vi "Demo_Main-Administrator.vi"() -> ()   [LabVIEW 2010]
uses:
  ControlCAN/ControlCAN.llb/DevType.ctl
  ControlCAN/ControlCAN.llb/CAN Channel.ctl
  ControlCAN/ControlCAN.llb/InitFlag.ctl
  ControlCAN/ControlCAN.llb/Mode.ctl
  ControlCAN/ControlCAN.llb/Fliter.ctl
  ControlCAN/ControlCAN.llb/VCI_CAN_OBJ.ctl
  ControlCAN/ControlCAN.llb/VCI_INIT_CONFIG.ctl
  ControlCAN/ControlCAN.llb/Return Val.ctl
  ControlCAN/ControlCAN.lvlib
panel:
  in  "下限":dbl format="%#.1f"
  out "零位角":dbl format="%#.6f"
  in  "Zero_R":bool
  in  "Zero_SAVE_W":bool
  in  "ZeroEn_R":bool
  in  "零位En":i8
  out "零位使能":i8
  in  "ZeroEn_W":bool
  in  "设定力矩_R":bool
  in  "设定力矩":dbl format="%#.6f"
  out "设定力矩_回":dbl format="%#.6f"
  in  "设定力矩_W":bool
  in  "PosLimitEn_R":bool
  in  "限位En":i8
  out "限位使能":i8
  in  "PosLimitEn_W":bool
  in  "Servo_Count_R":bool
  in  "伺服频率":u16
  out "伺服频率R":u16
  in  "Servo_Count_W":bool
  in  "Servo_EN_R":bool
  in  "伺服En":i8
  out "伺服使能":i8
  in  "Servo_EN_W":bool
  in  "Gear_R":bool
  in  "Kt_R":bool
  in  "Gear":u16
  out "Gear":dbl format="%#.6f"
  in  "Gear_W":bool
  in  "Kt":dbl format="%#.6f"
  out "Kt回":dbl format="%.4f"
  in  "Kt_W":bool
  in  "下限位R":bool
  out "下限位":dbl format="%#.6f"
  in  "下限位_W":bool
  in  "上限位_R":bool
  in  "上限位":dbl format="%#.6f"
  out "上限位 _回":dbl format="%#.6f"
  in  "上限位W":bool
  out "电压限制_回":dbl
  in  "电压限制_R":bool
  in  "电压限制_W":bool
  in  "电压限制":dbl
  in  "位置环KI_R":bool
  in  "位置环KP_R":bool
  in  "位置环KI":dbl format="%#.6f"
  out "位置环KI_回":dbl format="%#.6f"
  in  "位置环KI_W":bool
  in  "位置环KP":dbl format="%#.6f"
  out "位置环KP_回":dbl format="%#.6f"
  in  "位置环KP_W":bool
  in  "T4":u16
  in  "W4":u16
  in  "W3":u16
  out "W4":u16
  in  "W4_R":bool
  in  "W4_W":bool
  in  "W3_R":bool
  out "W3":u16
  in  "W3_W":bool
  out "W2":u16
  in  "W2_R":bool
  in  "W2_W":bool
  in  "W2":u16
  in  "W1_R":bool
  in  "W1":u16
  out "W1":u16
  in  "W1_W":bool
  in  "T4_R":bool
  out "T4":u16
  in  "T4_W":bool
  out "T3":u16
  out "T2":u16
  in  "T3_R":bool
  in  "T2_R":bool
  in  "T3_W":bool
  in  "T2_W":bool
  in  "T3":u16
  in  "T2":u16
  in  "T1_R":bool
  in  "T1":u16
  out "T1":u16
  in  "T1_W":bool
  in  "W_EN_R":bool
  in  "过载诊断":i8
  out "功率使能":i8
  in  "W_EN_W":bool
  in  "I_EN_R":bool
  in  "Direction_R":bool
  in  "电流诊断":i8
  out "电流使能":i8
  in  "I_EN_W":bool
  in  "方向":u16
  out "方向":i8
  in  "Direction_W":bool
  out "电流限制_回":dbl
  in  "电流限制_R":bool
  in  "电流限制_W":bool
  in  "电流限制":dbl
  in  "速度限制_R":bool
  in  "速度限制":dbl
  out "速度限制_回":dbl
  in  "速度限制_W":bool
  out "编码器线数_回":u16
  in  "编码器线数_R":bool
  in  "编码器线数_W":bool
  in  "线数":u16
  in  "极对数_R":bool
  in  "极对数":u8
  out "极对数_回":u8
  in  "极对数_W":bool
  in  "电机自动校准":string(combo)="0"
  in  "电机校准_W":bool
  in  "对准角_R":bool
  in  "对准角":dbl format="%#.6f"
  out "对准角_回":dbl format="%#.6f"
  in  "对准角_W":bool
  in  "减速度_R":bool
  in  "减速度":dbl format="%#.6f"
  out "减速度_回":dbl format="%#.6f"
  in  "减速度_W":bool
  out "版本号":dbl format="%_3f"
  in  "看门狗周期_R":bool
  in  "看门狗周期":u16
  out "看门狗周期_回":u16
  in  "看门狗周期_W":bool
  in  "看门狗_W":bool
  in  "看门狗":string(combo)="开启"
  in  "监测周期_R":bool
  in  "监测周期":u16
  out "监测周期_回":u16
  in  "监测周期_W":bool
  out "ERRO7":bool
  out "ERRO6":bool
  out "ERRO5":bool
  out "ERRO4":bool
  out "ERRO3":bool
  out "高温":bool
  out "高压":bool
  out "低压":bool
  out "warn7":bool
  out "warn6":bool
  out "warn5":bool
  out "warn4":bool
  out "warn3":bool
  out "高温":bool
  out "warn1":bool
  out "warn0":bool
  out "温度":dbl format="%#.6f"
  out "转速":dbl(graph)
  out "CAN ID":u8 format="%x"
  out "数组":u8[](array[numeric]) format="%x"
  in  "DATA_SAVE_W":bool
  out "CI_K0_回":u16
  out "BI_K0_回":u16
  in  "CI_K0_R":bool
  in  "BI_K0_R":bool
  in  "CI_K0_W":bool
  in  "BI_K0_W":bool
  in  "C电流零偏":u16
  in  "B电流零偏":u16
  in  "AI_K0_R":bool
  in  "A电流零偏":u16
  out "AI_K0_回":u16
  in  "AI_K0_W":bool
  out "Sin":i32
  out "Cosin":i32
  in  "加速度_R":bool
  in  "加速度":dbl format="%#.6f"
  out "加速度_回":dbl format="%#.6f"
  in  "加速度_W":bool
  in  "速度环KI_R":bool
  in  "速度环KP_R":bool
  in  "速度环KI":dbl format="%#.6f"
  out "速度环KI_回":dbl format="%#.6f"
  in  "速度环KI_W":bool
  in  "速度环KP":dbl format="%#.6f"
  out "速度环KP_回":dbl format="%#.6f"
  in  "速度环KP_W":bool
  in  "电流环KI_R":bool
  in  "电流环KP_R":bool
  in  "电流环KI":dbl format="%#.6f"
  out "电流环KI_回":dbl format="%#.6f"
  in  "电流环KI_W":bool
  in  "电流环KP":dbl format="%#.6f"
  out "电流环KP_回":dbl format="%#.6f"
  in  "电流环KP_W":bool
  out "波形图表3":dbl(graph)
  out "波形图表2":dbl(graph)
  out "波形图表1":dbl(graph)
  out "sCnt":u32 caption="处理统计"
  out "模式_回":string(combo)="00"
  in  "模式_R":bool
  in  "设定电流_R":bool
  in  "设定位置_R":bool
  in  "设定速度_R":bool
  in  "存储路径":path
  in  "保存":bool
  out "保存_S":bool
  in  "模式_W":bool
  in  "模式":string(combo)="00"
  in  "设定电流":dbl format="%#.6f"
  out "设定电流_回":dbl format="%#.6f"
  in  "设定电流_W":bool
  in  "设定位置":dbl format="%#.6f"
  out "设定位置_回":dbl format="%#.6f"
  in  "设定位置_W":bool
  in  "设定速度":dbl format="%#.1f"
  out "设定速度_回":dbl format="%#.6f"
  in  "设定速度_W":bool
  in  "监测_W":bool
  in  "监测":string(combo)="30"
  out "电机ID_R":u32
  in  "Clear":bool
  out "Ualfa":dbl format="%#.6f"
  out "Ubate":dbl format="%#.6f"
  out "Uq":dbl format="%#.6f"
  out "Ud":dbl format="%#.6f"
  out "PWM1":u16
  out "PWM2":u16
  out "PWM3":u16
  out "sector":u8
  out "Iqnow":dbl
  out "Idnow":dbl
  out "Ialfa":dbl
  out "Ibeta":dbl
  out "A电流":dbl
  out "C电流":dbl
  out "B电流":dbl
  out "供电电压":dbl
  out "机械角度":dbl format="%.2f"
  out "电气角度":dbl format="%.2f"
  out "转速":dbl
  out "CAN STD_ID":u32 format="%x"
  in  "电机ID":string(combo)="00"
  in  "电机ID_W":bool
  out "RecvCnt":u32 caption="接收统计"
  out "SendCnt":u32 caption="发送统计"
  in  "Format":u8(ring) items=["标准帧", "扩展帧"]
  in  "Type":u8(ring) items=["数据帧", "远程帧"]
  in  "Data":string="00 01 02 03 04 05 06 07"
  in  "ID":u32=291 format="0x%x"
  in  "Send":bool
  in  "RcvEnable":bool=TRUE
  out "Open":bool
  in  "Fliter":T1=1 items=["接收所有类型"=1, "只接收标准帧"=2, "只接收扩展帧"=3]
  in  "kBaudRate":u8(ring)=12 caption="波特率" items=["5k bps"=1, "10k bps"=2, "20k bps"=3, "40k bps"=4, "50k bps"=5, "80k bps"=6, "100k bps"=7, "125k bps"=8, "200k bps"=9, "250k bps"=10, "400k bps"=11, "500k bps"=12, "666k bps"=13, "800k bps"=14, "1000k bps"=15, "33.33k bps"=16, "66.66k bps"=17, "83.33k bps"=18]
  in  "Mode":T2 caption="工作模式" items=["正常工作", "仅侦听模式", "自测模式（环回）"]
  in  "InitFlag":T3 caption="初始化参数" items=["使用Flash参数", "使用界面设置参数"]
  in  "AccMask":u32=4294967295 caption="接收屏蔽码" format="%08x"
  in  "AccCode":u32 caption="接收过滤码" format="%08x"
  in  "Close":bool
  in  "Open":bool
  in  "Channel":T4 caption="CAN通道" items=["通道1", "通道2"]
  in  "DevType":T5=3 caption="设备类型" items=["USB-CAN"=2, "USB-CAN2"=3]
  # "发送指令帧包"
  # "CAN\n  ID"
  # "DATA"
  # "DATA"
  # "DATA"
  # "0"
  # "1"
  # "7"
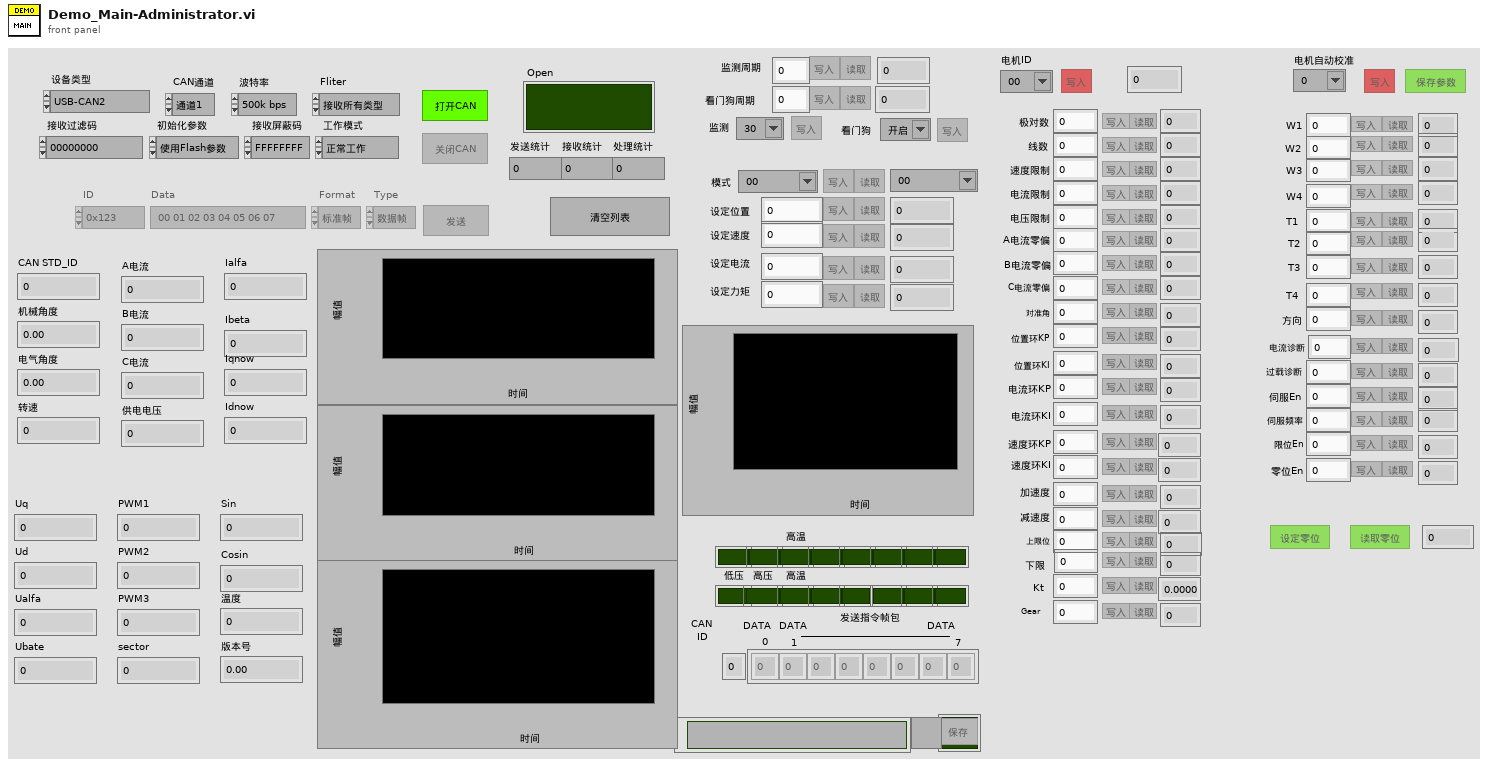
[diagram p1: front panel]
types:
  T1 = typedef "ControlCAN.lvlib/Fliter.ctl" = u8
  T2 = typedef "ControlCAN.lvlib/Mode.ctl" = u8
  T3 = typedef "ControlCAN.lvlib/InitFlag.ctl" = u32
  T4 = typedef "ControlCAN.lvlib/CAN Channel.ctl" = u32
  T5 = typedef "ControlCAN.lvlib/DevType.ctl" = u32
  T6 = typedef "ControlCAN.lvlib/VCI_CAN_OBJ.ctl" = cluster{"ID":u32, "TimeStamp":u32, "TimeFlag":u8, "SendType":u8, "RemoteFlag":u8, "ExternFlag":u8, "DataLen":u8, "Data":u8[], "Reserved":u8[]}
  T7 = cluster{"Type":enum16{"接收", "发送"}, "Channel":T4, "Time":timestamp, "VCI_CAN_OBJ":T6}[]
  T8 = typedef "ControlCAN.lvlib/VCI_INIT_CONFIG.ctl" = cluster{"AccCode":u32, "AccMask":u32, "InitFlag":T3, "Fliter":T1, "Timing0":u8, "Timing1":u8, "Mode":T2}
  T9 = cluster{"DevType":T5, "DevIndex":u32, "CanIndex":T4, "VCI_INIT_CONFIG":T8}
  T10 = typedef "ControlCAN.lvlib/Return Val.ctl" = i32
  T11 = enum16{"open", "replace", "create", "open or create", "replace or create", "replace or create with confirmation"}
  T12 = cluster{"[0]":cluster{"Type":enum16{"接收", "发送"}, "Channel":T4, "Time":timestamp, "VCI_CAN_OBJ":T6}}
  T13 = cluster{"Type":enum16{"接收", "发送"}, "Channel":T4, "Time":timestamp, "VCI_CAN_OBJ":T6}
  T14 = cluster{"Data[0]":u8, "Data[1]":u8, "Data[2]":u8, "Data[3]":u8, "Data[4]":u8, "Data[5]":u8, "Data[6]":u8, "Data[7]":u8}
  T15 = cluster{"Boolean array[0]":bool, "Boolean array[1]":bool, "Boolean array[2]":bool, "Boolean array[3]":bool, "Boolean array[4]":bool, "Boolean array[5]":bool, "Boolean array[6]":bool, "Boolean array[7]":bool}
  T16 = enum32{"invalid app kind", "Development System", "Run Time System", "Student Edition", "Embedded LabVIEW", "Evaluation", "Custom"}
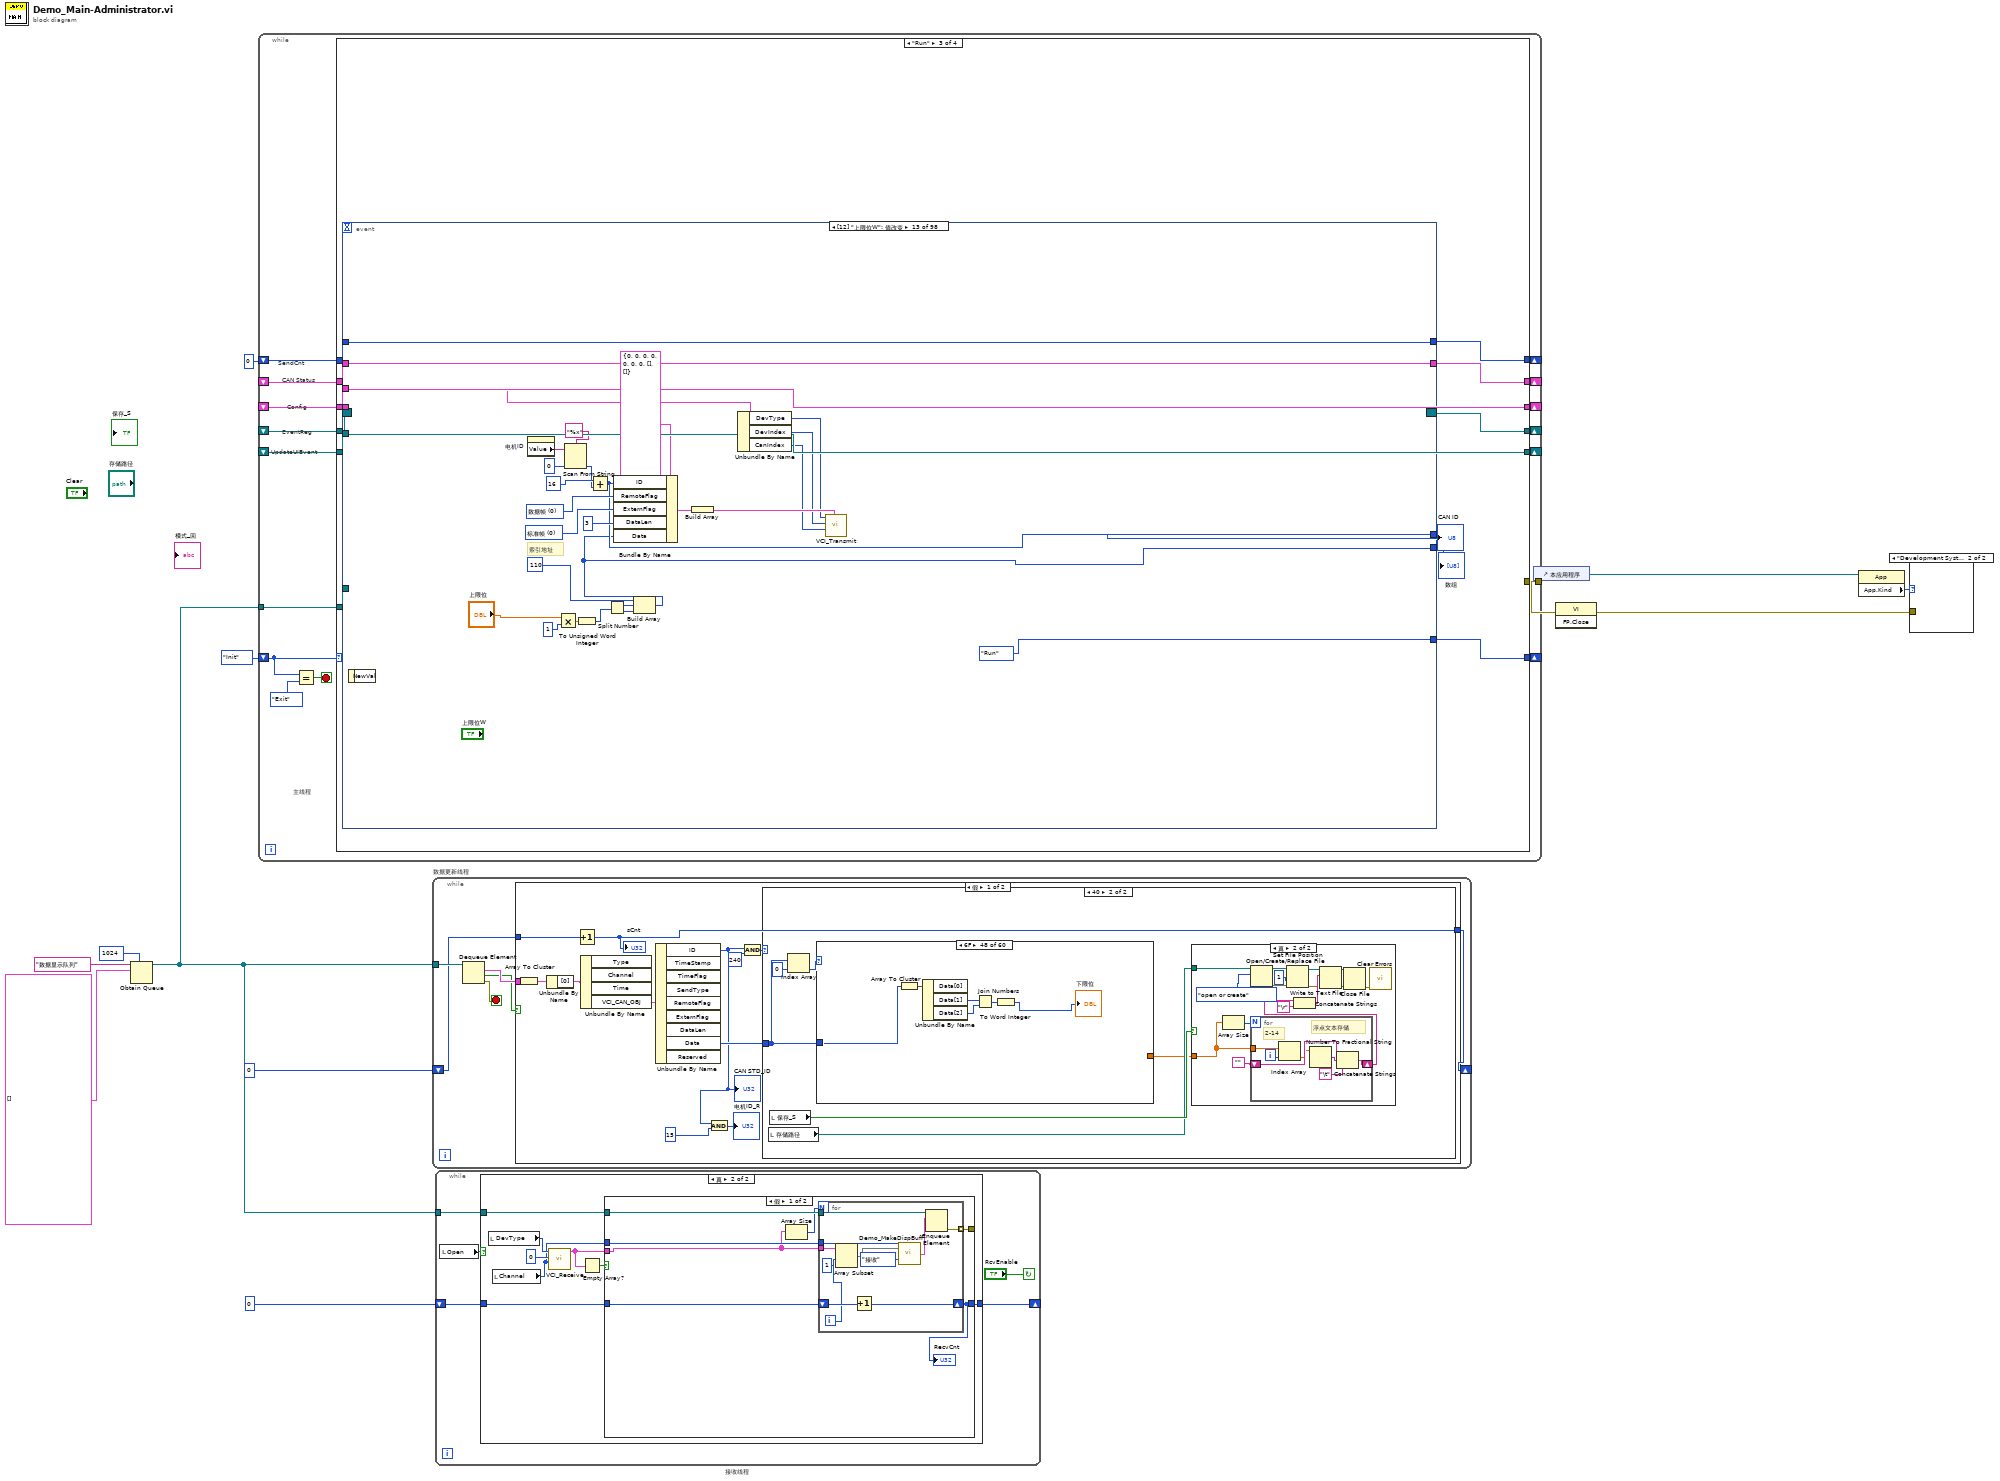
[diagram p0: block diagram]
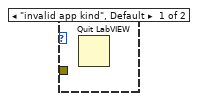
[diagram p2: hidden frame]
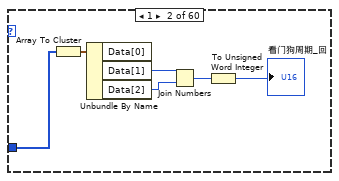
[diagram p6: hidden frame]
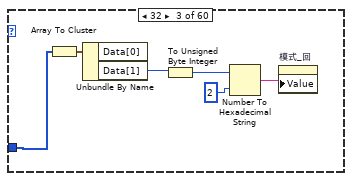
[diagram p7: hidden frame]
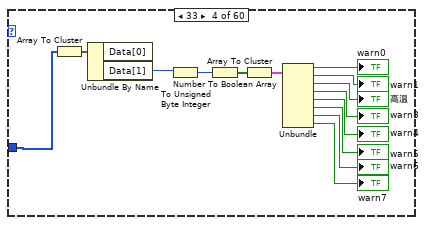
[diagram p8: hidden frame]
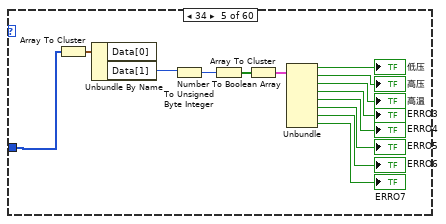
[diagram p9: hidden frame]
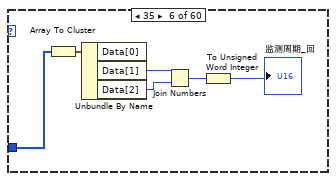
[diagram p10: hidden frame]
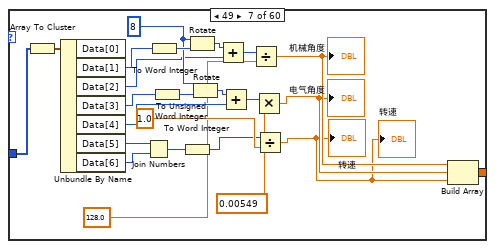
[diagram p11: hidden frame]
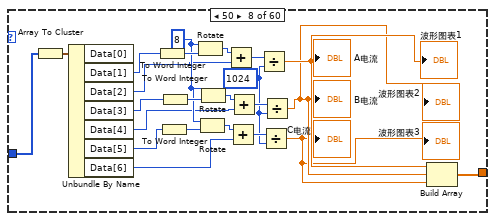
[diagram p12: hidden frame]
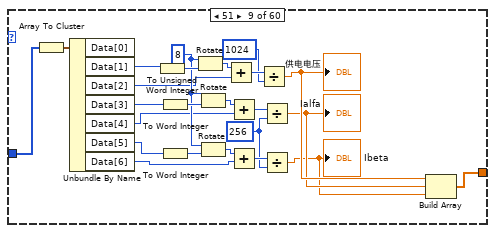
[diagram p13: hidden frame]
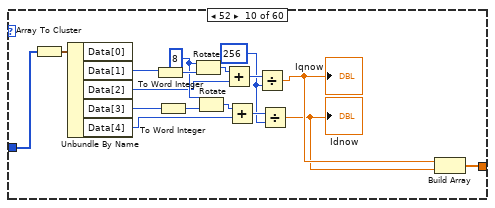
[diagram p14: hidden frame]
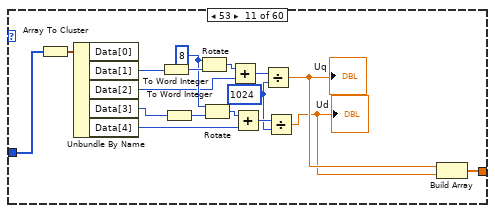
[diagram p15: hidden frame]
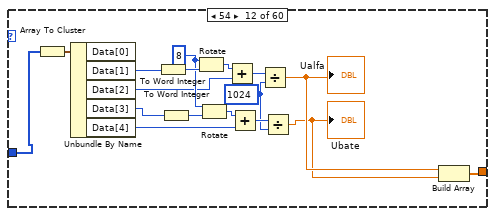
[diagram p16: hidden frame]
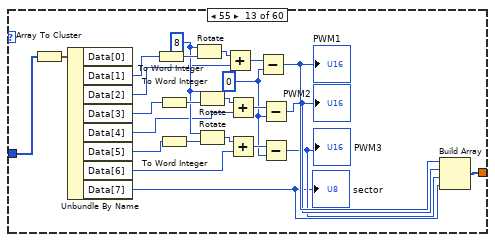
[diagram p17: hidden frame]
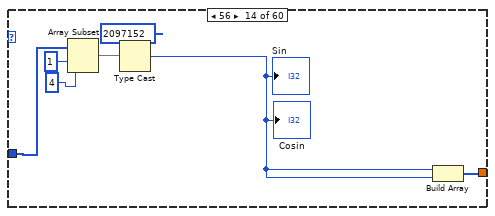
[diagram p18: hidden frame]
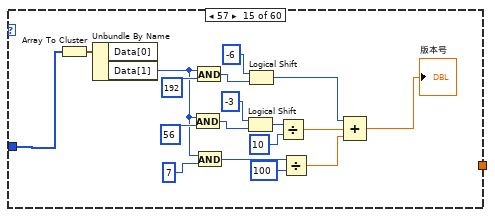
[diagram p19: hidden frame]
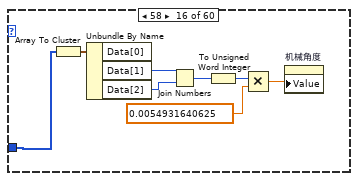
[diagram p20: hidden frame]
diagram:
  n1 = Obtain Queue(max queue size (-1, unlimited)=1024, name (unnamed)="数据显示队列" ("名称（未命名）"), element data type=T7 []) -> (queue out=w9:refnum<queue>)  [unwired: 2 in, 2 out]
  n2 = while "主线程" {
    shift-right: [w24] -> _
    shift-left: enum16{"Init", "Wait", "Run", "Exit"}."Init" -> [w27]
    shift-right: [w25] -> _
    shift-left: _ -> [w26]
    shift-right: [w23] -> _
    shift-left: _ -> [w22]
    tunnel: w9 -> [w21]
    shift-right: [w19] -> _
    shift-left: _ -> [w18]
    shift-right: [w17] -> _
    shift-left: _ -> [w16]
    shift-right: [w14] -> _
    shift-left: u32 0 -> [w15]
    tunnel: [w13] -> w4
    stop <- w28 stop-if-true
    # "CAN Status"
    # "Config"
    # "EventReg"
    # "UpdateUIEvent"
    # "SendCnt"
    n3 = Equal?(x=w27, y=enum16{"Init", "Wait", "Run", "Exit"}."Exit") -> (x = y?=w28:bool)
    n4 = case shown="\"Run\"" w27 {
      tunnel: w26 -> [_ w57 w158 w2353]
      tunnel: [w48 w56 w157 w2353] -> w25
      tunnel: [enum16{"Init", "Wait", "Run", "Exit"}."Wait" w53 w160 enum16{"Init", "Wait", "Run", "Exit"}."Exit"] -> w24
      tunnel: [w44 w54 w149 w2351] -> w23
      tunnel: w22 -> [_ w55 w149 w2351]
      tunnel: w21 -> [_ w52 w159 w2357]
      tunnel: [w36 w51 w155 w2356] -> w19
      tunnel: w18 -> [_ w51 w156 w2356]
      tunnel: [w35 w50 w154 w2354] -> w17
      tunnel: w16 -> [_ w50 w154 w2354]
      tunnel: w15 -> [w33 w49 w153 w2349]
      tunnel: [w33 w49 w152 w2349] -> w14
      tunnel: [_ _ _ errorcluster {"status"=FALSE, "code"=0, "source"=""} ("error constant")] -> w13
      frame "Init", Default {
        w37 = cluster{"CANOpen":bool} {"CANOpen"=FALSE}  # UpdateUI
        w47 = T9 {"DevType"=2, "DevIndex"=0, "CanIndex"=0, "VCI_INIT_CONFIG"={"AccCode"=0, "AccMask"=0, "InitFlag"=0, "Fliter"=0, "Timing0"=0, "Timing1"=0, "Mode"=0}}  # Config
        w48 = cluster{"Open":bool, "SendCnt":u32} {"Open"=FALSE, "SendCnt"=0}  # CAN Status
        n5 = property class="VI"("Front Panel.Closeable"=TRUE ("前面板窗口:可关闭")) -> ()  [unwired: 2 in, 2 out]
        n6 = invoke class="VI" method="Default Vals.Reinit All"() -> ()  [unwired: 3 in, 3 out]
        n7 = call "Demo_GetT0T1.vi"("kBaudRate"="kBaudRate") -> ("Timing0"=w30:u8, "Timing1"=w29:u8)
        n8 = Bundle By Name(cluster=w47, "DevType"="DevType", "CanIndex"="Channel", "VCI_INIT_CONFIG.AccCode"="AccCode", "VCI_INIT_CONFIG.AccMask"="AccMask", "VCI_INIT_CONFIG.InitFlag"="InitFlag", "VCI_INIT_CONFIG.Fliter"="Fliter", "VCI_INIT_CONFIG.Timing0"=w30, "VCI_INIT_CONFIG.Timing1"=w29, "VCI_INIT_CONFIG.Mode"="Mode") -> (w44:T9)
        n9 = local write "RcvEnable"(TRUE ("RcvEnable")) -> ()
        n10 = Create User Event(user event datatype=w37) -> (user event=w35:refnum<user-event>)  [unwired: 1 in, 1 out]
        n11 = register-events(w35) -> (reference out=w36:refnum<event-registration>)  [unwired: 2 in, 1 out]
      }
      frame "Wait" {
        n12 = event shown="[1] 前面板关闭？" {
          selector: _ -> [_ _ _ _ _ _ _ _ _ _]
          dyn-events: _ -> [_ _ _ _ _ _ _ _ _ _]
          timeout: _ -> [_ _ _ _ _ _ _ _ _ _]
          tunnel: w57 -> [w61 w101 w111 w116 w121 w126 w131 w136 w143 w148]
          tunnel: [w60 w101 w111 w116 w121 w126 w131 w136 w143 w148] -> w56
          tunnel: w55 -> [w71 w100 w110 w115 w120 w125 w130 w135 w142 w147]
          tunnel: [w71 w100 w109 w113 w118 w123 w128 w133 w141 w145] -> w54
          tunnel: [w62 enum16{"Init", "Wait", "Run", "Exit"}."Exit" enum16{"Init", "Wait", "Run", "Exit"}."Wait" enum16{"Init", "Wait", "Run", "Exit"}."Wait" enum16{"Init", "Wait", "Run", "Exit"}."Wait" enum16{"Init", "Wait", "Run", "Exit"}."Wait" enum16{"Init", "Wait", "Run", "Exit"}."Wait" enum16{"Init", "Wait", "Run", "Exit"}."Wait" enum16{"Init", "Wait", "Run", "Exit"}."Wait" enum16{"Init", "Wait", "Run", "Exit"}."Wait"] -> w53
          tunnel: w52 -> [_ _ _ _ _ _ _ _ _ _]
          tunnel: w50 -> [w59 _ _ _ _ _ _ _ _ _]
          event "Open": Value Change {
            w65 = T10 1 items=["OK"=1, "ERROR1"=0, "ERROR2"=-1] ("y")
            # "打开CAN的步骤：\n1.Open\n2.Init\n3.Start"
            n13 = event-data() -> ()  [unwired: 2 out]
            n14 = Unbundle By Name(w71) -> ("DevType"=w70:T5, "DevIndex"=w69:u32)
            n15 = call "VCI_OpenDevice.vi"("DevIndex"=w69, "DevType"=w70) -> ("error out"=w66:errorcluster, "Return Val"=w68:T10)  [unwired: 2 in, 6 out]
            n16 = Equal?(x=w68, y=w65) -> (x = y?=w67:bool)
            n17 = case shown="真" w67 {
              tunnel: w66 -> [_ w86]
              tunnel: w71 -> [_ w85]
              tunnel: w65 -> [_ w77]
              tunnel: [_ w76] -> w58
              frame False {
              }
              frame True {
                n18 = Unbundle By Name(w85) -> ("VCI_INIT_CONFIG"=w84:T8, "DevType"=w80:T5, "DevIndex"=w79:u32, "CanIndex"=w78:T4)
                n19 = call "VCI_InitCAN.vi"("VCI_INIT_CONFIG"=w84, "error in (no error)"=w86, "CANIndex"=w78, "DevIndex"=w79, "DevType"=w80) -> ("error out"=w81:errorcluster, "Return Val"=w83:T10)  [unwired: 5 out]
                n20 = Equal?(x=w77, y=w83) -> (x = y?=w82:bool)
                n21 = case shown="真" w82 {
                  tunnel: w81 -> [_ w97]
                  tunnel: w80 -> [_ w96]
                  tunnel: w79 -> [_ w95]
                  tunnel: w78 -> [_ w94]
                  tunnel: w77 -> [_ w92]
                  tunnel: [_ w88] -> w76
                  frame False {
                  }
                  frame True {
                    n22 = call "VCI_StartCAN.vi"("error in (no error)"=w97, "CANIndex"=w94, "DevIndex"=w95, "DevType"=w96) -> ("error out"=w90:errorcluster, "Return Val"=w93:T10)  [unwired: 6 out]
                    n23 = Unbundle By Name(w90) -> ("status"=w87:bool)
                    n24 = Equal?(x=w92, y=w93) -> (x = y?=w91:bool)
                    n25 = Not(x=w87) -> (.not. x?=w89:bool)
                    n26 = And(x=w91, y=w89) -> (x .and. y?=w88:bool)
                  }
                }
              }
            }
            n27 = case shown="真" w58 {
              tunnel: w59 -> [_ w75]
              tunnel: w58 -> [_ w73]
              frame False {
              }
              frame True {
                n28 = Bundle By Name(cluster=cluster{"CANOpen":bool} {"CANOpen"=FALSE} ("事件数据"), "CANOpen"=w73) -> (w72:cluster{"CANOpen":bool})
                n29 = Generate User Event(user event=w75, event data cluster=w72) -> ()  [unwired: 1 in, 2 out]
              }
            }
            n30 = Select(t=enum16{"Init", "Wait", "Run", "Exit"}."Run", s=w58, f=enum16{"Init", "Wait", "Run", "Exit"}."Wait") -> (s? t:f=w62:enum16{"Init", "Wait", "Run", "Exit"})
            n31 = Bundle By Name(cluster=w61, "Open"=w58) -> (w60:cluster{"Open":bool, "SendCnt":u32})
          }
          event Panel Close? {
            n32 = event-data() -> ()  [unwired: 2 out]
            n33 = event-data("Discard?"=TRUE ("放弃？")) -> ()  [unwired: 1 in, 1 out]
          }
          event Value Change {
            w107 = T5 3 items=["USB-CAN"=2, "USB-CAN2"=3] ("y")
            n34 = event-data() -> ("NewVal"=w108:T5)  [unwired: 1 out]
            n35 = Equal?(x=w108, y=w107) -> (x = y?=w106:bool)
            n36 = Bundle By Name(cluster=w110, "DevType"=w108) -> (w109:T9)
            n37 = Select(t=i32[] [] ("禁用项[]"), s=w106, f=i32[] [1] ("禁用项[]")) -> (s? t:f=w105:i32[])
            n38 = property on="Channel" class="Ring (严格)"("Disabled Items []"=w105) -> ()  [unwired: 2 in, 2 out]
          }
          event Value Change {
            n39 = event-data() -> ("NewVal"=w114:T4)  [unwired: 1 out]
            n40 = Bundle By Name(cluster=w115, "CanIndex"=w114) -> (w113:T9)
          }
          event "AccCode": Value Change {
            n41 = event-data() -> ("NewVal"=w119:u32)  [unwired: 1 out]
            n42 = Bundle By Name(cluster=w120, "VCI_INIT_CONFIG.AccCode"=w119) -> (w118:T9)
          }
          event "AccMask": Value Change {
            n43 = event-data() -> ("NewVal"=w124:u32)  [unwired: 1 out]
            n44 = Bundle By Name(cluster=w125, "VCI_INIT_CONFIG.AccMask"=w124) -> (w123:T9)
          }
          event Value Change {
            n45 = event-data() -> ("NewVal"=w129:T3)  [unwired: 1 out]
            n46 = Bundle By Name(cluster=w130, "VCI_INIT_CONFIG.InitFlag"=w129) -> (w128:T9)
          }
          event Value Change {
            n47 = event-data() -> ("NewVal"=w134:T2)  [unwired: 1 out]
            n48 = Bundle By Name(cluster=w135, "VCI_INIT_CONFIG.Mode"=w134) -> (w133:T9)
          }
          event "kBaudRate": Value Change {
            n49 = event-data() -> ("NewVal"=w139:u8)  [unwired: 1 out]
            n50 = call "Demo_GetT0T1.vi"("kBaudRate"=w139) -> ("Timing0"=w138:u8, "Timing1"=w137:u8)
            n51 = Bundle By Name(cluster=w142, "VCI_INIT_CONFIG.Timing0"=w138, "VCI_INIT_CONFIG.Timing1"=w137) -> (w141:T9)
          }
          event Value Change {
            n52 = event-data() -> ("NewVal"=w146:T1)  [unwired: 1 out]
            n53 = Bundle By Name(cluster=w147, "VCI_INIT_CONFIG.Fliter"=w146) -> (w145:T9)
          }
        }
      }
      frame "Run" {
        n54 = event shown="[12] \"上限位W\": 值改变" {
          selector: w156 -> [_ _ _ _ _ _ _ _ _ _ _ _ _ _ _ _ _ _ _ _ _ _ _ _ _ _ _ _ _ _ _ _ _ _ _ _ _ _ _ _ _ _ _ _ _ _ _ _ _ _ _ _ _ _ _ _ _ _ _ _ _ _ _ _ _ _ _ _ _ _ _ _ _ _ _ _ _ _ _ _ _ _ _ _ _ _ _ _ _ _ _ _ _ _ _ _ _ _]
          dyn-events: [_ _ _ _ _ _ _ _ _ _ _ _ _ _ _ _ _ _ _ _ _ _ _ _ _ _ _ _ _ _ _ _ _ _ _ _ _ _ _ _ _ _ _ _ _ _ _ _ _ _ _ _ _ _ _ _ _ _ _ _ _ _ _ _ _ _ _ _ _ _ _ _ _ _ _ _ _ _ _ _ _ _ _ _ _ _ _ _ _ _ _ _ _ _ _ _ _ _] -> w155
          timeout: _ -> [_ _ _ _ _ _ _ _ _ _ _ _ _ _ _ _ _ _ _ _ _ _ _ _ _ _ _ _ _ _ _ _ _ _ _ _ _ _ _ _ _ _ _ _ _ _ _ _ _ _ _ _ _ _ _ _ _ _ _ _ _ _ _ _ _ _ _ _ _ _ _ _ _ _ _ _ _ _ _ _ _ _ _ _ _ _ _ _ _ _ _ _ _ _ _ _ _ _]
          tunnel: [enum16{"Init", "Wait", "Run", "Exit"}."Run" enum16{"Init", "Wait", "Run", "Exit"}."Run" enum16{"Init", "Wait", "Run", "Exit"}."Run" enum16{"Init", "Wait", "Run", "Exit"}."Run" enum16{"Init", "Wait", "Run", "Exit"}."Run" enum16{"Init", "Wait", "Run", "Exit"}."Run" enum16{"Init", "Wait", "Run", "Exit"}."Run" enum16{"Init", "Wait", "Run", "Exit"}."Run" enum16{"Init", "Wait", "Run", "Exit"}."Run" enum16{"Init", "Wait", "Run", "Exit"}."Run" enum16{"Init", "Wait", "Run", "Exit"}."Run" enum16{"Init", "Wait", "Run", "Exit"}."Run" enum16{"Init", "Wait", "Run", "Exit"}."Run" enum16{"Init", "Wait", "Run", "Exit"}."Run" enum16{"Init", "Wait", "Run", "Exit"}."Run" enum16{"Init", "Wait", "Run", "Exit"}."Run" enum16{"Init", "Wait", "Run", "Exit"}."Run" enum16{"Init", "Wait", "Run", "Exit"}."Run" enum16{"Init", "Wait", "Run", "Exit"}."Run" enum16{"Init", "Wait", "Run", "Exit"}."Run" enum16{"Init", "Wait", "Run", "Exit"}."Run" enum16{"Init", "Wait", "Run", "Exit"}."Run" enum16{"Init", "Wait", "Run", "Exit"}."Run" enum16{"Init", "Wait", "Run", "Exit"}."Run" enum16{"Init", "Wait", "Run", "Exit"}."Run" enum16{"Init", "Wait", "Run", "Exit"}."Run" enum16{"Init", "Wait", "Run", "Exit"}."Run" enum16{"Init", "Wait", "Run", "Exit"}."Run" enum16{"Init", "Wait", "Run", "Exit"}."Run" enum16{"Init", "Wait", "Run", "Exit"}."Run" enum16{"Init", "Wait", "Run", "Exit"}."Run" enum16{"Init", "Wait", "Run", "Exit"}."Run" enum16{"Init", "Wait", "Run", "Exit"}."Run" enum16{"Init", "Wait", "Run", "Exit"}."Run" enum16{"Init", "Wait", "Run", "Exit"}."Run" enum16{"Init", "Wait", "Run", "Exit"}."Run" enum16{"Init", "Wait", "Run", "Exit"}."Run" enum16{"Init", "Wait", "Run", "Exit"}."Run" enum16{"Init", "Wait", "Run", "Exit"}."Run" enum16{"Init", "Wait", "Run", "Exit"}."Run" enum16{"Init", "Wait", "Run", "Exit"}."Run" enum16{"Init", "Wait", "Run", "Exit"}."Run" enum16{"Init", "Wait", "Run", "Exit"}."Run" enum16{"Init", "Wait", "Run", "Exit"}."Run" enum16{"Init", "Wait", "Run", "Exit"}."Run" enum16{"Init", "Wait", "Run", "Exit"}."Run" enum16{"Init", "Wait", "Run", "Exit"}."Run" enum16{"Init", "Wait", "Run", "Exit"}."Run" enum16{"Init", "Wait", "Run", "Exit"}."Run" enum16{"Init", "Wait", "Run", "Exit"}."Run" enum16{"Init", "Wait", "Run", "Exit"}."Run" enum16{"Init", "Wait", "Run", "Exit"}."Run" enum16{"Init", "Wait", "Run", "Exit"}."Run" w1354 enum16{"Init", "Wait", "Run", "Exit"}."Run" enum16{"Init", "Wait", "Run", "Exit"}."Run" enum16{"Init", "Wait", "Run", "Exit"}."Run" enum16{"Init", "Wait", "Run", "Exit"}."Run" enum16{"Init", "Wait", "Run", "Exit"}."Run" enum16{"Init", "Wait", "Run", "Exit"}."Run" enum16{"Init", "Wait", "Run", "Exit"}."Run" enum16{"Init", "Wait", "Run", "Exit"}."Run" enum16{"Init", "Wait", "Run", "Exit"}."Run" enum16{"Init", "Wait", "Run", "Exit"}."Run" enum16{"Init", "Wait", "Run", "Exit"}."Run" enum16{"Init", "Wait", "Run", "Exit"}."Run" enum16{"Init", "Wait", "Run", "Exit"}."Run" enum16{"Init", "Wait", "Run", "Exit"}."Run" enum16{"Init", "Wait", "Run", "Exit"}."Run" enum16{"Init", "Wait", "Run", "Exit"}."Run" enum16{"Init", "Wait", "Run", "Exit"}."Run" enum16{"Init", "Wait", "Run", "Exit"}."Run" enum16{"Init", "Wait", "Run", "Exit"}."Run" enum16{"Init", "Wait", "Run", "Exit"}."Run" enum16{"Init", "Wait", "Run", "Exit"}."Run" enum16{"Init", "Wait", "Run", "Exit"}."Run" enum16{"Init", "Wait", "Run", "Exit"}."Run" enum16{"Init", "Wait", "Run", "Exit"}."Run" enum16{"Init", "Wait", "Run", "Exit"}."Run" enum16{"Init", "Wait", "Run", "Exit"}."Run" enum16{"Init", "Wait", "Run", "Exit"}."Run" enum16{"Init", "Wait", "Run", "Exit"}."Run" enum16{"Init", "Wait", "Run", "Exit"}."Run" enum16{"Init", "Wait", "Run", "Exit"}."Run" enum16{"Init", "Wait", "Run", "Exit"}."Run" enum16{"Init", "Wait", "Run", "Exit"}."Run" enum16{"Init", "Wait", "Run", "Exit"}."Run" enum16{"Init", "Wait", "Run", "Exit"}."Run" enum16{"Init", "Wait", "Run", "Exit"}."Run" enum16{"Init", "Wait", "Run", "Exit"}."Run" enum16{"Init", "Wait", "Run", "Exit"}."Run" enum16{"Init", "Wait", "Run", "Exit"}."Run" enum16{"Init", "Wait", "Run", "Exit"}."Run" enum16{"Init", "Wait", "Run", "Exit"}."Run" enum16{"Init", "Wait", "Run", "Exit"}."Run" enum16{"Init", "Wait", "Run", "Exit"}."Run" enum16{"Init", "Wait", "Run", "Exit"}."Run" enum16{"Init", "Wait", "Run", "Exit"}."Run"] -> w160
          tunnel: w159 -> [_ _ _ _ _ _ _ _ _ _ _ _ _ _ _ _ _ _ _ _ _ _ _ _ _ _ _ _ _ _ _ _ _ _ _ _ _ _ _ _ _ _ _ _ _ _ _ _ _ _ _ _ _ _ _ _ _ _ _ _ _ _ _ _ _ _ _ _ _ _ _ _ _ _ _ _ _ _ _ _ _ _ _ _ _ _ _ _ _ _ _ _ _ _ _ _ _ _]
          tunnel: [w162 w179 w196 w219 w241 w262 w286 w307 w334 w355 w382 w403 w430 w454 w475 w496 w515 w536 w552 w590 w611 w637 w663 w689 w715 w736 w762 w788 w814 w840 w866 w892 w916 w940 w964 w991 w1012 w1033 w1054 w1075 w1096 w1117 w1138 w1159 w1180 w1201 w1222 w1243 w1264 w1285 w1306 w1334 w1340 w1359 w1383 w1407 w1428 w1452 w1473 w1497 w1518 w1539 w1560 w1584 w1608 w1629 w1653 w1674 w1698 w1719 w1741 w1762 w1784 w1805 w1827 w1848 w1874 w1895 w1921 w1942 w1969 w1990 w2011 w2037 w2058 w2084 w2106 w2127 w2148 w2174 w2195 w2219 w2240 w2262 w2283 w2305 w2326 w2347] -> w157
          tunnel: w158 -> [w162 w179 w196 w219 w241 w262 w286 w307 w334 w355 w382 w403 w430 w454 w475 w496 w515 w536 w552 w590 w611 w637 w663 w689 w715 w736 w762 w788 w814 w840 w866 w892 w916 w940 w964 w991 w1012 w1033 w1054 w1075 w1096 w1117 w1138 w1159 w1180 w1201 w1222 w1243 w1264 w1285 w1306 w1334 w1342 w1359 w1383 w1407 w1428 w1452 w1473 w1497 w1518 w1539 w1560 w1584 w1608 w1629 w1653 w1674 w1698 w1719 w1741 w1762 w1784 w1805 w1827 w1848 w1874 w1895 w1921 w1942 w1969 w1990 w2011 w2037 w2058 w2084 w2106 w2127 w2148 w2174 w2195 w2219 w2240 w2262 w2283 w2305 w2326 w2347]
          tunnel: w149 -> [_ w174 w186 w201 w224 w245 w267 w290 w315 w338 w360 w386 w405 w435 w458 w485 w501 w519 w542 w572 w594 w622 w645 w671 w694 w719 w741 w767 w793 w819 w845 w871 w897 w921 w945 w972 w995 w1021 w1037 w1058 w1079 w1100 w1121 w1142 w1163 w1184 w1205 w1226 w1247 w1268 w1289 _ w1347 _ w1360 w1388 w1411 w1432 w1453 w1478 w1501 w1519 w1540 w1563 w1589 w1612 w1634 w1654 w1679 w1702 w1721 w1742 w1767 w1788 w1807 w1828 w1853 w1878 w1900 w1925 w1947 w1971 w1994 w2021 w2038 w2063 _ _ w2131 w2151 w2178 _ _ _ w2266 w2288 w2309 w2330]
          tunnel: w154 -> [_ _ _ _ _ _ _ _ _ _ _ _ _ _ _ _ _ _ _ _ _ _ _ _ _ _ _ _ _ _ _ _ _ _ _ _ _ _ _ _ _ _ _ _ _ _ _ _ _ _ _ _ w1339 _ _ _ _ _ _ _ _ _ _ _ _ _ _ _ _ _ _ _ _ _ _ _ _ _ _ _ _ _ _ _ _ _ _ _ _ _ _ _ _ _ _ _ _ _]
          tunnel: w153 -> [w161 w167 w195 w218 w240 w261 w285 w306 w333 w354 w381 w402 w429 w453 w474 w495 w514 w535 w551 w589 w610 w636 w662 w688 w714 w735 w761 w787 w813 w839 w865 w891 w915 w939 w963 w990 w1011 w1032 w1053 w1074 w1095 w1116 w1137 w1158 w1179 w1200 w1221 w1242 w1263 w1284 w1305 w1333 w1335 w1353 w1382 w1406 w1427 w1451 w1472 w1496 w1517 w1538 w1559 w1583 w1607 w1628 w1652 w1673 w1697 w1718 w1740 w1761 w1783 w1804 w1826 w1847 w1873 w1894 w1920 w1941 w1968 w1989 w2010 w2036 w2057 w2083 w2105 w2126 w2147 w2173 w2194 w2218 w2239 w2261 w2282 w2304 w2325 w2346]
          tunnel: [w161 w166 w195 w218 w240 w261 w285 w306 w333 w354 w381 w402 w429 w453 w474 w495 w514 w535 w551 w589 w610 w636 w662 w688 w714 w735 w761 w787 w813 w839 w865 w891 w915 w939 w963 w990 w1011 w1032 w1053 w1074 w1095 w1116 w1137 w1158 w1179 w1200 w1221 w1242 w1263 w1284 w1305 w1333 w1335 w1353 w1382 w1406 w1427 w1451 w1472 w1496 w1517 w1538 w1559 w1583 w1607 w1628 w1652 w1673 w1697 w1718 w1740 w1761 w1783 w1804 w1826 w1847 w1873 w1894 w1920 w1941 w1968 w1989 w2010 w2036 w2057 w2083 w2105 w2126 w2147 w2173 w2194 w2218 w2239 w2261 w2282 w2304 w2325 w2346] -> w152
          tunnel: [_ _ w182 w199 w222 w243 w264 w288 w313 w336 w358 w384 w407 w433 w456 w477 w499 w517 w538 w570 w592 w613 w639 w665 w691 w717 w738 w764 w790 w816 w842 w869 w894 w918 w942 w970 w993 w1020 w1035 w1056 w1077 w1098 w1119 w1140 w1161 w1182 w1203 w1224 w1245 w1266 w1287 _ _ _ w1363 w1387 w1409 w1430 w1454 w1476 w1499 w1521 w1541 w1564 w1587 w1610 w1632 w1655 w1676 w1699 w1723 w1743 w1765 w1786 w1809 w1829 w1851 w1876 w1898 w1923 w1945 w1972 w1992 w2015 w2040 w2061 w2087 w2108 w2129 w2152 w2176 w2198 w2222 w2243 w2264 w2286 w2306 w2328] -> w151
          tunnel: [_ _ w181 w200 w223 w244 w265 w289 w314 w337 w359 w385 w408 w434 w457 w476 w500 w518 w541 w569 w591 w612 w638 w664 w692 w718 w737 w763 w789 w815 w841 w868 w893 w917 w941 w971 w992 w1014 w1034 w1055 w1076 w1097 w1118 w1139 w1160 w1181 w1204 w1223 w1244 w1265 w1288 _ _ _ w1364 w1386 w1410 w1431 w1455 w1477 w1500 w1522 w1542 w1565 w1588 w1611 w1633 w1656 w1677 w1700 w1724 w1744 w1766 w1787 w1810 w1830 w1852 w1877 w1899 w1924 w1946 w1973 w1993 w2020 w2041 w2062 w2088 w2109 w2130 w2153 w2177 w2199 w2223 w2244 w2265 w2287 w2307 w2329] -> w150
          tunnel: w149 -> [_ _ _ _ _ _ _ _ _ _ _ _ _ _ _ _ _ _ _ _ _ _ _ _ _ _ _ _ _ _ _ _ _ _ _ _ _ _ _ _ _ _ _ _ _ _ _ _ _ _ _ _ _ _ _ _ _ _ _ _ _ _ _ _ _ _ _ _ _ _ _ _ _ _ _ _ _ _ _ _ _ _ _ _ _ _ w2089 w2110 _ _ _ w2200 w2220 w2245 _ _ _ _]
          event Timeout {
            n55 = event-data() -> ()  [unwired: 3 out]
          }
          event "Send": Value Change {
            n56 = event-data() -> ()  [unwired: 2 out]
            n57 = Increment(x=w167) -> (x+1=w166:u32)
            "SendCnt" <- w166
            n58 = call "Demo_MakeData.vi"("DataString"="Data") -> ("Data"=w169:u8[], "DataLen"=w170:u8)  [unwired: 9 out]
            n59 = Bundle By Name(cluster=T6 {"ID"=0, "TimeStamp"=0, "TimeFlag"=0, "SendType"=0, "RemoteFlag"=0, "ExternFlag"=0, "DataLen"=0, "Data"=[], "Reserved"=[]} ("Send"), "ID"="ID", "RemoteFlag"="Type", "ExternFlag"="Format", "DataLen"=w170, "Data"=w169) -> (w164:T6)
            n60 = Build Array(w164) -> (w165:T6[])
            n61 = Unbundle By Name(w174) -> ("DevType"=w173:T5, "DevIndex"=w172:u32, "CanIndex"=w168:T4)
            n62 = call "VCI_Transmit.vi"("Buffer"=w165, "CANIndex"=w168, "DevIndex"=w172, "DevType"=w173) -> ()  [unwired: 1 in, 7 out]
          }
          event "电机ID_W": Value Change {
            w185 = u8 0 items=["数据帧", "遥控帧"]
            w181 = u32 138
            w184 = u8 0 items=["标准帧", "扩展帧"]
            n63 = event-data() -> ()  [unwired: 2 out]
            n64 = call "Demo_MakeData.vi"("DataString"="电机ID") -> ("Data"=w182:u8[], "DataLen"=w190:u8)  [unwired: 9 out]
            n65 = Bundle By Name(cluster=T6 {"ID"=0, "TimeStamp"=0, "TimeFlag"=0, "SendType"=0, "RemoteFlag"=0, "ExternFlag"=0, "DataLen"=0, "Data"=[], "Reserved"=[]} ("Send"), "ID"=w181, "RemoteFlag"=w185, "ExternFlag"=w184, "DataLen"=w190, "Data"=w182) -> (w187:T6)
            n66 = Build Array(w187) -> (w188:T6[])
            n67 = Unbundle By Name(w186) -> ("DevType"=w192:T5, "DevIndex"=w191:u32, "CanIndex"=w189:T4)
            n68 = call "VCI_Transmit.vi"("Buffer"=w188, "CANIndex"=w189, "DevIndex"=w191, "DevType"=w192) -> ()  [unwired: 1 in, 7 out]
          }
          event "电机校准_W": Value Change {
            w216 = u8 0 items=["数据帧", "遥控帧"]
            w217 = u8 0 items=["标准帧", "扩展帧"]
            # "地址"
            n69 = event-data() -> ()  [unwired: 2 out]
            n70 = property on="电机ID" class="CmbBox"() -> ("Value"=w207:string)  [unwired: 2 in, 2 out]
            n71 = Concatenate Strings("20 ", "AA 01 02 03 04 05 55") -> (w203:string)
            n72 = Scan From String(format string="%x" ("格式字符串"), input string=w207, default 1=u8 0) -> (output 1=w204:u8)  [unwired: 2 in, 3 out]
            n73 = call "Demo_MakeData.vi"("DataString"=w203) -> ("Data"=w199:u8[], "DataLen"=w212:u8)  [unwired: 9 out]
            n74 = Add(x=u32 16, y=w204) -> (x+y=w200:u32)
            n75 = Bundle By Name(cluster=T6 {"ID"=0, "TimeStamp"=0, "TimeFlag"=0, "SendType"=0, "RemoteFlag"=0, "ExternFlag"=0, "DataLen"=0, "Data"=[], "Reserved"=[]} ("Send"), "ID"=w200, "RemoteFlag"=w216, "ExternFlag"=w217, "DataLen"=w212, "Data"=w199) -> (w215:T6)
            n76 = Build Array(w215) -> (w214:T6[])
            n77 = Unbundle By Name(w201) -> ("DevType"=w210:T5, "DevIndex"=w211:u32, "CanIndex"=w213:T4)
            n78 = call "VCI_Transmit.vi"("Buffer"=w214, "CANIndex"=w213, "DevIndex"=w211, "DevType"=w210) -> ()  [unwired: 1 in, 7 out]
          }
          event "极对数_W": Value Change {
            w236 = u8 0 items=["数据帧", "遥控帧"]
            w237 = u8 0 items=["标准帧", "扩展帧"]
            # "索引地址"
            n79 = event-data() -> ()  [unwired: 2 out]
            n80 = property on="电机ID" class="CmbBox"() -> ("Value"=w228:string)  [unwired: 2 in, 2 out]
            n81 = Scan From String(format string="%x" ("格式字符串"), input string=w228, default 1=u8 0) -> (output 1=w225:u8)  [unwired: 2 in, 3 out]
            n82 = Add(x=u32 16, y=w225) -> (x+y=w223:u32)
            n83 = Build Array(u8 94, "极对数") -> (w222:u8[])
            n84 = Bundle By Name(cluster=T6 {"ID"=0, "TimeStamp"=0, "TimeFlag"=0, "SendType"=0, "RemoteFlag"=0, "ExternFlag"=0, "DataLen"=0, "Data"=[], "Reserved"=[]} ("Send"), "ID"=w223, "RemoteFlag"=w236, "ExternFlag"=w237, "DataLen"=u8 2, "Data"=w222) -> (w235:T6)
            n85 = Build Array(w235) -> (w234:T6[])
            n86 = Unbundle By Name(w224) -> ("DevType"=w231:T5, "DevIndex"=w232:u32, "CanIndex"=w233:T4)
            n87 = call "VCI_Transmit.vi"("Buffer"=w234, "CANIndex"=w233, "DevIndex"=w232, "DevType"=w231) -> ()  [unwired: 1 in, 7 out]
          }
          event "极对数_R": Value Change {
            w248 = u8 0 items=["数据帧", "遥控帧"]
            w247 = u8 0 items=["标准帧", "扩展帧"]
            # "地址"
            n88 = event-data() -> ()  [unwired: 2 out]
            n89 = property on="电机ID" class="CmbBox"() -> ("Value"=w257:string)  [unwired: 2 in, 2 out]
            n90 = Scan From String(format string="%x" ("格式字符串"), input string=w257, default 1=u8 0) -> (output 1=w260:u8)  [unwired: 2 in, 3 out]
            n91 = call "Demo_MakeData.vi"("DataString"="5E") -> ("Data"=w243:u8[], "DataLen"=w252:u8)  [unwired: 9 out]
            n92 = Add(x=u32 48, y=w260) -> (x+y=w244:u32)
            n93 = Bundle By Name(cluster=T6 {"ID"=0, "TimeStamp"=0, "TimeFlag"=0, "SendType"=0, "RemoteFlag"=0, "ExternFlag"=0, "DataLen"=0, "Data"=[], "Reserved"=[]} ("Send"), "ID"=w244, "RemoteFlag"=w248, "ExternFlag"=w247, "DataLen"=w252, "Data"=w243) -> (w249:T6)
            n94 = Build Array(w249) -> (w250:T6[])
            n95 = Unbundle By Name(w245) -> ("DevType"=w254:T5, "DevIndex"=w253:u32, "CanIndex"=w251:T4)
            n96 = call "VCI_Transmit.vi"("Buffer"=w250, "CANIndex"=w251, "DevIndex"=w253, "DevType"=w254) -> ()  [unwired: 1 in, 7 out]
          }
          event "编码器线数_W": Value Change {
            w279 = u8 0 items=["数据帧", "遥控帧"]
            w280 = u8 0 items=["标准帧", "扩展帧"]
            # "索引地址"
            n97 = event-data() -> ()  [unwired: 2 out]
            n98 = property on="电机ID" class="CmbBox"() -> ("Value"=w271:string)  [unwired: 2 in, 2 out]
            n99 = Scan From String(format string="%x" ("格式字符串"), input string=w271, default 1=u8 0) -> (output 1=w268:u8)  [unwired: 2 in, 3 out]
            n100 = Split Number(x="线数") -> (hi(x)=w283:u8, lo(x)=w284:u8)
            n101 = Add(x=u32 16, y=w268) -> (x+y=w265:u32)
            n102 = Build Array(u8 95, w283, w284) -> (w264:u8[])
            n103 = Bundle By Name(cluster=T6 {"ID"=0, "TimeStamp"=0, "TimeFlag"=0, "SendType"=0, "RemoteFlag"=0, "ExternFlag"=0, "DataLen"=0, "Data"=[], "Reserved"=[]} ("Send"), "ID"=w265, "RemoteFlag"=w279, "ExternFlag"=w280, "DataLen"=u8 3, "Data"=w264) -> (w278:T6)
            n104 = Build Array(w278) -> (w277:T6[])
            n105 = Unbundle By Name(w267) -> ("DevType"=w274:T5, "DevIndex"=w275:u32, "CanIndex"=w276:T4)
            n106 = call "VCI_Transmit.vi"("Buffer"=w277, "CANIndex"=w276, "DevIndex"=w275, "DevType"=w274) -> ()  [unwired: 1 in, 7 out]
          }
          event "编码器线数_R": Value Change {
            w293 = u8 0 items=["数据帧", "遥控帧"]
            w292 = u8 0 items=["标准帧", "扩展帧"]
            # "地址"
            n107 = event-data() -> ()  [unwired: 2 out]
            n108 = property on="电机ID" class="CmbBox"() -> ("Value"=w302:string)  [unwired: 2 in, 2 out]
            n109 = Scan From String(format string="%x" ("格式字符串"), input string=w302, default 1=u8 0) -> (output 1=w305:u8)  [unwired: 2 in, 3 out]
            n110 = call "Demo_MakeData.vi"("DataString"="5F ") -> ("Data"=w288:u8[], "DataLen"=w297:u8)  [unwired: 9 out]
            n111 = Add(x=u32 48, y=w305) -> (x+y=w289:u32)
            n112 = Bundle By Name(cluster=T6 {"ID"=0, "TimeStamp"=0, "TimeFlag"=0, "SendType"=0, "RemoteFlag"=0, "ExternFlag"=0, "DataLen"=0, "Data"=[], "Reserved"=[]} ("Send"), "ID"=w289, "RemoteFlag"=w293, "ExternFlag"=w292, "DataLen"=w297, "Data"=w288) -> (w294:T6)
            n113 = Build Array(w294) -> (w295:T6[])
            n114 = Unbundle By Name(w290) -> ("DevType"=w299:T5, "DevIndex"=w298:u32, "CanIndex"=w296:T4)
            n115 = call "VCI_Transmit.vi"("Buffer"=w295, "CANIndex"=w296, "DevIndex"=w298, "DevType"=w299) -> ()  [unwired: 1 in, 7 out]
          }
          event "速度限制_W": Value Change {
            w319 = u8 0 items=["数据帧", "遥控帧"]
            w318 = u8 0 items=["标准帧", "扩展帧"]
            # "索引地址"
            n116 = event-data() -> ()  [unwired: 2 out]
            n117 = property on="电机ID" class="CmbBox"() -> ("Value"=w327:string)  [unwired: 2 in, 2 out]
            n118 = Multiply ("乘")(x="速度限制", y=i16 1) -> (x*y=w311:i16)
            n119 = Scan From String(format string="%x" ("格式字符串"), input string=w327, default 1=u8 0) -> (output 1=w330:u8)  [unwired: 2 in, 3 out]
            n120 = Absolute Value(x=w311) -> (abs(x)=w308:i16)
            n121 = Add(x=u32 16, y=w330) -> (x+y=w314:u32)
            n122 = Split Number(x=w308) -> (hi(x)=w331:u8, lo(x)=w332:u8)
            n123 = Build Array(u8 88, w331, w332) -> (w313:u8[])
            n124 = Bundle By Name(cluster=T6 {"ID"=0, "TimeStamp"=0, "TimeFlag"=0, "SendType"=0, "RemoteFlag"=0, "ExternFlag"=0, "DataLen"=0, "Data"=[], "Reserved"=[]} ("Send"), "ID"=w314, "RemoteFlag"=w319, "ExternFlag"=w318, "DataLen"=u8 3, "Data"=w313) -> (w320:T6)
            n125 = Build Array(w320) -> (w321:T6[])
            n126 = Unbundle By Name(w315) -> ("DevType"=w324:T5, "DevIndex"=w323:u32, "CanIndex"=w322:T4)
            n127 = call "VCI_Transmit.vi"("Buffer"=w321, "CANIndex"=w322, "DevIndex"=w323, "DevType"=w324) -> ()  [unwired: 1 in, 7 out]
          }
          event "速度限制_R": Value Change {
            w341 = u8 0 items=["数据帧", "遥控帧"]
            w340 = u8 0 items=["标准帧", "扩展帧"]
            # "地址"
            n128 = event-data() -> ()  [unwired: 2 out]
            n129 = property on="电机ID" class="CmbBox"() -> ("Value"=w350:string)  [unwired: 2 in, 2 out]
            n130 = Scan From String(format string="%x" ("格式字符串"), input string=w350, default 1=u8 0) -> (output 1=w353:u8)  [unwired: 2 in, 3 out]
            n131 = call "Demo_MakeData.vi"("DataString"="58") -> ("Data"=w336:u8[], "DataLen"=w345:u8)  [unwired: 9 out]
            n132 = Add(x=u32 48, y=w353) -> (x+y=w337:u32)
            n133 = Bundle By Name(cluster=T6 {"ID"=0, "TimeStamp"=0, "TimeFlag"=0, "SendType"=0, "RemoteFlag"=0, "ExternFlag"=0, "DataLen"=0, "Data"=[], "Reserved"=[]} ("Send"), "ID"=w337, "RemoteFlag"=w341, "ExternFlag"=w340, "DataLen"=w345, "Data"=w336) -> (w342:T6)
            n134 = Build Array(w342) -> (w343:T6[])
            n135 = Unbundle By Name(w338) -> ("DevType"=w347:T5, "DevIndex"=w346:u32, "CanIndex"=w344:T4)
            n136 = call "VCI_Transmit.vi"("Buffer"=w343, "CANIndex"=w344, "DevIndex"=w346, "DevType"=w347) -> ()  [unwired: 1 in, 7 out]
          }
          event "电流限制_W": Value Change {
            w374 = u8 0 items=["数据帧", "遥控帧"]
            w375 = u8 0 items=["标准帧", "扩展帧"]
            # "索引地址"
            n137 = event-data() -> ()  [unwired: 2 out]
            n138 = property on="电机ID" class="CmbBox"() -> ("Value"=w366:string)  [unwired: 2 in, 2 out]
            n139 = Multiply ("乘")(x="电流限制", y=i16 8) -> (x*y=w378:i16)
            n140 = Scan From String(format string="%x" ("格式字符串"), input string=w366, default 1=u8 0) -> (output 1=w363:u8)  [unwired: 2 in, 3 out]
            n141 = Absolute Value(x=w378) -> (abs(x)=w380:i16)
            n142 = Add(x=u32 16, y=w363) -> (x+y=w359:u32)
            n143 = Split Number(x=w380) -> (hi(x)=w362:u8, lo(x)=w361:u8)
            n144 = Build Array(u8 87, w362, w361) -> (w358:u8[])
            n145 = Bundle By Name(cluster=T6 {"ID"=0, "TimeStamp"=0, "TimeFlag"=0, "SendType"=0, "RemoteFlag"=0, "ExternFlag"=0, "DataLen"=0, "Data"=[], "Reserved"=[]} ("Send"), "ID"=w359, "RemoteFlag"=w374, "ExternFlag"=w375, "DataLen"=u8 3, "Data"=w358) -> (w373:T6)
            n146 = Build Array(w373) -> (w372:T6[])
            n147 = Unbundle By Name(w360) -> ("DevType"=w369:T5, "DevIndex"=w370:u32, "CanIndex"=w371:T4)
            n148 = call "VCI_Transmit.vi"("Buffer"=w372, "CANIndex"=w371, "DevIndex"=w370, "DevType"=w369) -> ()  [unwired: 1 in, 7 out]
          }
          event "电流限制_R": Value Change {
            w389 = u8 0 items=["数据帧", "遥控帧"]
            w388 = u8 0 items=["标准帧", "扩展帧"]
            # "地址"
            n149 = event-data() -> ()  [unwired: 2 out]
            n150 = property on="电机ID" class="CmbBox"() -> ("Value"=w398:string)  [unwired: 2 in, 2 out]
            n151 = Scan From String(format string="%x" ("格式字符串"), input string=w398, default 1=u8 0) -> (output 1=w401:u8)  [unwired: 2 in, 3 out]
            n152 = call "Demo_MakeData.vi"("DataString"="57 ") -> ("Data"=w384:u8[], "DataLen"=w393:u8)  [unwired: 9 out]
            n153 = Add(x=u32 48, y=w401) -> (x+y=w385:u32)
            n154 = Bundle By Name(cluster=T6 {"ID"=0, "TimeStamp"=0, "TimeFlag"=0, "SendType"=0, "RemoteFlag"=0, "ExternFlag"=0, "DataLen"=0, "Data"=[], "Reserved"=[]} ("Send"), "ID"=w385, "RemoteFlag"=w389, "ExternFlag"=w388, "DataLen"=w393, "Data"=w384) -> (w390:T6)
            n155 = Build Array(w390) -> (w391:T6[])
            n156 = Unbundle By Name(w386) -> ("DevType"=w395:T5, "DevIndex"=w394:u32, "CanIndex"=w392:T4)
            n157 = call "VCI_Transmit.vi"("Buffer"=w391, "CANIndex"=w392, "DevIndex"=w394, "DevType"=w395) -> ()  [unwired: 1 in, 7 out]
          }
          event "上限位W": Value Change {
            w423 = u8 0 items=["数据帧", "遥控帧"]
            w424 = u8 0 items=["标准帧", "扩展帧"]
            # "索引地址"
            n158 = event-data() -> ()  [unwired: 2 out]
            n159 = property on="电机ID" class="CmbBox"() -> ("Value"=w415:string)  [unwired: 2 in, 2 out]
            n160 = Multiply(x="上限位", y=u16 1) -> (x*y=w410:dbl)
            n161 = Scan From String(format string="%x" ("格式字符串"), input string=w415, default 1=u8 0) -> (output 1=w412:u8)  [unwired: 2 in, 3 out]
            n162 = To Unsigned Word Integer(number=w410) -> (unsigned 16bit integer=w409:u16)
            n163 = Add(x=u32 16, y=w412) -> (x+y=w408:u32)
            n164 = Split Number(x=w409) -> (hi(x)=w427:u8, lo(x)=w428:u8)
            n165 = Build Array(u8 110, w427, w428) -> (w407:u8[])
            n166 = Bundle By Name(cluster=T6 {"ID"=0, "TimeStamp"=0, "TimeFlag"=0, "SendType"=0, "RemoteFlag"=0, "ExternFlag"=0, "DataLen"=0, "Data"=[], "Reserved"=[]} ("Send"), "ID"=w408, "RemoteFlag"=w423, "ExternFlag"=w424, "DataLen"=u8 3, "Data"=w407) -> (w422:T6)
            n167 = Build Array(w422) -> (w421:T6[])
            n168 = Unbundle By Name(w405) -> ("DevType"=w418:T5, "DevIndex"=w419:u32, "CanIndex"=w420:T4)
            n169 = call "VCI_Transmit.vi"("Buffer"=w421, "CANIndex"=w420, "DevIndex"=w419, "DevType"=w418) -> ()  [unwired: 1 in, 7 out]
          }
          event "监测周期_W": Value Change {
            w447 = u8 0 items=["数据帧", "遥控帧"]
            w448 = u8 0 items=["标准帧", "扩展帧"]
            # "索引地址"
            n170 = event-data() -> ()  [unwired: 2 out]
            n171 = property on="电机ID" class="CmbBox"() -> ("Value"=w439:string)  [unwired: 2 in, 2 out]
            n172 = Scan From String(format string="%x" ("格式字符串"), input string=w439, default 1=u8 0) -> (output 1=w436:u8)  [unwired: 2 in, 3 out]
            n173 = Split Number(x="监测周期") -> (hi(x)=w451:u8, lo(x)=w452:u8)
            n174 = Add(x=u32 16, y=w436) -> (x+y=w434:u32)
            n175 = Build Array(u8 35, w451, w452) -> (w433:u8[])
            n176 = Bundle By Name(cluster=T6 {"ID"=0, "TimeStamp"=0, "TimeFlag"=0, "SendType"=0, "RemoteFlag"=0, "ExternFlag"=0, "DataLen"=0, "Data"=[], "Reserved"=[]} ("Send"), "ID"=w434, "RemoteFlag"=w447, "ExternFlag"=w448, "DataLen"=u8 3, "Data"=w433) -> (w446:T6)
            n177 = Build Array(w446) -> (w445:T6[])
            n178 = Unbundle By Name(w435) -> ("DevType"=w442:T5, "DevIndex"=w443:u32, "CanIndex"=w444:T4)
            n179 = call "VCI_Transmit.vi"("Buffer"=w445, "CANIndex"=w444, "DevIndex"=w443, "DevType"=w442) -> ()  [unwired: 1 in, 7 out]
          }
          event "监测周期_R": Value Change {
            w471 = u8 0 items=["数据帧", "遥控帧"]
            w472 = u8 0 items=["标准帧", "扩展帧"]
            # "地址"
            n180 = event-data() -> ()  [unwired: 2 out]
            n181 = property on="电机ID" class="CmbBox"() -> ("Value"=w462:string)  [unwired: 2 in, 2 out]
            n182 = Scan From String(format string="%x" ("格式字符串"), input string=w462, default 1=u8 0) -> (output 1=w459:u8)  [unwired: 2 in, 3 out]
            n183 = call "Demo_MakeData.vi"("DataString"="23 ") -> ("Data"=w456:u8[], "DataLen"=w467:u8)  [unwired: 9 out]
            n184 = Add(x=u32 48, y=w459) -> (x+y=w457:u32)
            n185 = Bundle By Name(cluster=T6 {"ID"=0, "TimeStamp"=0, "TimeFlag"=0, "SendType"=0, "RemoteFlag"=0, "ExternFlag"=0, "DataLen"=0, "Data"=[], "Reserved"=[]} ("Send"), "ID"=w457, "RemoteFlag"=w471, "ExternFlag"=w472, "DataLen"=w467, "Data"=w456) -> (w470:T6)
            n186 = Build Array(w470) -> (w469:T6[])
            n187 = Unbundle By Name(w458) -> ("DevType"=w465:T5, "DevIndex"=w466:u32, "CanIndex"=w468:T4)
            n188 = call "VCI_Transmit.vi"("Buffer"=w469, "CANIndex"=w468, "DevIndex"=w466, "DevType"=w465) -> ()  [unwired: 1 in, 7 out]
          }
          event "监测_W": Value Change {
            w493 = u8 0 items=["数据帧", "遥控帧"]
            w494 = u8 0 items=["标准帧", "扩展帧"]
            # "地址"
            n189 = event-data() -> ()  [unwired: 2 out]
            n190 = property on="电机ID" class="CmbBox"() -> ("Value"=w482:string)  [unwired: 2 in, 2 out]
            n191 = Scan From String(format string="%x" ("格式字符串"), input string=w482, default 1=u8 0) -> (output 1=w479:u8)  [unwired: 2 in, 3 out]
            n192 = call "Demo_MakeData.vi"("DataString"="监测") -> ("Data"=w477:u8[], "DataLen"=w489:u8)  [unwired: 9 out]
            n193 = Add(x=u32 48, y=w479) -> (x+y=w476:u32)
            n194 = Bundle By Name(cluster=T6 {"ID"=0, "TimeStamp"=0, "TimeFlag"=0, "SendType"=0, "RemoteFlag"=0, "ExternFlag"=0, "DataLen"=0, "Data"=[], "Reserved"=[]} ("Send"), "ID"=w476, "RemoteFlag"=w493, "ExternFlag"=w494, "DataLen"=w489, "Data"=w477) -> (w492:T6)
            n195 = Build Array(w492) -> (w491:T6[])
            n196 = Unbundle By Name(w485) -> ("DevType"=w487:T5, "DevIndex"=w488:u32, "CanIndex"=w490:T4)
            n197 = call "VCI_Transmit.vi"("Buffer"=w491, "CANIndex"=w490, "DevIndex"=w488, "DevType"=w487) -> ()  [unwired: 1 in, 7 out]
          }
          event "看门狗周期_W": Value Change {
            w507 = u8 0 items=["数据帧", "遥控帧"]
            w506 = u8 0 items=["标准帧", "扩展帧"]
            w500 = u32 138
            # "索引地址"
            n198 = event-data() -> ()  [unwired: 2 out]
            n199 = Split Number(x="看门狗周期") -> (hi(x)=w503:u8, lo(x)=w502:u8)
            n200 = Build Array(u8 1, w503, w502) -> (w499:u8[])
            n201 = Bundle By Name(cluster=T6 {"ID"=0, "TimeStamp"=0, "TimeFlag"=0, "SendType"=0, "RemoteFlag"=0, "ExternFlag"=0, "DataLen"=0, "Data"=[], "Reserved"=[]} ("Send"), "ID"=w500, "RemoteFlag"=w507, "ExternFlag"=w506, "DataLen"=u8 3, "Data"=w499) -> (w508:T6)
            n202 = Build Array(w508) -> (w509:T6[])
            n203 = Unbundle By Name(w501) -> ("DevType"=w512:T5, "DevIndex"=w511:u32, "CanIndex"=w510:T4)
            n204 = call "VCI_Transmit.vi"("Buffer"=w509, "CANIndex"=w510, "DevIndex"=w511, "DevType"=w512) -> ()  [unwired: 1 in, 7 out]
          }
          event "看门狗周期_R": Value Change {
            w522 = u8 0 items=["数据帧", "遥控帧"]
            w521 = u8 0 items=["标准帧", "扩展帧"]
            # "地址"
            n205 = event-data() -> ()  [unwired: 2 out]
            n206 = property on="电机ID" class="CmbBox"() -> ("Value"=w531:string)  [unwired: 2 in, 2 out]
            n207 = Scan From String(format string="%x" ("格式字符串"), input string=w531, default 1=u8 0) -> (output 1=w534:u8)  [unwired: 2 in, 3 out]
            n208 = call "Demo_MakeData.vi"("DataString"="01") -> ("Data"=w517:u8[], "DataLen"=w526:u8)  [unwired: 9 out]
            n209 = Add(x=u32 48, y=w534) -> (x+y=w518:u32)
            n210 = Bundle By Name(cluster=T6 {"ID"=0, "TimeStamp"=0, "TimeFlag"=0, "SendType"=0, "RemoteFlag"=0, "ExternFlag"=0, "DataLen"=0, "Data"=[], "Reserved"=[]} ("Send"), "ID"=w518, "RemoteFlag"=w522, "ExternFlag"=w521, "DataLen"=w526, "Data"=w517) -> (w523:T6)
            n211 = Build Array(w523) -> (w524:T6[])
            n212 = Unbundle By Name(w519) -> ("DevType"=w528:T5, "DevIndex"=w527:u32, "CanIndex"=w525:T4)
            n213 = call "VCI_Transmit.vi"("Buffer"=w524, "CANIndex"=w525, "DevIndex"=w527, "DevType"=w528) -> ()  [unwired: 1 in, 7 out]
          }
          event "看门狗_W": Value Change {
            w549 = u8 0 items=["数据帧", "遥控帧"]
            w541 = u32 138
            w550 = u8 0 items=["标准帧", "扩展帧"]
            n214 = event-data() -> ()  [unwired: 2 out]
            n215 = case shown="\"开启\", 默认" "看门狗" {
              tunnel: [w553 w558 w563] -> w538
              frame "开启", Default {
                n216 = Split Number(x=u16 52428) -> (hi(x)=w556:u8, lo(x)=w557:u8)
                n217 = Build Array(u8 2, w556, w557) -> (w553:u8[])
              }
              frame "喂狗" {
                n218 = Split Number(x=u16 43690) -> (hi(x)=w560:u8, lo(x)=w559:u8)
                n219 = Build Array(u8 2, w560, w559) -> (w558:u8[])
              }
              frame "关闭" {
                n220 = Split Number(x=u16 52394) -> (hi(x)=w565:u8, lo(x)=w564:u8)
                n221 = Build Array(u8 2, w565, w564) -> (w563:u8[])
              }
            }
            n222 = Bundle By Name(cluster=T6 {"ID"=0, "TimeStamp"=0, "TimeFlag"=0, "SendType"=0, "RemoteFlag"=0, "ExternFlag"=0, "DataLen"=0, "Data"=[], "Reserved"=[]} ("Send"), "ID"=w541, "RemoteFlag"=w549, "ExternFlag"=w550, "DataLen"=u8 3, "Data"=w538) -> (w548:T6)
            n223 = Build Array(w548) -> (w547:T6[])
            n224 = Unbundle By Name(w542) -> ("DevType"=w544:T5, "DevIndex"=w545:u32, "CanIndex"=w546:T4)
            n225 = call "VCI_Transmit.vi"("Buffer"=w547, "CANIndex"=w546, "DevIndex"=w545, "DevType"=w544) -> ()  [unwired: 1 in, 7 out]
          }
          event "模式_W": Value Change {
            w574 = u8 0 items=["数据帧", "遥控帧"]
            w573 = u8 0 items=["标准帧", "扩展帧"]
            # "地址"
            n226 = event-data() -> ()  [unwired: 2 out]
            n227 = property on="电机ID" class="CmbBox"() -> ("Value"=w583:string)  [unwired: 2 in, 2 out]
            n228 = Concatenate Strings("20 ", "模式") -> (w587:string)
            n229 = Scan From String(format string="%x" ("格式字符串"), input string=w583, default 1=u8 0) -> (output 1=w586:u8)  [unwired: 2 in, 3 out]
            n230 = property on="模式_回" class="CmbBox"("Value"="模式") -> ()  [unwired: 2 in, 2 out]
            n231 = call "Demo_MakeData.vi"("DataString"=w587) -> ("Data"=w570:u8[], "DataLen"=w578:u8)  [unwired: 9 out]
            n232 = Add(x=u32 16, y=w586) -> (x+y=w569:u32)
            n233 = Bundle By Name(cluster=T6 {"ID"=0, "TimeStamp"=0, "TimeFlag"=0, "SendType"=0, "RemoteFlag"=0, "ExternFlag"=0, "DataLen"=0, "Data"=[], "Reserved"=[]} ("Send"), "ID"=w569, "RemoteFlag"=w574, "ExternFlag"=w573, "DataLen"=w578, "Data"=w570) -> (w575:T6)
            n234 = Build Array(w575) -> (w576:T6[])
            n235 = Unbundle By Name(w572) -> ("DevType"=w580:T5, "DevIndex"=w579:u32, "CanIndex"=w577:T4)
            n236 = call "VCI_Transmit.vi"("Buffer"=w576, "CANIndex"=w577, "DevIndex"=w579, "DevType"=w580) -> ()  [unwired: 1 in, 7 out]
          }
          event "模式_R": Value Change {
            w607 = u8 0 items=["数据帧", "遥控帧"]
            w608 = u8 0 items=["标准帧", "扩展帧"]
            # "地址"
            n237 = event-data() -> ()  [unwired: 2 out]
            n238 = property on="电机ID" class="CmbBox"() -> ("Value"=w598:string)  [unwired: 2 in, 2 out]
            n239 = Scan From String(format string="%x" ("格式字符串"), input string=w598, default 1=u8 0) -> (output 1=w595:u8)  [unwired: 2 in, 3 out]
            n240 = call "Demo_MakeData.vi"("DataString"="20 ") -> ("Data"=w592:u8[], "DataLen"=w603:u8)  [unwired: 9 out]
            n241 = Add(x=u32 48, y=w595) -> (x+y=w591:u32)
            n242 = Bundle By Name(cluster=T6 {"ID"=0, "TimeStamp"=0, "TimeFlag"=0, "SendType"=0, "RemoteFlag"=0, "ExternFlag"=0, "DataLen"=0, "Data"=[], "Reserved"=[]} ("Send"), "ID"=w591, "RemoteFlag"=w607, "ExternFlag"=w608, "DataLen"=w603, "Data"=w592) -> (w606:T6)
            n243 = Build Array(w606) -> (w605:T6[])
            n244 = Unbundle By Name(w594) -> ("DevType"=w601:T5, "DevIndex"=w602:u32, "CanIndex"=w604:T4)
            n245 = call "VCI_Transmit.vi"("Buffer"=w605, "CANIndex"=w604, "DevIndex"=w602, "DevType"=w601) -> ()  [unwired: 1 in, 7 out]
          }
          event "设定位置_W": Value Change {
            w624 = u8 0 items=["数据帧", "遥控帧"]
            w623 = u8 0 items=["标准帧", "扩展帧"]
            # "索引地址"
            n246 = event-data() -> ()  [unwired: 2 out]
            n247 = Multiply ("乘")(x="设定位置", y=u16 128) -> (x*y=w616:i16)
            n248 = property on="电机ID" class="CmbBox"() -> ("Value"=w632:string)  [unwired: 2 in, 2 out]
            n249 = Scan From String(format string="%x" ("格式字符串"), input string=w632, default 1=u8 0) -> (output 1=w635:u8)  [unwired: 2 in, 3 out]
            n250 = Split Number(x=w616) -> (hi(x)=w615:u8, lo(x)=w614:u8)
            n251 = Add(x=u32 16, y=w635) -> (x+y=w612:u32)
            n252 = Build Array(u8 64, w615, w614) -> (w613:u8[])
            n253 = Bundle By Name(cluster=T6 {"ID"=0, "TimeStamp"=0, "TimeFlag"=0, "SendType"=0, "RemoteFlag"=0, "ExternFlag"=0, "DataLen"=0, "Data"=[], "Reserved"=[]} ("Send"), "ID"=w612, "RemoteFlag"=w624, "ExternFlag"=w623, "DataLen"=u8 3, "Data"=w613) -> (w625:T6)
            n254 = Build Array(w625) -> (w626:T6[])
            n255 = Unbundle By Name(w622) -> ("DevType"=w629:T5, "DevIndex"=w628:u32, "CanIndex"=w627:T4)
            n256 = call "VCI_Transmit.vi"("Buffer"=w626, "CANIndex"=w627, "DevIndex"=w628, "DevType"=w629) -> ()  [unwired: 1 in, 7 out]
          }
          event "设定速度_W": Value Change {
            w657 = u8 0 items=["数据帧", "遥控帧"]
            w658 = u8 0 items=["标准帧", "扩展帧"]
            # "索引地址"
            n257 = event-data() -> ()  [unwired: 2 out]
            n258 = property on="电机ID" class="CmbBox"() -> ("Value"=w649:string)  [unwired: 2 in, 2 out]
            n259 = Multiply ("乘")(x="设定速度", y=i16 1) -> (x*y=w642:i16)
            n260 = Scan From String(format string="%x" ("格式字符串"), input string=w649, default 1=u8 0) -> (output 1=w646:u8)  [unwired: 2 in, 3 out]
            n261 = Split Number(x=w642) -> (hi(x)=w641:u8, lo(x)=w640:u8)
            n262 = Add(x=u32 16, y=w646) -> (x+y=w638:u32)
            n263 = Build Array(u8 65, w641, w640) -> (w639:u8[])
            n264 = Bundle By Name(cluster=T6 {"ID"=0, "TimeStamp"=0, "TimeFlag"=0, "SendType"=0, "RemoteFlag"=0, "ExternFlag"=0, "DataLen"=0, "Data"=[], "Reserved"=[]} ("Send"), "ID"=w638, "RemoteFlag"=w657, "ExternFlag"=w658, "DataLen"=u8 3, "Data"=w639) -> (w656:T6)
            n265 = Build Array(w656) -> (w655:T6[])
            n266 = Unbundle By Name(w645) -> ("DevType"=w652:T5, "DevIndex"=w653:u32, "CanIndex"=w654:T4)
            n267 = call "VCI_Transmit.vi"("Buffer"=w655, "CANIndex"=w654, "DevIndex"=w653, "DevType"=w652) -> ()  [unwired: 1 in, 7 out]
          }
          event "设定电流_W": Value Change {
            w676 = u8 0 items=["数据帧", "遥控帧"]
            w675 = u8 0 items=["标准帧", "扩展帧"]
            # "索引地址"
            n268 = event-data() -> ()  [unwired: 2 out]
            n269 = property on="电机ID" class="CmbBox"() -> ("Value"=w684:string)  [unwired: 2 in, 2 out]
            n270 = Multiply ("乘")(x="设定电流", y=i16 256) -> (x*y=w668:i16)
            n271 = Scan From String(format string="%x" ("格式字符串"), input string=w684, default 1=u8 0) -> (output 1=w687:u8)  [unwired: 2 in, 3 out]
            n272 = Split Number(x=w668) -> (hi(x)=w667:u8, lo(x)=w666:u8)
            n273 = Add(x=u32 16, y=w687) -> (x+y=w664:u32)
            n274 = Build Array(u8 66, w667, w666) -> (w665:u8[])
            n275 = Bundle By Name(cluster=T6 {"ID"=0, "TimeStamp"=0, "TimeFlag"=0, "SendType"=0, "RemoteFlag"=0, "ExternFlag"=0, "DataLen"=0, "Data"=[], "Reserved"=[]} ("Send"), "ID"=w664, "RemoteFlag"=w676, "ExternFlag"=w675, "DataLen"=u8 3, "Data"=w665) -> (w677:T6)
            n276 = Build Array(w677) -> (w678:T6[])
            n277 = Unbundle By Name(w671) -> ("DevType"=w681:T5, "DevIndex"=w680:u32, "CanIndex"=w679:T4)
            n278 = call "VCI_Transmit.vi"("Buffer"=w678, "CANIndex"=w679, "DevIndex"=w680, "DevType"=w681) -> ()  [unwired: 1 in, 7 out]
          }
          event "设定力矩_W": Value Change {
            w702 = u8 0 items=["数据帧", "遥控帧"]
            w701 = u8 0 items=["标准帧", "扩展帧"]
            # "索引地址"
            n279 = event-data() -> ()  [unwired: 2 out]
            n280 = property on="电机ID" class="CmbBox"() -> ("Value"=w710:string)  [unwired: 2 in, 2 out]
            n281 = Multiply ("乘")(x="设定力矩", y=i16 256) -> (x*y=w697:i16)
            n282 = Scan From String(format string="%x" ("格式字符串"), input string=w710, default 1=u8 0) -> (output 1=w713:u8)  [unwired: 2 in, 3 out]
            n283 = Split Number(x=w697) -> (hi(x)=w696:u8, lo(x)=w695:u8)
            n284 = Add(x=u32 16, y=w713) -> (x+y=w692:u32)
            n285 = Build Array(u8 67, w696, w695) -> (w691:u8[])
            n286 = Bundle By Name(cluster=T6 {"ID"=0, "TimeStamp"=0, "TimeFlag"=0, "SendType"=0, "RemoteFlag"=0, "ExternFlag"=0, "DataLen"=0, "Data"=[], "Reserved"=[]} ("Send"), "ID"=w692, "RemoteFlag"=w702, "ExternFlag"=w701, "DataLen"=u8 3, "Data"=w691) -> (w703:T6)
            n287 = Build Array(w703) -> (w704:T6[])
            n288 = Unbundle By Name(w694) -> ("DevType"=w707:T5, "DevIndex"=w706:u32, "CanIndex"=w705:T4)
            n289 = call "VCI_Transmit.vi"("Buffer"=w704, "CANIndex"=w705, "DevIndex"=w706, "DevType"=w707) -> ()  [unwired: 1 in, 7 out]
          }
          event "设定力矩_R": Value Change {
            w722 = u8 0 items=["数据帧", "遥控帧"]
            w721 = u8 0 items=["标准帧", "扩展帧"]
            # "地址"
            n290 = event-data() -> ()  [unwired: 2 out]
            n291 = property on="电机ID" class="CmbBox"() -> ("Value"=w731:string)  [unwired: 2 in, 2 out]
            n292 = Scan From String(format string="%x" ("格式字符串"), input string=w731, default 1=u8 0) -> (output 1=w734:u8)  [unwired: 2 in, 3 out]
            n293 = call "Demo_MakeData.vi"("DataString"="43 ") -> ("Data"=w717:u8[], "DataLen"=w726:u8)  [unwired: 9 out]
            n294 = Add(x=u32 48, y=w734) -> (x+y=w718:u32)
            n295 = Bundle By Name(cluster=T6 {"ID"=0, "TimeStamp"=0, "TimeFlag"=0, "SendType"=0, "RemoteFlag"=0, "ExternFlag"=0, "DataLen"=0, "Data"=[], "Reserved"=[]} ("Send"), "ID"=w718, "RemoteFlag"=w722, "ExternFlag"=w721, "DataLen"=w726, "Data"=w717) -> (w723:T6)
            n296 = Build Array(w723) -> (w724:T6[])
            n297 = Unbundle By Name(w719) -> ("DevType"=w728:T5, "DevIndex"=w727:u32, "CanIndex"=w725:T4)
            n298 = call "VCI_Transmit.vi"("Buffer"=w724, "CANIndex"=w725, "DevIndex"=w727, "DevType"=w728) -> ()  [unwired: 1 in, 7 out]
          }
          event "电流环KP_W": Value Change {
            w753 = u8 0 items=["数据帧", "遥控帧"]
            w754 = u8 0 items=["标准帧", "扩展帧"]
            # "索引地址"
            n299 = event-data() -> ()  [unwired: 2 out]
            n300 = property on="电机ID" class="CmbBox"() -> ("Value"=w745:string)  [unwired: 2 in, 2 out]
            n301 = Multiply ("乘")(x="电流环KP", y=u16 256) -> (x*y=w758:u16)
            n302 = Scan From String(format string="%x" ("格式字符串"), input string=w745, default 1=u8 0) -> (output 1=w742:u8)  [unwired: 2 in, 3 out]
            n303 = Split Number(x=w758) -> (hi(x)=w759:u8, lo(x)=w760:u8)
            n304 = Add(x=u32 16, y=w742) -> (x+y=w737:u32)
            n305 = Build Array(u8 81, w759, w760) -> (w738:u8[])
            n306 = Bundle By Name(cluster=T6 {"ID"=0, "TimeStamp"=0, "TimeFlag"=0, "SendType"=0, "RemoteFlag"=0, "ExternFlag"=0, "DataLen"=0, "Data"=[], "Reserved"=[]} ("Send"), "ID"=w737, "RemoteFlag"=w753, "ExternFlag"=w754, "DataLen"=u8 3, "Data"=w738) -> (w752:T6)
            n307 = Build Array(w752) -> (w751:T6[])
            n308 = Unbundle By Name(w741) -> ("DevType"=w748:T5, "DevIndex"=w749:u32, "CanIndex"=w750:T4)
            n309 = call "VCI_Transmit.vi"("Buffer"=w751, "CANIndex"=w750, "DevIndex"=w749, "DevType"=w748) -> ()  [unwired: 1 in, 7 out]
          }
          event "电流环KI_W": Value Change {
            w775 = u8 0 items=["数据帧", "遥控帧"]
            w774 = u8 0 items=["标准帧", "扩展帧"]
            # "索引地址"
            n310 = event-data() -> ()  [unwired: 2 out]
            n311 = property on="电机ID" class="CmbBox"() -> ("Value"=w783:string)  [unwired: 2 in, 2 out]
            n312 = Multiply ("乘")(x="电流环KI", y=u16 256) -> (x*y=w770:u16)
            n313 = Scan From String(format string="%x" ("格式字符串"), input string=w783, default 1=u8 0) -> (output 1=w786:u8)  [unwired: 2 in, 3 out]
            n314 = Split Number(x=w770) -> (hi(x)=w769:u8, lo(x)=w768:u8)
            n315 = Add(x=u32 16, y=w786) -> (x+y=w763:u32)
            n316 = Build Array(u8 82, w769, w768) -> (w764:u8[])
            n317 = Bundle By Name(cluster=T6 {"ID"=0, "TimeStamp"=0, "TimeFlag"=0, "SendType"=0, "RemoteFlag"=0, "ExternFlag"=0, "DataLen"=0, "Data"=[], "Reserved"=[]} ("Send"), "ID"=w763, "RemoteFlag"=w775, "ExternFlag"=w774, "DataLen"=u8 3, "Data"=w764) -> (w776:T6)
            n318 = Build Array(w776) -> (w777:T6[])
            n319 = Unbundle By Name(w767) -> ("DevType"=w780:T5, "DevIndex"=w779:u32, "CanIndex"=w778:T4)
            n320 = call "VCI_Transmit.vi"("Buffer"=w777, "CANIndex"=w778, "DevIndex"=w779, "DevType"=w780) -> ()  [unwired: 1 in, 7 out]
          }
          event "速度环KP_W": Value Change {
            w801 = u8 0 items=["数据帧", "遥控帧"]
            w800 = u8 0 items=["标准帧", "扩展帧"]
            # "索引地址"
            n321 = event-data() -> ()  [unwired: 2 out]
            n322 = property on="电机ID" class="CmbBox"() -> ("Value"=w809:string)  [unwired: 2 in, 2 out]
            n323 = Multiply ("乘")(x="速度环KP", y=u16 256) -> (x*y=w796:u16)
            n324 = Scan From String(format string="%x" ("格式字符串"), input string=w809, default 1=u8 0) -> (output 1=w812:u8)  [unwired: 2 in, 3 out]
            n325 = Split Number(x=w796) -> (hi(x)=w795:u8, lo(x)=w794:u8)
            n326 = Add(x=u32 16, y=w812) -> (x+y=w789:u32)
            n327 = Build Array(u8 83, w795, w794) -> (w790:u8[])
            n328 = Bundle By Name(cluster=T6 {"ID"=0, "TimeStamp"=0, "TimeFlag"=0, "SendType"=0, "RemoteFlag"=0, "ExternFlag"=0, "DataLen"=0, "Data"=[], "Reserved"=[]} ("Send"), "ID"=w789, "RemoteFlag"=w801, "ExternFlag"=w800, "DataLen"=u8 3, "Data"=w790) -> (w802:T6)
            n329 = Build Array(w802) -> (w803:T6[])
            n330 = Unbundle By Name(w793) -> ("DevType"=w806:T5, "DevIndex"=w805:u32, "CanIndex"=w804:T4)
            n331 = call "VCI_Transmit.vi"("Buffer"=w803, "CANIndex"=w804, "DevIndex"=w805, "DevType"=w806) -> ()  [unwired: 1 in, 7 out]
          }
          event "速度环KI_W": Value Change {
            w831 = u8 0 items=["数据帧", "遥控帧"]
            w832 = u8 0 items=["标准帧", "扩展帧"]
            # "索引地址"
            n332 = event-data() -> ()  [unwired: 2 out]
            n333 = property on="电机ID" class="CmbBox"() -> ("Value"=w823:string)  [unwired: 2 in, 2 out]
            n334 = Multiply ("乘")(x="速度环KI", y=u16 256) -> (x*y=w836:u16)
            n335 = Scan From String(format string="%x" ("格式字符串"), input string=w823, default 1=u8 0) -> (output 1=w820:u8)  [unwired: 2 in, 3 out]
            n336 = Split Number(x=w836) -> (hi(x)=w837:u8, lo(x)=w838:u8)
            n337 = Add(x=u32 16, y=w820) -> (x+y=w815:u32)
            n338 = Build Array(u8 84, w837, w838) -> (w816:u8[])
            n339 = Bundle By Name(cluster=T6 {"ID"=0, "TimeStamp"=0, "TimeFlag"=0, "SendType"=0, "RemoteFlag"=0, "ExternFlag"=0, "DataLen"=0, "Data"=[], "Reserved"=[]} ("Send"), "ID"=w815, "RemoteFlag"=w831, "ExternFlag"=w832, "DataLen"=u8 3, "Data"=w816) -> (w830:T6)
            n340 = Build Array(w830) -> (w829:T6[])
            n341 = Unbundle By Name(w819) -> ("DevType"=w826:T5, "DevIndex"=w827:u32, "CanIndex"=w828:T4)
            n342 = call "VCI_Transmit.vi"("Buffer"=w829, "CANIndex"=w828, "DevIndex"=w827, "DevType"=w826) -> ()  [unwired: 1 in, 7 out]
          }
          event "加速度_W": Value Change {
            w853 = u8 0 items=["数据帧", "遥控帧"]
            w852 = u8 0 items=["标准帧", "扩展帧"]
            # "索引地址"
            n343 = event-data() -> ()  [unwired: 2 out]
            n344 = property on="电机ID" class="CmbBox"() -> ("Value"=w861:string)  [unwired: 2 in, 2 out]
            n345 = Multiply ("乘")(x="加速度", y=u16 8) -> (x*y=w848:u16)
            n346 = Scan From String(format string="%x" ("格式字符串"), input string=w861, default 1=u8 0) -> (output 1=w864:u8)  [unwired: 2 in, 3 out]
            n347 = Split Number(x=w848) -> (hi(x)=w847:u8, lo(x)=w846:u8)
            n348 = Add(x=u32 16, y=w864) -> (x+y=w841:u32)
            n349 = Build Array(u8 85, w847, w846) -> (w842:u8[])
            n350 = Bundle By Name(cluster=T6 {"ID"=0, "TimeStamp"=0, "TimeFlag"=0, "SendType"=0, "RemoteFlag"=0, "ExternFlag"=0, "DataLen"=0, "Data"=[], "Reserved"=[]} ("Send"), "ID"=w841, "RemoteFlag"=w853, "ExternFlag"=w852, "DataLen"=u8 3, "Data"=w842) -> (w854:T6)
            n351 = Build Array(w854) -> (w855:T6[])
            n352 = Unbundle By Name(w845) -> ("DevType"=w858:T5, "DevIndex"=w857:u32, "CanIndex"=w856:T4)
            n353 = call "VCI_Transmit.vi"("Buffer"=w855, "CANIndex"=w856, "DevIndex"=w857, "DevType"=w858) -> ()  [unwired: 1 in, 7 out]
          }
          event "减速度_W": Value Change {
            w883 = u8 0 items=["数据帧", "遥控帧"]
            w884 = u8 0 items=["标准帧", "扩展帧"]
            # "索引地址"
            n354 = event-data() -> ()  [unwired: 2 out]
            n355 = property on="电机ID" class="CmbBox"() -> ("Value"=w875:string)  [unwired: 2 in, 2 out]
            n356 = Multiply ("乘")(x="减速度", y=u16 8) -> (x*y=w888:u16)
            n357 = Scan From String(format string="%x" ("格式字符串"), input string=w875, default 1=u8 0) -> (output 1=w872:u8)  [unwired: 2 in, 3 out]
            n358 = Split Number(x=w888) -> (hi(x)=w889:u8, lo(x)=w890:u8)
            n359 = Add(x=u32 16, y=w872) -> (x+y=w868:u32)
            n360 = Build Array(u8 86, w889, w890) -> (w869:u8[])
            n361 = Bundle By Name(cluster=T6 {"ID"=0, "TimeStamp"=0, "TimeFlag"=0, "SendType"=0, "RemoteFlag"=0, "ExternFlag"=0, "DataLen"=0, "Data"=[], "Reserved"=[]} ("Send"), "ID"=w868, "RemoteFlag"=w883, "ExternFlag"=w884, "DataLen"=u8 3, "Data"=w869) -> (w882:T6)
            n362 = Build Array(w882) -> (w881:T6[])
            n363 = Unbundle By Name(w871) -> ("DevType"=w878:T5, "DevIndex"=w879:u32, "CanIndex"=w880:T4)
            n364 = call "VCI_Transmit.vi"("Buffer"=w881, "CANIndex"=w880, "DevIndex"=w879, "DevType"=w878) -> ()  [unwired: 1 in, 7 out]
          }
          event "AI_K0_W": Value Change {
            w903 = u8 0 items=["数据帧", "遥控帧"]
            w902 = u8 0 items=["标准帧", "扩展帧"]
            # "索引地址"
            n365 = event-data() -> ()  [unwired: 2 out]
            n366 = property on="电机ID" class="CmbBox"() -> ("Value"=w911:string)  [unwired: 2 in, 2 out]
            n367 = Scan From String(format string="%x" ("格式字符串"), input string=w911, default 1=u8 0) -> (output 1=w914:u8)  [unwired: 2 in, 3 out]
            n368 = Split Number(x="A电流零偏") -> (hi(x)=w899:u8, lo(x)=w898:u8)
            n369 = Add(x=u32 16, y=w914) -> (x+y=w893:u32)
            n370 = Build Array(u8 90, w899, w898) -> (w894:u8[])
            n371 = Bundle By Name(cluster=T6 {"ID"=0, "TimeStamp"=0, "TimeFlag"=0, "SendType"=0, "RemoteFlag"=0, "ExternFlag"=0, "DataLen"=0, "Data"=[], "Reserved"=[]} ("Send"), "ID"=w893, "RemoteFlag"=w903, "ExternFlag"=w902, "DataLen"=u8 3, "Data"=w894) -> (w904:T6)
            n372 = Build Array(w904) -> (w905:T6[])
            n373 = Unbundle By Name(w897) -> ("DevType"=w908:T5, "DevIndex"=w907:u32, "CanIndex"=w906:T4)
            n374 = call "VCI_Transmit.vi"("Buffer"=w905, "CANIndex"=w906, "DevIndex"=w907, "DevType"=w908) -> ()  [unwired: 1 in, 7 out]
          }
          event "BI_K0_W": Value Change {
            w927 = u8 0 items=["数据帧", "遥控帧"]
            w926 = u8 0 items=["标准帧", "扩展帧"]
            # "索引地址"
            n375 = event-data() -> ()  [unwired: 2 out]
            n376 = property on="电机ID" class="CmbBox"() -> ("Value"=w935:string)  [unwired: 2 in, 2 out]
            n377 = Scan From String(format string="%x" ("格式字符串"), input string=w935, default 1=u8 0) -> (output 1=w938:u8)  [unwired: 2 in, 3 out]
            n378 = Split Number(x="B电流零偏") -> (hi(x)=w923:u8, lo(x)=w922:u8)
            n379 = Add(x=u32 16, y=w938) -> (x+y=w917:u32)
            n380 = Build Array(u8 91, w923, w922) -> (w918:u8[])
            n381 = Bundle By Name(cluster=T6 {"ID"=0, "TimeStamp"=0, "TimeFlag"=0, "SendType"=0, "RemoteFlag"=0, "ExternFlag"=0, "DataLen"=0, "Data"=[], "Reserved"=[]} ("Send"), "ID"=w917, "RemoteFlag"=w927, "ExternFlag"=w926, "DataLen"=u8 3, "Data"=w918) -> (w928:T6)
            n382 = Build Array(w928) -> (w929:T6[])
            n383 = Unbundle By Name(w921) -> ("DevType"=w932:T5, "DevIndex"=w931:u32, "CanIndex"=w930:T4)
            n384 = call "VCI_Transmit.vi"("Buffer"=w929, "CANIndex"=w930, "DevIndex"=w931, "DevType"=w932) -> ()  [unwired: 1 in, 7 out]
          }
          event "CI_K0_W": Value Change {
            w951 = u8 0 items=["数据帧", "遥控帧"]
            w950 = u8 0 items=["标准帧", "扩展帧"]
            # "索引地址"
            n385 = event-data() -> ()  [unwired: 2 out]
            n386 = property on="电机ID" class="CmbBox"() -> ("Value"=w959:string)  [unwired: 2 in, 2 out]
            n387 = Scan From String(format string="%x" ("格式字符串"), input string=w959, default 1=u8 0) -> (output 1=w962:u8)  [unwired: 2 in, 3 out]
            n388 = Split Number(x="C电流零偏") -> (hi(x)=w947:u8, lo(x)=w946:u8)
            n389 = Add(x=u32 16, y=w962) -> (x+y=w941:u32)
            n390 = Build Array(u8 92, w947, w946) -> (w942:u8[])
            n391 = Bundle By Name(cluster=T6 {"ID"=0, "TimeStamp"=0, "TimeFlag"=0, "SendType"=0, "RemoteFlag"=0, "ExternFlag"=0, "DataLen"=0, "Data"=[], "Reserved"=[]} ("Send"), "ID"=w941, "RemoteFlag"=w951, "ExternFlag"=w950, "DataLen"=u8 3, "Data"=w942) -> (w952:T6)
            n392 = Build Array(w952) -> (w953:T6[])
            n393 = Unbundle By Name(w945) -> ("DevType"=w956:T5, "DevIndex"=w955:u32, "CanIndex"=w954:T4)
            n394 = call "VCI_Transmit.vi"("Buffer"=w953, "CANIndex"=w954, "DevIndex"=w955, "DevType"=w956) -> ()  [unwired: 1 in, 7 out]
          }
          event "对准角_W": Value Change {
            w984 = u8 0 items=["数据帧", "遥控帧"]
            w985 = u8 0 items=["标准帧", "扩展帧"]
            # "索引地址"
            n395 = event-data() -> ()  [unwired: 2 out]
            n396 = property on="电机ID" class="CmbBox"() -> ("Value"=w976:string)  [unwired: 2 in, 2 out]
            n397 = Multiply(x="对准角", y=u16 8) -> (x*y=w967:dbl)
            n398 = Scan From String(format string="%x" ("格式字符串"), input string=w976, default 1=u8 0) -> (output 1=w973:u8)  [unwired: 2 in, 3 out]
            n399 = To Unsigned Word Integer(number=w967) -> (unsigned 16bit integer=w966:u16)
            n400 = Add(x=u32 16, y=w973) -> (x+y=w971:u32)
            n401 = Split Number(x=w966) -> (hi(x)=w988:u8, lo(x)=w989:u8)
            n402 = Build Array(u8 93, w988, w989) -> (w970:u8[])
            n403 = Bundle By Name(cluster=T6 {"ID"=0, "TimeStamp"=0, "TimeFlag"=0, "SendType"=0, "RemoteFlag"=0, "ExternFlag"=0, "DataLen"=0, "Data"=[], "Reserved"=[]} ("Send"), "ID"=w971, "RemoteFlag"=w984, "ExternFlag"=w985, "DataLen"=u8 3, "Data"=w970) -> (w983:T6)
            n404 = Build Array(w983) -> (w982:T6[])
            n405 = Unbundle By Name(w972) -> ("DevType"=w979:T5, "DevIndex"=w980:u32, "CanIndex"=w981:T4)
            n406 = call "VCI_Transmit.vi"("Buffer"=w982, "CANIndex"=w981, "DevIndex"=w980, "DevType"=w979) -> ()  [unwired: 1 in, 7 out]
          }
          event "DATA_SAVE_W": Value Change {
            w1008 = u8 0 items=["数据帧", "遥控帧"]
            w1009 = u8 0 items=["标准帧", "扩展帧"]
            # "地址"
            n407 = event-data() -> ()  [unwired: 2 out]
            n408 = property on="电机ID" class="CmbBox"() -> ("Value"=w999:string)  [unwired: 2 in, 2 out]
            n409 = Scan From String(format string="%x" ("格式字符串"), input string=w999, default 1=u8 0) -> (output 1=w996:u8)  [unwired: 2 in, 3 out]
            n410 = call "Demo_MakeData.vi"("DataString"="50") -> ("Data"=w993:u8[], "DataLen"=w1004:u8)  [unwired: 9 out]
            n411 = Add(x=u32 16, y=w996) -> (x+y=w992:u32)
            n412 = Bundle By Name(cluster=T6 {"ID"=0, "TimeStamp"=0, "TimeFlag"=0, "SendType"=0, "RemoteFlag"=0, "ExternFlag"=0, "DataLen"=0, "Data"=[], "Reserved"=[]} ("Send"), "ID"=w992, "RemoteFlag"=w1008, "ExternFlag"=w1009, "DataLen"=w1004, "Data"=w993) -> (w1007:T6)
            n413 = Build Array(w1007) -> (w1006:T6[])
            n414 = Unbundle By Name(w995) -> ("DevType"=w1002:T5, "DevIndex"=w1003:u32, "CanIndex"=w1005:T4)
            n415 = call "VCI_Transmit.vi"("Buffer"=w1006, "CANIndex"=w1005, "DevIndex"=w1003, "DevType"=w1002) -> ()  [unwired: 1 in, 7 out]
          }
          event "Zero_SAVE_W": Value Change {
            w1024 = u8 0 items=["数据帧", "遥控帧"]
            w1023 = u8 0 items=["标准帧", "扩展帧"]
            # "地址"
            n416 = event-data() -> ()  [unwired: 2 out]
            n417 = property on="电机ID" class="CmbBox"() -> ("Value"=w1016:string)  [unwired: 2 in, 2 out]
            n418 = Scan From String(format string="%x" ("格式字符串"), input string=w1016, default 1=u8 0) -> (output 1=w1019:u8)  [unwired: 2 in, 3 out]
            n419 = Add(x=u32 16, y=w1019) -> (x+y=w1014:u32)
            n420 = call "Demo_MakeData.vi"("DataString"="75") -> ("Data"=w1020:u8[], "DataLen"=w1028:u8)  [unwired: 9 out]
            n421 = Bundle By Name(cluster=T6 {"ID"=0, "TimeStamp"=0, "TimeFlag"=0, "SendType"=0, "RemoteFlag"=0, "ExternFlag"=0, "DataLen"=0, "Data"=[], "Reserved"=[]} ("Send"), "ID"=w1014, "RemoteFlag"=w1024, "ExternFlag"=w1023, "DataLen"=w1028, "Data"=w1020) -> (w1025:T6)
            n422 = Build Array(w1025) -> (w1026:T6[])
            n423 = Unbundle By Name(w1021) -> ("DevType"=w1030:T5, "DevIndex"=w1029:u32, "CanIndex"=w1027:T4)
            n424 = call "VCI_Transmit.vi"("Buffer"=w1026, "CANIndex"=w1027, "DevIndex"=w1029, "DevType"=w1030) -> ()  [unwired: 1 in, 7 out]
          }
          event "设定位置_R": Value Change {
            w1040 = u8 0 items=["数据帧", "遥控帧"]
            w1039 = u8 0 items=["标准帧", "扩展帧"]
            # "地址"
            n425 = event-data() -> ()  [unwired: 2 out]
            n426 = property on="电机ID" class="CmbBox"() -> ("Value"=w1049:string)  [unwired: 2 in, 2 out]
            n427 = Scan From String(format string="%x" ("格式字符串"), input string=w1049, default 1=u8 0) -> (output 1=w1052:u8)  [unwired: 2 in, 3 out]
            n428 = call "Demo_MakeData.vi"("DataString"="40 ") -> ("Data"=w1035:u8[], "DataLen"=w1044:u8)  [unwired: 9 out]
            n429 = Add(x=u32 48, y=w1052) -> (x+y=w1034:u32)
            n430 = Bundle By Name(cluster=T6 {"ID"=0, "TimeStamp"=0, "TimeFlag"=0, "SendType"=0, "RemoteFlag"=0, "ExternFlag"=0, "DataLen"=0, "Data"=[], "Reserved"=[]} ("Send"), "ID"=w1034, "RemoteFlag"=w1040, "ExternFlag"=w1039, "DataLen"=w1044, "Data"=w1035) -> (w1041:T6)
            n431 = Build Array(w1041) -> (w1042:T6[])
            n432 = Unbundle By Name(w1037) -> ("DevType"=w1046:T5, "DevIndex"=w1045:u32, "CanIndex"=w1043:T4)
            n433 = call "VCI_Transmit.vi"("Buffer"=w1042, "CANIndex"=w1043, "DevIndex"=w1045, "DevType"=w1046) -> ()  [unwired: 1 in, 7 out]
          }
          event "设定速度_R": Value Change {
            w1071 = u8 0 items=["数据帧", "遥控帧"]
            w1072 = u8 0 items=["标准帧", "扩展帧"]
            # "地址"
            n434 = event-data() -> ()  [unwired: 2 out]
            n435 = property on="电机ID" class="CmbBox"() -> ("Value"=w1062:string)  [unwired: 2 in, 2 out]
            n436 = Scan From String(format string="%x" ("格式字符串"), input string=w1062, default 1=u8 0) -> (output 1=w1059:u8)  [unwired: 2 in, 3 out]
            n437 = call "Demo_MakeData.vi"("DataString"="41 ") -> ("Data"=w1056:u8[], "DataLen"=w1067:u8)  [unwired: 9 out]
            n438 = Add(x=u32 48, y=w1059) -> (x+y=w1055:u32)
            n439 = Bundle By Name(cluster=T6 {"ID"=0, "TimeStamp"=0, "TimeFlag"=0, "SendType"=0, "RemoteFlag"=0, "ExternFlag"=0, "DataLen"=0, "Data"=[], "Reserved"=[]} ("Send"), "ID"=w1055, "RemoteFlag"=w1071, "ExternFlag"=w1072, "DataLen"=w1067, "Data"=w1056) -> (w1070:T6)
            n440 = Build Array(w1070) -> (w1069:T6[])
            n441 = Unbundle By Name(w1058) -> ("DevType"=w1065:T5, "DevIndex"=w1066:u32, "CanIndex"=w1068:T4)
            n442 = call "VCI_Transmit.vi"("Buffer"=w1069, "CANIndex"=w1068, "DevIndex"=w1066, "DevType"=w1065) -> ()  [unwired: 1 in, 7 out]
          }
          event "设定电流_R": Value Change {
            w1092 = u8 0 items=["数据帧", "遥控帧"]
            w1093 = u8 0 items=["标准帧", "扩展帧"]
            # "地址"
            n443 = event-data() -> ()  [unwired: 2 out]
            n444 = property on="电机ID" class="CmbBox"() -> ("Value"=w1083:string)  [unwired: 2 in, 2 out]
            n445 = Scan From String(format string="%x" ("格式字符串"), input string=w1083, default 1=u8 0) -> (output 1=w1080:u8)  [unwired: 2 in, 3 out]
            n446 = call "Demo_MakeData.vi"("DataString"="42 ") -> ("Data"=w1077:u8[], "DataLen"=w1088:u8)  [unwired: 9 out]
            n447 = Add(x=u32 48, y=w1080) -> (x+y=w1076:u32)
            n448 = Bundle By Name(cluster=T6 {"ID"=0, "TimeStamp"=0, "TimeFlag"=0, "SendType"=0, "RemoteFlag"=0, "ExternFlag"=0, "DataLen"=0, "Data"=[], "Reserved"=[]} ("Send"), "ID"=w1076, "RemoteFlag"=w1092, "ExternFlag"=w1093, "DataLen"=w1088, "Data"=w1077) -> (w1091:T6)
            n449 = Build Array(w1091) -> (w1090:T6[])
            n450 = Unbundle By Name(w1079) -> ("DevType"=w1086:T5, "DevIndex"=w1087:u32, "CanIndex"=w1089:T4)
            n451 = call "VCI_Transmit.vi"("Buffer"=w1090, "CANIndex"=w1089, "DevIndex"=w1087, "DevType"=w1086) -> ()  [unwired: 1 in, 7 out]
          }
          event "电流环KP_R": Value Change {
            w1113 = u8 0 items=["数据帧", "遥控帧"]
            w1114 = u8 0 items=["标准帧", "扩展帧"]
            # "地址"
            n452 = event-data() -> ()  [unwired: 2 out]
            n453 = property on="电机ID" class="CmbBox"() -> ("Value"=w1104:string)  [unwired: 2 in, 2 out]
            n454 = Scan From String(format string="%x" ("格式字符串"), input string=w1104, default 1=u8 0) -> (output 1=w1101:u8)  [unwired: 2 in, 3 out]
            n455 = call "Demo_MakeData.vi"("DataString"="51 ") -> ("Data"=w1098:u8[], "DataLen"=w1109:u8)  [unwired: 9 out]
            n456 = Add(x=u32 48, y=w1101) -> (x+y=w1097:u32)
            n457 = Bundle By Name(cluster=T6 {"ID"=0, "TimeStamp"=0, "TimeFlag"=0, "SendType"=0, "RemoteFlag"=0, "ExternFlag"=0, "DataLen"=0, "Data"=[], "Reserved"=[]} ("Send"), "ID"=w1097, "RemoteFlag"=w1113, "ExternFlag"=w1114, "DataLen"=w1109, "Data"=w1098) -> (w1112:T6)
            n458 = Build Array(w1112) -> (w1111:T6[])
            n459 = Unbundle By Name(w1100) -> ("DevType"=w1107:T5, "DevIndex"=w1108:u32, "CanIndex"=w1110:T4)
            n460 = call "VCI_Transmit.vi"("Buffer"=w1111, "CANIndex"=w1110, "DevIndex"=w1108, "DevType"=w1107) -> ()  [unwired: 1 in, 7 out]
          }
          event "电流环KI_R": Value Change {
            w1134 = u8 0 items=["数据帧", "遥控帧"]
            w1135 = u8 0 items=["标准帧", "扩展帧"]
            # "地址"
            n461 = event-data() -> ()  [unwired: 2 out]
            n462 = property on="电机ID" class="CmbBox"() -> ("Value"=w1125:string)  [unwired: 2 in, 2 out]
            n463 = Scan From String(format string="%x" ("格式字符串"), input string=w1125, default 1=u8 0) -> (output 1=w1122:u8)  [unwired: 2 in, 3 out]
            n464 = call "Demo_MakeData.vi"("DataString"="52 ") -> ("Data"=w1119:u8[], "DataLen"=w1130:u8)  [unwired: 9 out]
            n465 = Add(x=u32 48, y=w1122) -> (x+y=w1118:u32)
            n466 = Bundle By Name(cluster=T6 {"ID"=0, "TimeStamp"=0, "TimeFlag"=0, "SendType"=0, "RemoteFlag"=0, "ExternFlag"=0, "DataLen"=0, "Data"=[], "Reserved"=[]} ("Send"), "ID"=w1118, "RemoteFlag"=w1134, "ExternFlag"=w1135, "DataLen"=w1130, "Data"=w1119) -> (w1133:T6)
            n467 = Build Array(w1133) -> (w1132:T6[])
            n468 = Unbundle By Name(w1121) -> ("DevType"=w1128:T5, "DevIndex"=w1129:u32, "CanIndex"=w1131:T4)
            n469 = call "VCI_Transmit.vi"("Buffer"=w1132, "CANIndex"=w1131, "DevIndex"=w1129, "DevType"=w1128) -> ()  [unwired: 1 in, 7 out]
          }
          event "速度环KP_R": Value Change {
            w1145 = u8 0 items=["数据帧", "遥控帧"]
            w1144 = u8 0 items=["标准帧", "扩展帧"]
            # "地址"
            n470 = event-data() -> ()  [unwired: 2 out]
            n471 = property on="电机ID" class="CmbBox"() -> ("Value"=w1154:string)  [unwired: 2 in, 2 out]
            n472 = Scan From String(format string="%x" ("格式字符串"), input string=w1154, default 1=u8 0) -> (output 1=w1157:u8)  [unwired: 2 in, 3 out]
            n473 = call "Demo_MakeData.vi"("DataString"="53 ") -> ("Data"=w1140:u8[], "DataLen"=w1149:u8)  [unwired: 9 out]
            n474 = Add(x=u32 48, y=w1157) -> (x+y=w1139:u32)
            n475 = Bundle By Name(cluster=T6 {"ID"=0, "TimeStamp"=0, "TimeFlag"=0, "SendType"=0, "RemoteFlag"=0, "ExternFlag"=0, "DataLen"=0, "Data"=[], "Reserved"=[]} ("Send"), "ID"=w1139, "RemoteFlag"=w1145, "ExternFlag"=w1144, "DataLen"=w1149, "Data"=w1140) -> (w1146:T6)
            n476 = Build Array(w1146) -> (w1147:T6[])
            n477 = Unbundle By Name(w1142) -> ("DevType"=w1151:T5, "DevIndex"=w1150:u32, "CanIndex"=w1148:T4)
            n478 = call "VCI_Transmit.vi"("Buffer"=w1147, "CANIndex"=w1148, "DevIndex"=w1150, "DevType"=w1151) -> ()  [unwired: 1 in, 7 out]
          }
          event "速度环KI_R": Value Change {
            w1166 = u8 0 items=["数据帧", "遥控帧"]
            w1165 = u8 0 items=["标准帧", "扩展帧"]
            # "地址"
            n479 = event-data() -> ()  [unwired: 2 out]
            n480 = property on="电机ID" class="CmbBox"() -> ("Value"=w1175:string)  [unwired: 2 in, 2 out]
            n481 = Scan From String(format string="%x" ("格式字符串"), input string=w1175, default 1=u8 0) -> (output 1=w1178:u8)  [unwired: 2 in, 3 out]
            n482 = call "Demo_MakeData.vi"("DataString"="54 ") -> ("Data"=w1161:u8[], "DataLen"=w1170:u8)  [unwired: 9 out]
            n483 = Add(x=u32 48, y=w1178) -> (x+y=w1160:u32)
            n484 = Bundle By Name(cluster=T6 {"ID"=0, "TimeStamp"=0, "TimeFlag"=0, "SendType"=0, "RemoteFlag"=0, "ExternFlag"=0, "DataLen"=0, "Data"=[], "Reserved"=[]} ("Send"), "ID"=w1160, "RemoteFlag"=w1166, "ExternFlag"=w1165, "DataLen"=w1170, "Data"=w1161) -> (w1167:T6)
            n485 = Build Array(w1167) -> (w1168:T6[])
            n486 = Unbundle By Name(w1163) -> ("DevType"=w1172:T5, "DevIndex"=w1171:u32, "CanIndex"=w1169:T4)
            n487 = call "VCI_Transmit.vi"("Buffer"=w1168, "CANIndex"=w1169, "DevIndex"=w1171, "DevType"=w1172) -> ()  [unwired: 1 in, 7 out]
          }
          event "加速度_R": Value Change {
            w1197 = u8 0 items=["数据帧", "遥控帧"]
            w1198 = u8 0 items=["标准帧", "扩展帧"]
            # "地址"
            n488 = event-data() -> ()  [unwired: 2 out]
            n489 = property on="电机ID" class="CmbBox"() -> ("Value"=w1188:string)  [unwired: 2 in, 2 out]
            n490 = Scan From String(format string="%x" ("格式字符串"), input string=w1188, default 1=u8 0) -> (output 1=w1185:u8)  [unwired: 2 in, 3 out]
            n491 = call "Demo_MakeData.vi"("DataString"="55") -> ("Data"=w1182:u8[], "DataLen"=w1193:u8)  [unwired: 9 out]
            n492 = Add(x=u32 48, y=w1185) -> (x+y=w1181:u32)
            n493 = Bundle By Name(cluster=T6 {"ID"=0, "TimeStamp"=0, "TimeFlag"=0, "SendType"=0, "RemoteFlag"=0, "ExternFlag"=0, "DataLen"=0, "Data"=[], "Reserved"=[]} ("Send"), "ID"=w1181, "RemoteFlag"=w1197, "ExternFlag"=w1198, "DataLen"=w1193, "Data"=w1182) -> (w1196:T6)
            n494 = Build Array(w1196) -> (w1195:T6[])
            n495 = Unbundle By Name(w1184) -> ("DevType"=w1191:T5, "DevIndex"=w1192:u32, "CanIndex"=w1194:T4)
            n496 = call "VCI_Transmit.vi"("Buffer"=w1195, "CANIndex"=w1194, "DevIndex"=w1192, "DevType"=w1191) -> ()  [unwired: 1 in, 7 out]
          }
          event "减速度_R": Value Change {
            w1208 = u8 0 items=["数据帧", "遥控帧"]
            w1207 = u8 0 items=["标准帧", "扩展帧"]
            # "地址"
            n497 = event-data() -> ()  [unwired: 2 out]
            n498 = property on="电机ID" class="CmbBox"() -> ("Value"=w1217:string)  [unwired: 2 in, 2 out]
            n499 = Scan From String(format string="%x" ("格式字符串"), input string=w1217, default 1=u8 0) -> (output 1=w1220:u8)  [unwired: 2 in, 3 out]
            n500 = call "Demo_MakeData.vi"("DataString"="56") -> ("Data"=w1203:u8[], "DataLen"=w1212:u8)  [unwired: 9 out]
            n501 = Add(x=u32 48, y=w1220) -> (x+y=w1204:u32)
            n502 = Bundle By Name(cluster=T6 {"ID"=0, "TimeStamp"=0, "TimeFlag"=0, "SendType"=0, "RemoteFlag"=0, "ExternFlag"=0, "DataLen"=0, "Data"=[], "Reserved"=[]} ("Send"), "ID"=w1204, "RemoteFlag"=w1208, "ExternFlag"=w1207, "DataLen"=w1212, "Data"=w1203) -> (w1209:T6)
            n503 = Build Array(w1209) -> (w1210:T6[])
            n504 = Unbundle By Name(w1205) -> ("DevType"=w1214:T5, "DevIndex"=w1213:u32, "CanIndex"=w1211:T4)
            n505 = call "VCI_Transmit.vi"("Buffer"=w1210, "CANIndex"=w1211, "DevIndex"=w1213, "DevType"=w1214) -> ()  [unwired: 1 in, 7 out]
          }
          event "AI_K0_R": Value Change {
            w1229 = u8 0 items=["数据帧", "遥控帧"]
            w1228 = u8 0 items=["标准帧", "扩展帧"]
            # "地址"
            n506 = event-data() -> ()  [unwired: 2 out]
            n507 = property on="电机ID" class="CmbBox"() -> ("Value"=w1238:string)  [unwired: 2 in, 2 out]
            n508 = Scan From String(format string="%x" ("格式字符串"), input string=w1238, default 1=u8 0) -> (output 1=w1241:u8)  [unwired: 2 in, 3 out]
            n509 = call "Demo_MakeData.vi"("DataString"="5A") -> ("Data"=w1224:u8[], "DataLen"=w1233:u8)  [unwired: 9 out]
            n510 = Add(x=u32 48, y=w1241) -> (x+y=w1223:u32)
            n511 = Bundle By Name(cluster=T6 {"ID"=0, "TimeStamp"=0, "TimeFlag"=0, "SendType"=0, "RemoteFlag"=0, "ExternFlag"=0, "DataLen"=0, "Data"=[], "Reserved"=[]} ("Send"), "ID"=w1223, "RemoteFlag"=w1229, "ExternFlag"=w1228, "DataLen"=w1233, "Data"=w1224) -> (w1230:T6)
            n512 = Build Array(w1230) -> (w1231:T6[])
            n513 = Unbundle By Name(w1226) -> ("DevType"=w1235:T5, "DevIndex"=w1234:u32, "CanIndex"=w1232:T4)
            n514 = call "VCI_Transmit.vi"("Buffer"=w1231, "CANIndex"=w1232, "DevIndex"=w1234, "DevType"=w1235) -> ()  [unwired: 1 in, 7 out]
          }
          event "BI_K0_R": Value Change {
            w1250 = u8 0 items=["数据帧", "遥控帧"]
            w1249 = u8 0 items=["标准帧", "扩展帧"]
            # "地址"
            n515 = event-data() -> ()  [unwired: 2 out]
            n516 = property on="电机ID" class="CmbBox"() -> ("Value"=w1259:string)  [unwired: 2 in, 2 out]
            n517 = Scan From String(format string="%x" ("格式字符串"), input string=w1259, default 1=u8 0) -> (output 1=w1262:u8)  [unwired: 2 in, 3 out]
            n518 = call "Demo_MakeData.vi"("DataString"="5B") -> ("Data"=w1245:u8[], "DataLen"=w1254:u8)  [unwired: 9 out]
            n519 = Add(x=u32 48, y=w1262) -> (x+y=w1244:u32)
            n520 = Bundle By Name(cluster=T6 {"ID"=0, "TimeStamp"=0, "TimeFlag"=0, "SendType"=0, "RemoteFlag"=0, "ExternFlag"=0, "DataLen"=0, "Data"=[], "Reserved"=[]} ("Send"), "ID"=w1244, "RemoteFlag"=w1250, "ExternFlag"=w1249, "DataLen"=w1254, "Data"=w1245) -> (w1251:T6)
            n521 = Build Array(w1251) -> (w1252:T6[])
            n522 = Unbundle By Name(w1247) -> ("DevType"=w1256:T5, "DevIndex"=w1255:u32, "CanIndex"=w1253:T4)
            n523 = call "VCI_Transmit.vi"("Buffer"=w1252, "CANIndex"=w1253, "DevIndex"=w1255, "DevType"=w1256) -> ()  [unwired: 1 in, 7 out]
          }
          event "CI_K0_R": Value Change {
            w1271 = u8 0 items=["数据帧", "遥控帧"]
            w1270 = u8 0 items=["标准帧", "扩展帧"]
            # "地址"
            n524 = event-data() -> ()  [unwired: 2 out]
            n525 = property on="电机ID" class="CmbBox"() -> ("Value"=w1280:string)  [unwired: 2 in, 2 out]
            n526 = Scan From String(format string="%x" ("格式字符串"), input string=w1280, default 1=u8 0) -> (output 1=w1283:u8)  [unwired: 2 in, 3 out]
            n527 = call "Demo_MakeData.vi"("DataString"="5C") -> ("Data"=w1266:u8[], "DataLen"=w1275:u8)  [unwired: 9 out]
            n528 = Add(x=u32 48, y=w1283) -> (x+y=w1265:u32)
            n529 = Bundle By Name(cluster=T6 {"ID"=0, "TimeStamp"=0, "TimeFlag"=0, "SendType"=0, "RemoteFlag"=0, "ExternFlag"=0, "DataLen"=0, "Data"=[], "Reserved"=[]} ("Send"), "ID"=w1265, "RemoteFlag"=w1271, "ExternFlag"=w1270, "DataLen"=w1275, "Data"=w1266) -> (w1272:T6)
            n530 = Build Array(w1272) -> (w1273:T6[])
            n531 = Unbundle By Name(w1268) -> ("DevType"=w1277:T5, "DevIndex"=w1276:u32, "CanIndex"=w1274:T4)
            n532 = call "VCI_Transmit.vi"("Buffer"=w1273, "CANIndex"=w1274, "DevIndex"=w1276, "DevType"=w1277) -> ()  [unwired: 1 in, 7 out]
          }
          event "对准角_R": Value Change {
            w1302 = u8 0 items=["数据帧", "遥控帧"]
            w1303 = u8 0 items=["标准帧", "扩展帧"]
            # "地址"
            n533 = event-data() -> ()  [unwired: 2 out]
            n534 = property on="电机ID" class="CmbBox"() -> ("Value"=w1293:string)  [unwired: 2 in, 2 out]
            n535 = Scan From String(format string="%x" ("格式字符串"), input string=w1293, default 1=u8 0) -> (output 1=w1290:u8)  [unwired: 2 in, 3 out]
            n536 = call "Demo_MakeData.vi"("DataString"="5D") -> ("Data"=w1287:u8[], "DataLen"=w1298:u8)  [unwired: 9 out]
            n537 = Add(x=u32 48, y=w1290) -> (x+y=w1288:u32)
            n538 = Bundle By Name(cluster=T6 {"ID"=0, "TimeStamp"=0, "TimeFlag"=0, "SendType"=0, "RemoteFlag"=0, "ExternFlag"=0, "DataLen"=0, "Data"=[], "Reserved"=[]} ("Send"), "ID"=w1288, "RemoteFlag"=w1302, "ExternFlag"=w1303, "DataLen"=w1298, "Data"=w1287) -> (w1301:T6)
            n539 = Build Array(w1301) -> (w1300:T6[])
            n540 = Unbundle By Name(w1289) -> ("DevType"=w1296:T5, "DevIndex"=w1297:u32, "CanIndex"=w1299:T4)
            n541 = call "VCI_Transmit.vi"("Buffer"=w1300, "CANIndex"=w1299, "DevIndex"=w1297, "DevType"=w1296) -> ()  [unwired: 1 in, 7 out]
          }
          event "保存": Value Change {
            w1330 = "-"
            n542 = event-data() -> ()  [unwired: 2 out]
            n543 = Get Date/Time String(want seconds? (F)=TRUE) -> (date string=w1310:string, time string=w1331:string)  [unwired: 2 in]
            n544 = Search and Replace String(input string=w1310, search string="/", replace string="-") -> (result string=w1316:string)  [unwired: 5 in, 3 out]
            n545 = Search and Replace String(input string=w1331, search string=":", replace string="-") -> (result string=w1328:string)  [unwired: 5 in, 3 out]
            n546 = property on="保存_S" class="Bool (严格)"() -> ("Value"=w1322:bool)  [unwired: 2 in, 2 out]
            n547 = Search and Replace String(input string=w1316, search string="/", replace string="-") -> (result string=w1311:string)  [unwired: 5 in, 3 out]
            n548 = Search and Replace String(input string=w1328, search string=":", replace string="-") -> (result string=w1329:string)  [unwired: 5 in, 3 out]
            n549 = Not(x=w1322) -> (.not. x?=w1318:bool)
            n550 = property on="保存_S" class="Bool (严格)"("Value"=w1318) -> ()  [unwired: 2 in, 2 out]
            n551 = Concatenate Strings("D:\\PMSM\\", w1311, w1330, w1329, w1330, "电机数据存储", ".txt") -> (w1308:string)
            n552 = Select(t=w1308, s=w1318, f="") -> (s? t:f=w1323:string)
            n553 = String To Path(string=w1323) -> (path=w1309:path)
            n554 = local write "存储路径"(w1309) -> ()
          }
          event "Close": Value Change {
            w1343 = T10 1 items=["OK"=1, "ERROR1"=0, "ERROR2"=-1] ("y")
            n555 = event-data() -> ()  [unwired: 2 out]
            n556 = Unbundle By Name(w1347) -> ("DevType"=w1346:T5, "DevIndex"=w1345:u32)
            n557 = call "VCI_CloseDevice.vi"("DevIndex"=w1345, "DevType"=w1346) -> ("Return Val"=w1344:T10)  [unwired: 1 in, 8 out]
            n558 = Equal?(x=w1344, y=w1343) -> (x = y?=w1341:bool)
            n559 = Not(x=w1341) -> (.not. x?=w1337:bool)
            n560 = Bundle By Name(cluster=cluster{"CANOpen":bool} {"CANOpen"=FALSE} ("事件数据"), "CANOpen"=w1337) -> (w1336:cluster{"CANOpen":bool})
            n561 = Bundle By Name(cluster=w1342, "Open"=w1337) -> (w1340:cluster{"Open":bool, "SendCnt":u32})
            n562 = local write "Open"(w1337) -> ()
            n563 = Generate User Event(user event=w1339, event data cluster=w1336) -> ()  [unwired: 1 in, 2 out]
          }
          event User Event {
            w1358 = u8 0
            w1357 = u8 2
            n564 = event-data() -> ("CANOpen"=w1351:bool)  [unwired: 1 out]
            "Open" <- w1351
            n565 = Not(x=w1351) -> (.not. x?=w1352:bool)
            n566 = Select(t=w1357, s=w1351, f=w1358) -> (s? t:f=w1350:u8)
            n567 = Select(t=w1358, s=w1351, f=w1357) -> (s? t:f=w1349:u8)
            n568 = property class="VI"("Front Panel.Closeable"=w1352) -> ()  [unwired: 2 in, 2 out]
            n569 = property on="Close" class="Bool"("DisabledEnum"=w1349) -> ()  [unwired: 2 in, 2 out]
            n570 = property on="ID" class="DigNum (严格)"("DisabledEnum"=w1349) -> ()  [unwired: 2 in, 2 out]
            n571 = property on="Data" class="Str"("DisabledEnum"=w1349) -> ()  [unwired: 2 in, 2 out]
            n572 = property on="Format" class="Ring (严格)"("DisabledEnum"=w1349) -> ()  [unwired: 2 in, 2 out]
            n573 = property on="Type" class="Ring (严格)"("DisabledEnum"=w1349) -> ()  [unwired: 2 in, 2 out]
            n574 = property on="Send" class="Bool"("DisabledEnum"=w1349) -> ()  [unwired: 2 in, 2 out]
            n575 = Select(t=enum16{"Init", "Wait", "Run", "Exit"}."Run", s=w1351, f=enum16{"Init", "Wait", "Run", "Exit"}."Wait") -> (s? t:f=w1354:enum16{"Init", "Wait", "Run", "Exit"})
            n576 = property on="Fliter" class="Ring (严格)"("DisabledEnum"=w1350) -> ()  [unwired: 2 in, 2 out]
            n577 = property on="DevType" class="Ring (严格)"("DisabledEnum"=w1350) -> ()  [unwired: 2 in, 2 out]
            n578 = property on="Channel" class="Ring (严格)"("DisabledEnum"=w1350) -> ()  [unwired: 2 in, 2 out]
            n579 = property on="AccCode" class="DigNum (严格)"("DisabledEnum"=w1350) -> ()  [unwired: 2 in, 2 out]
            n580 = property on="AccMask" class="DigNum (严格)"("DisabledEnum"=w1350) -> ()  [unwired: 2 in, 2 out]
            n581 = property on="InitFlag" class="Ring (严格)"("DisabledEnum"=w1350) -> ()  [unwired: 2 in, 2 out]
            n582 = property on="Mode" class="Ring (严格)"("DisabledEnum"=w1350) -> ()  [unwired: 2 in, 2 out]
            n583 = property on="kBaudRate" class="Ring (严格)"("DisabledEnum"=w1350) -> ()  [unwired: 2 in, 2 out]
            n584 = property on="电机ID_W" class="Bool"("DisabledEnum"=w1349) -> ()  [unwired: 2 in, 2 out]
            n585 = property on="监测_W" class="Bool"("DisabledEnum"=w1349) -> ()  [unwired: 2 in, 2 out]
            n586 = property on="模式_W" class="Bool"("DisabledEnum"=w1349) -> ()  [unwired: 2 in, 2 out]
            n587 = property on="模式_R" class="Bool"("DisabledEnum"=w1349) -> ()  [unwired: 2 in, 2 out]
            n588 = property on="设定位置_W" class="Bool"("DisabledEnum"=w1349) -> ()  [unwired: 2 in, 2 out]
            n589 = property on="设定位置_R" class="Bool"("DisabledEnum"=w1349) -> ()  [unwired: 2 in, 2 out]
            n590 = property on="设定速度_W" class="Bool"("DisabledEnum"=w1349) -> ()  [unwired: 2 in, 2 out]
            n591 = property on="设定速度_R" class="Bool"("DisabledEnum"=w1349) -> ()  [unwired: 2 in, 2 out]
            n592 = property on="设定电流_W" class="Bool"("DisabledEnum"=w1349) -> ()  [unwired: 2 in, 2 out]
            n593 = property on="设定电流_R" class="Bool"("DisabledEnum"=w1349) -> ()  [unwired: 2 in, 2 out]
            n594 = property on="保存" class="Bool"("DisabledEnum"=w1349) -> ()  [unwired: 2 in, 2 out]
            n595 = property on="电流环KP_W" class="Bool"("DisabledEnum"=w1349) -> ()  [unwired: 2 in, 2 out]
            n596 = property on="电流环KI_W" class="Bool"("DisabledEnum"=w1349) -> ()  [unwired: 2 in, 2 out]
            n597 = property on="速度环KP_W" class="Bool"("DisabledEnum"=w1349) -> ()  [unwired: 2 in, 2 out]
            n598 = property on="速度环KI_W" class="Bool"("DisabledEnum"=w1349) -> ()  [unwired: 2 in, 2 out]
            n599 = property on="加速度_W" class="Bool"("DisabledEnum"=w1349) -> ()  [unwired: 2 in, 2 out]
            n600 = property on="AI_K0_W" class="Bool"("DisabledEnum"=w1349) -> ()  [unwired: 2 in, 2 out]
            n601 = property on="BI_K0_W" class="Bool"("DisabledEnum"=w1349) -> ()  [unwired: 2 in, 2 out]
            n602 = property on="CI_K0_W" class="Bool"("DisabledEnum"=w1349) -> ()  [unwired: 2 in, 2 out]
            n603 = property on="DATA_SAVE_W" class="Bool"("DisabledEnum"=w1349) -> ()  [unwired: 2 in, 2 out]
            n604 = property on="监测周期_W" class="Bool"("DisabledEnum"=w1349) -> ()  [unwired: 2 in, 2 out]
            n605 = property on="看门狗_W" class="Bool"("DisabledEnum"=w1349) -> ()  [unwired: 2 in, 2 out]
            n606 = property on="电流环KP_R" class="Bool"("DisabledEnum"=w1349) -> ()  [unwired: 2 in, 2 out]
            n607 = property on="电流环KI_R" class="Bool"("DisabledEnum"=w1349) -> ()  [unwired: 2 in, 2 out]
            n608 = property on="速度环KP_R" class="Bool"("DisabledEnum"=w1349) -> ()  [unwired: 2 in, 2 out]
            n609 = property on="速度环KI_R" class="Bool"("DisabledEnum"=w1349) -> ()  [unwired: 2 in, 2 out]
            n610 = property on="加速度_R" class="Bool"("DisabledEnum"=w1349) -> ()  [unwired: 2 in, 2 out]
            n611 = property on="AI_K0_R" class="Bool"("DisabledEnum"=w1349) -> ()  [unwired: 2 in, 2 out]
            n612 = property on="BI_K0_R" class="Bool"("DisabledEnum"=w1349) -> ()  [unwired: 2 in, 2 out]
            n613 = property on="CI_K0_R" class="Bool"("DisabledEnum"=w1349) -> ()  [unwired: 2 in, 2 out]
            n614 = property on="监测周期_R" class="Bool"("DisabledEnum"=w1349) -> ()  [unwired: 2 in, 2 out]
            n615 = property on="看门狗周期_W" class="Bool"("DisabledEnum"=w1349) -> ()  [unwired: 2 in, 2 out]
            n616 = property on="看门狗周期_R" class="Bool"("DisabledEnum"=w1349) -> ()  [unwired: 2 in, 2 out]
            n617 = property on="减速度_R" class="Bool"("DisabledEnum"=w1349) -> ()  [unwired: 2 in, 2 out]
            n618 = property on="减速度_W" class="Bool"("DisabledEnum"=w1349) -> ()  [unwired: 2 in, 2 out]
            n619 = property on="对准角_W" class="Bool"("DisabledEnum"=w1349) -> ()  [unwired: 2 in, 2 out]
            n620 = property on="对准角_R" class="Bool"("DisabledEnum"=w1349) -> ()  [unwired: 2 in, 2 out]
            n621 = property on="电机校准_W" class="Bool"("DisabledEnum"=w1349) -> ()  [unwired: 2 in, 2 out]
            n622 = property on="极对数_W" class="Bool"("DisabledEnum"=w1349) -> ()  [unwired: 2 in, 2 out]
            n623 = property on="极对数_R" class="Bool"("DisabledEnum"=w1349) -> ()  [unwired: 2 in, 2 out]
            n624 = property on="编码器线数_W" class="Bool"("DisabledEnum"=w1349) -> ()  [unwired: 2 in, 2 out]
            n625 = property on="编码器线数_R" class="Bool"("DisabledEnum"=w1349) -> ()  [unwired: 2 in, 2 out]
            n626 = property on="速度限制_W" class="Bool"("DisabledEnum"=w1349) -> ()  [unwired: 2 in, 2 out]
            n627 = property on="速度限制_R" class="Bool"("DisabledEnum"=w1349) -> ()  [unwired: 2 in, 2 out]
            n628 = property on="电流限制_W" class="Bool"("DisabledEnum"=w1349) -> ()  [unwired: 2 in, 2 out]
            n629 = property on="电流限制_R" class="Bool"("DisabledEnum"=w1349) -> ()  [unwired: 2 in, 2 out]
            n630 = property on="W1_W" class="Bool"("DisabledEnum"=w1349) -> ()  [unwired: 2 in, 2 out]
            n631 = property on="W1_R" class="Bool"("DisabledEnum"=w1349) -> ()  [unwired: 2 in, 2 out]
            n632 = property on="W2_W" class="Bool"("DisabledEnum"=w1349) -> ()  [unwired: 2 in, 2 out]
            n633 = property on="W2_R" class="Bool"("DisabledEnum"=w1349) -> ()  [unwired: 2 in, 2 out]
            n634 = property on="W3_W" class="Bool"("DisabledEnum"=w1349) -> ()  [unwired: 2 in, 2 out]
            n635 = property on="W3_R" class="Bool"("DisabledEnum"=w1349) -> ()  [unwired: 2 in, 2 out]
            n636 = property on="T3_R" class="Bool"("DisabledEnum"=w1349) -> ()  [unwired: 2 in, 2 out]
            n637 = property on="T4_W" class="Bool"("DisabledEnum"=w1349) -> ()  [unwired: 2 in, 2 out]
            n638 = property on="T1_W" class="Bool"("DisabledEnum"=w1349) -> ()  [unwired: 2 in, 2 out]
            n639 = property on="T2_R" class="Bool"("DisabledEnum"=w1349) -> ()  [unwired: 2 in, 2 out]
            n640 = property on="T1_R" class="Bool"("DisabledEnum"=w1349) -> ()  [unwired: 2 in, 2 out]
            n641 = property on="T2_W" class="Bool"("DisabledEnum"=w1349) -> ()  [unwired: 2 in, 2 out]
            n642 = property on="W4_W" class="Bool"("DisabledEnum"=w1349) -> ()  [unwired: 2 in, 2 out]
            n643 = property on="W4_R" class="Bool"("DisabledEnum"=w1349) -> ()  [unwired: 2 in, 2 out]
            n644 = property on="T3_W" class="Bool"("DisabledEnum"=w1349) -> ()  [unwired: 2 in, 2 out]
            n645 = property on="W_EN_R" class="Bool"("DisabledEnum"=w1349) -> ()  [unwired: 2 in, 2 out]
            n646 = property on="I_EN_W" class="Bool"("DisabledEnum"=w1349) -> ()  [unwired: 2 in, 2 out]
            n647 = property on="W_EN_W" class="Bool"("DisabledEnum"=w1349) -> ()  [unwired: 2 in, 2 out]
            n648 = property on="I_EN_R" class="Bool"("DisabledEnum"=w1349) -> ()  [unwired: 2 in, 2 out]
            n649 = property on="T4_R" class="Bool"("DisabledEnum"=w1349) -> ()  [unwired: 2 in, 2 out]
            n650 = property on="Direction_W" class="Bool"("DisabledEnum"=w1349) -> ()  [unwired: 2 in, 2 out]
            n651 = property on="Servo_EN_W" class="Bool"("DisabledEnum"=w1349) -> ()  [unwired: 2 in, 2 out]
            n652 = property on="Servo_EN_R" class="Bool"("DisabledEnum"=w1349) -> ()  [unwired: 2 in, 2 out]
            n653 = property on="Direction_R" class="Bool"("DisabledEnum"=w1349) -> ()  [unwired: 2 in, 2 out]
            n654 = property on="Servo_Count_W" class="Bool"("DisabledEnum"=w1349) -> ()  [unwired: 2 in, 2 out]
            n655 = property on="Kt_W" class="Bool"("DisabledEnum"=w1349) -> ()  [unwired: 2 in, 2 out]
            n656 = property on="Kt_R" class="Bool"("DisabledEnum"=w1349) -> ()  [unwired: 2 in, 2 out]
            n657 = property on="PosLimitEn_W" class="Bool"("DisabledEnum"=w1349) -> ()  [unwired: 2 in, 2 out]
            n658 = property on="PosLimitEn_R" class="Bool"("DisabledEnum"=w1349) -> ()  [unwired: 2 in, 2 out]
            n659 = property on="Gear_W" class="Bool"("DisabledEnum"=w1349) -> ()  [unwired: 2 in, 2 out]
            n660 = property on="Gear_R" class="Bool"("DisabledEnum"=w1349) -> ()  [unwired: 2 in, 2 out]
            n661 = property on="Servo_Count_R" class="Bool"("DisabledEnum"=w1349) -> ()  [unwired: 2 in, 2 out]
            n662 = property on="位置环KI_W" class="Bool"("DisabledEnum"=w1349) -> ()  [unwired: 2 in, 2 out]
            n663 = property on="上限位W" class="Bool"("DisabledEnum"=w1349) -> ()  [unwired: 2 in, 2 out]
            n664 = property on="上限位_R" class="Bool"("DisabledEnum"=w1349) -> ()  [unwired: 2 in, 2 out]
            n665 = property on="电压限制_W" class="Bool"("DisabledEnum"=w1349) -> ()  [unwired: 2 in, 2 out]
            n666 = property on="电压限制_R" class="Bool"("DisabledEnum"=w1349) -> ()  [unwired: 2 in, 2 out]
            n667 = property on="位置环KP_W" class="Bool"("DisabledEnum"=w1349) -> ()  [unwired: 2 in, 2 out]
            n668 = property on="位置环KP_R" class="Bool"("DisabledEnum"=w1349) -> ()  [unwired: 2 in, 2 out]
            n669 = property on="位置环KI_R" class="Bool"("DisabledEnum"=w1349) -> ()  [unwired: 2 in, 2 out]
            n670 = property on="ZeroEn_W" class="Bool"("DisabledEnum"=w1349) -> ()  [unwired: 2 in, 2 out]
            n671 = property on="Zero_SAVE_W" class="Bool"("DisabledEnum"=w1349) -> ()  [unwired: 2 in, 2 out]
            n672 = property on="设定力矩_W" class="Bool"("DisabledEnum"=w1349) -> ()  [unwired: 2 in, 2 out]
            n673 = property on="ZeroEn_R" class="Bool"("DisabledEnum"=w1349) -> ()  [unwired: 2 in, 2 out]
            n674 = property on="设定力矩_R" class="Bool"("DisabledEnum"=w1349) -> ()  [unwired: 2 in, 2 out]
            n675 = property on="Zero_R" class="Bool"("DisabledEnum"=w1349) -> ()  [unwired: 2 in, 2 out]
            n676 = property on="下限位_W" class="Bool"("DisabledEnum"=w1349) -> ()  [unwired: 2 in, 2 out]
            n677 = property on="下限位R" class="Bool"("DisabledEnum"=w1349) -> ()  [unwired: 2 in, 2 out]
          }
          event "T1_W": Value Change {
            w1376 = u8 0 items=["数据帧", "遥控帧"]
            w1377 = u8 0 items=["标准帧", "扩展帧"]
            # "索引地址"
            n678 = event-data() -> ()  [unwired: 2 out]
            n679 = property on="电机ID" class="CmbBox"() -> ("Value"=w1368:string)  [unwired: 2 in, 2 out]
            n680 = Scan From String(format string="%x" ("格式字符串"), input string=w1368, default 1=u8 0) -> (output 1=w1365:u8)  [unwired: 2 in, 3 out]
            n681 = Split Number(x="T1") -> (hi(x)=w1380:u8, lo(x)=w1381:u8)
            n682 = Add(x=u32 16, y=w1365) -> (x+y=w1364:u32)
            n683 = Build Array(u8 100, w1380, w1381) -> (w1363:u8[])
            n684 = Bundle By Name(cluster=T6 {"ID"=0, "TimeStamp"=0, "TimeFlag"=0, "SendType"=0, "RemoteFlag"=0, "ExternFlag"=0, "DataLen"=0, "Data"=[], "Reserved"=[]} ("Send"), "ID"=w1364, "RemoteFlag"=w1376, "ExternFlag"=w1377, "DataLen"=u8 3, "Data"=w1363) -> (w1375:T6)
            n685 = Build Array(w1375) -> (w1374:T6[])
            n686 = Unbundle By Name(w1360) -> ("DevType"=w1371:T5, "DevIndex"=w1372:u32, "CanIndex"=w1373:T4)
            n687 = call "VCI_Transmit.vi"("Buffer"=w1374, "CANIndex"=w1373, "DevIndex"=w1372, "DevType"=w1371) -> ()  [unwired: 1 in, 7 out]
          }
          event "W1_W": Value Change {
            w1400 = u8 0 items=["数据帧", "遥控帧"]
            w1401 = u8 0 items=["标准帧", "扩展帧"]
            # "索引地址"
            n688 = event-data() -> ()  [unwired: 2 out]
            n689 = property on="电机ID" class="CmbBox"() -> ("Value"=w1392:string)  [unwired: 2 in, 2 out]
            n690 = Scan From String(format string="%x" ("格式字符串"), input string=w1392, default 1=u8 0) -> (output 1=w1389:u8)  [unwired: 2 in, 3 out]
            n691 = Split Number(x="W1") -> (hi(x)=w1404:u8, lo(x)=w1405:u8)
            n692 = Add(x=u32 16, y=w1389) -> (x+y=w1386:u32)
            n693 = Build Array(u8 96, w1404, w1405) -> (w1387:u8[])
            n694 = Bundle By Name(cluster=T6 {"ID"=0, "TimeStamp"=0, "TimeFlag"=0, "SendType"=0, "RemoteFlag"=0, "ExternFlag"=0, "DataLen"=0, "Data"=[], "Reserved"=[]} ("Send"), "ID"=w1386, "RemoteFlag"=w1400, "ExternFlag"=w1401, "DataLen"=u8 3, "Data"=w1387) -> (w1399:T6)
            n695 = Build Array(w1399) -> (w1398:T6[])
            n696 = Unbundle By Name(w1388) -> ("DevType"=w1395:T5, "DevIndex"=w1396:u32, "CanIndex"=w1397:T4)
            n697 = call "VCI_Transmit.vi"("Buffer"=w1398, "CANIndex"=w1397, "DevIndex"=w1396, "DevType"=w1395) -> ()  [unwired: 1 in, 7 out]
          }
          event "W1_R": Value Change {
            w1414 = u8 0 items=["数据帧", "遥控帧"]
            w1413 = u8 0 items=["标准帧", "扩展帧"]
            # "地址"
            n698 = event-data() -> ()  [unwired: 2 out]
            n699 = property on="电机ID" class="CmbBox"() -> ("Value"=w1423:string)  [unwired: 2 in, 2 out]
            n700 = Scan From String(format string="%x" ("格式字符串"), input string=w1423, default 1=u8 0) -> (output 1=w1426:u8)  [unwired: 2 in, 3 out]
            n701 = call "Demo_MakeData.vi"("DataString"="60") -> ("Data"=w1409:u8[], "DataLen"=w1418:u8)  [unwired: 9 out]
            n702 = Add(x=u32 48, y=w1426) -> (x+y=w1410:u32)
            n703 = Bundle By Name(cluster=T6 {"ID"=0, "TimeStamp"=0, "TimeFlag"=0, "SendType"=0, "RemoteFlag"=0, "ExternFlag"=0, "DataLen"=0, "Data"=[], "Reserved"=[]} ("Send"), "ID"=w1410, "RemoteFlag"=w1414, "ExternFlag"=w1413, "DataLen"=w1418, "Data"=w1409) -> (w1415:T6)
            n704 = Build Array(w1415) -> (w1416:T6[])
            n705 = Unbundle By Name(w1411) -> ("DevType"=w1420:T5, "DevIndex"=w1419:u32, "CanIndex"=w1417:T4)
            n706 = call "VCI_Transmit.vi"("Buffer"=w1416, "CANIndex"=w1417, "DevIndex"=w1419, "DevType"=w1420) -> ()  [unwired: 1 in, 7 out]
          }
          event "W2_W": Value Change {
            w1438 = u8 0 items=["数据帧", "遥控帧"]
            w1437 = u8 0 items=["标准帧", "扩展帧"]
            # "索引地址"
            n707 = event-data() -> ()  [unwired: 2 out]
            n708 = property on="电机ID" class="CmbBox"() -> ("Value"=w1446:string)  [unwired: 2 in, 2 out]
            n709 = Scan From String(format string="%x" ("格式字符串"), input string=w1446, default 1=u8 0) -> (output 1=w1449:u8)  [unwired: 2 in, 3 out]
            n710 = Split Number(x="W2") -> (hi(x)=w1434:u8, lo(x)=w1433:u8)
            n711 = Add(x=u32 16, y=w1449) -> (x+y=w1431:u32)
            n712 = Build Array(u8 97, w1434, w1433) -> (w1430:u8[])
            n713 = Bundle By Name(cluster=T6 {"ID"=0, "TimeStamp"=0, "TimeFlag"=0, "SendType"=0, "RemoteFlag"=0, "ExternFlag"=0, "DataLen"=0, "Data"=[], "Reserved"=[]} ("Send"), "ID"=w1431, "RemoteFlag"=w1438, "ExternFlag"=w1437, "DataLen"=u8 3, "Data"=w1430) -> (w1439:T6)
            n714 = Build Array(w1439) -> (w1440:T6[])
            n715 = Unbundle By Name(w1432) -> ("DevType"=w1443:T5, "DevIndex"=w1442:u32, "CanIndex"=w1441:T4)
            n716 = call "VCI_Transmit.vi"("Buffer"=w1440, "CANIndex"=w1441, "DevIndex"=w1442, "DevType"=w1443) -> ()  [unwired: 1 in, 7 out]
          }
          event "W2_R": Value Change {
            w1469 = u8 0 items=["数据帧", "遥控帧"]
            w1470 = u8 0 items=["标准帧", "扩展帧"]
            # "地址"
            n717 = event-data() -> ()  [unwired: 2 out]
            n718 = property on="电机ID" class="CmbBox"() -> ("Value"=w1460:string)  [unwired: 2 in, 2 out]
            n719 = Scan From String(format string="%x" ("格式字符串"), input string=w1460, default 1=u8 0) -> (output 1=w1457:u8)  [unwired: 2 in, 3 out]
            n720 = call "Demo_MakeData.vi"("DataString"="61 ") -> ("Data"=w1454:u8[], "DataLen"=w1465:u8)  [unwired: 9 out]
            n721 = Add(x=u32 48, y=w1457) -> (x+y=w1455:u32)
            n722 = Bundle By Name(cluster=T6 {"ID"=0, "TimeStamp"=0, "TimeFlag"=0, "SendType"=0, "RemoteFlag"=0, "ExternFlag"=0, "DataLen"=0, "Data"=[], "Reserved"=[]} ("Send"), "ID"=w1455, "RemoteFlag"=w1469, "ExternFlag"=w1470, "DataLen"=w1465, "Data"=w1454) -> (w1468:T6)
            n723 = Build Array(w1468) -> (w1467:T6[])
            n724 = Unbundle By Name(w1453) -> ("DevType"=w1463:T5, "DevIndex"=w1464:u32, "CanIndex"=w1466:T4)
            n725 = call "VCI_Transmit.vi"("Buffer"=w1467, "CANIndex"=w1466, "DevIndex"=w1464, "DevType"=w1463) -> ()  [unwired: 1 in, 7 out]
          }
          event "W3_W": Value Change {
            w1484 = u8 0 items=["数据帧", "遥控帧"]
            w1483 = u8 0 items=["标准帧", "扩展帧"]
            # "索引地址"
            n726 = event-data() -> ()  [unwired: 2 out]
            n727 = property on="电机ID" class="CmbBox"() -> ("Value"=w1492:string)  [unwired: 2 in, 2 out]
            n728 = Scan From String(format string="%x" ("格式字符串"), input string=w1492, default 1=u8 0) -> (output 1=w1495:u8)  [unwired: 2 in, 3 out]
            n729 = Split Number(x="W3") -> (hi(x)=w1480:u8, lo(x)=w1481:u8)
            n730 = Add(x=u32 16, y=w1495) -> (x+y=w1477:u32)
            n731 = Build Array(u8 98, w1480, w1481) -> (w1476:u8[])
            n732 = Bundle By Name(cluster=T6 {"ID"=0, "TimeStamp"=0, "TimeFlag"=0, "SendType"=0, "RemoteFlag"=0, "ExternFlag"=0, "DataLen"=0, "Data"=[], "Reserved"=[]} ("Send"), "ID"=w1477, "RemoteFlag"=w1484, "ExternFlag"=w1483, "DataLen"=u8 3, "Data"=w1476) -> (w1485:T6)
            n733 = Build Array(w1485) -> (w1486:T6[])
            n734 = Unbundle By Name(w1478) -> ("DevType"=w1489:T5, "DevIndex"=w1488:u32, "CanIndex"=w1487:T4)
            n735 = call "VCI_Transmit.vi"("Buffer"=w1486, "CANIndex"=w1487, "DevIndex"=w1488, "DevType"=w1489) -> ()  [unwired: 1 in, 7 out]
          }
          event "W4_R": Value Change {
            w1514 = u8 0 items=["数据帧", "遥控帧"]
            w1515 = u8 0 items=["标准帧", "扩展帧"]
            # "地址"
            n736 = event-data() -> ()  [unwired: 2 out]
            n737 = property on="电机ID" class="CmbBox"() -> ("Value"=w1505:string)  [unwired: 2 in, 2 out]
            n738 = Scan From String(format string="%x" ("格式字符串"), input string=w1505, default 1=u8 0) -> (output 1=w1502:u8)  [unwired: 2 in, 3 out]
            n739 = call "Demo_MakeData.vi"("DataString"="63 ") -> ("Data"=w1499:u8[], "DataLen"=w1510:u8)  [unwired: 9 out]
            n740 = Add(x=u32 48, y=w1502) -> (x+y=w1500:u32)
            n741 = Bundle By Name(cluster=T6 {"ID"=0, "TimeStamp"=0, "TimeFlag"=0, "SendType"=0, "RemoteFlag"=0, "ExternFlag"=0, "DataLen"=0, "Data"=[], "Reserved"=[]} ("Send"), "ID"=w1500, "RemoteFlag"=w1514, "ExternFlag"=w1515, "DataLen"=w1510, "Data"=w1499) -> (w1513:T6)
            n742 = Build Array(w1513) -> (w1512:T6[])
            n743 = Unbundle By Name(w1501) -> ("DevType"=w1508:T5, "DevIndex"=w1509:u32, "CanIndex"=w1511:T4)
            n744 = call "VCI_Transmit.vi"("Buffer"=w1512, "CANIndex"=w1511, "DevIndex"=w1509, "DevType"=w1508) -> ()  [unwired: 1 in, 7 out]
          }
          event "T1_R": Value Change {
            w1535 = u8 0 items=["数据帧", "遥控帧"]
            w1536 = u8 0 items=["标准帧", "扩展帧"]
            # "地址"
            n745 = event-data() -> ()  [unwired: 2 out]
            n746 = property on="电机ID" class="CmbBox"() -> ("Value"=w1526:string)  [unwired: 2 in, 2 out]
            n747 = Scan From String(format string="%x" ("格式字符串"), input string=w1526, default 1=u8 0) -> (output 1=w1523:u8)  [unwired: 2 in, 3 out]
            n748 = call "Demo_MakeData.vi"("DataString"="64") -> ("Data"=w1521:u8[], "DataLen"=w1531:u8)  [unwired: 9 out]
            n749 = Add(x=u32 48, y=w1523) -> (x+y=w1522:u32)
            n750 = Bundle By Name(cluster=T6 {"ID"=0, "TimeStamp"=0, "TimeFlag"=0, "SendType"=0, "RemoteFlag"=0, "ExternFlag"=0, "DataLen"=0, "Data"=[], "Reserved"=[]} ("Send"), "ID"=w1522, "RemoteFlag"=w1535, "ExternFlag"=w1536, "DataLen"=w1531, "Data"=w1521) -> (w1534:T6)
            n751 = Build Array(w1534) -> (w1533:T6[])
            n752 = Unbundle By Name(w1519) -> ("DevType"=w1529:T5, "DevIndex"=w1530:u32, "CanIndex"=w1532:T4)
            n753 = call "VCI_Transmit.vi"("Buffer"=w1533, "CANIndex"=w1532, "DevIndex"=w1530, "DevType"=w1529) -> ()  [unwired: 1 in, 7 out]
          }
          event "W3_R": Value Change {
            w1556 = u8 0 items=["数据帧", "遥控帧"]
            w1557 = u8 0 items=["标准帧", "扩展帧"]
            # "地址"
            n754 = event-data() -> ()  [unwired: 2 out]
            n755 = property on="电机ID" class="CmbBox"() -> ("Value"=w1547:string)  [unwired: 2 in, 2 out]
            n756 = Scan From String(format string="%x" ("格式字符串"), input string=w1547, default 1=u8 0) -> (output 1=w1544:u8)  [unwired: 2 in, 3 out]
            n757 = call "Demo_MakeData.vi"("DataString"="62") -> ("Data"=w1541:u8[], "DataLen"=w1552:u8)  [unwired: 9 out]
            n758 = Add(x=u32 48, y=w1544) -> (x+y=w1542:u32)
            n759 = Bundle By Name(cluster=T6 {"ID"=0, "TimeStamp"=0, "TimeFlag"=0, "SendType"=0, "RemoteFlag"=0, "ExternFlag"=0, "DataLen"=0, "Data"=[], "Reserved"=[]} ("Send"), "ID"=w1542, "RemoteFlag"=w1556, "ExternFlag"=w1557, "DataLen"=w1552, "Data"=w1541) -> (w1555:T6)
            n760 = Build Array(w1555) -> (w1554:T6[])
            n761 = Unbundle By Name(w1540) -> ("DevType"=w1550:T5, "DevIndex"=w1551:u32, "CanIndex"=w1553:T4)
            n762 = call "VCI_Transmit.vi"("Buffer"=w1554, "CANIndex"=w1553, "DevIndex"=w1551, "DevType"=w1550) -> ()  [unwired: 1 in, 7 out]
          }
          event "W4_W": Value Change {
            w1569 = u8 0 items=["数据帧", "遥控帧"]
            w1568 = u8 0 items=["标准帧", "扩展帧"]
            (unwired) u8[] [] ("Reserved")
            # "索引地址"
            n763 = event-data() -> ()  [unwired: 2 out]
            n764 = property on="电机ID" class="CmbBox"() -> ("Value"=w1576:string)  [unwired: 2 in, 2 out]
            n765 = Scan From String(format string="%x" ("格式字符串"), input string=w1576, default 1=u8 0) -> (output 1=w1579:u8)  [unwired: 2 in, 3 out]
            n766 = Split Number(x="W4") -> (hi(x)=w1581:u8, lo(x)=w1580:u8)
            n767 = Add(x=u32 16, y=w1579) -> (x+y=w1565:u32)
            n768 = Build Array(u8 99, w1581, w1580) -> (w1564:u8[])
            n769 = Bundle By Name(cluster=T6 {"ID"=0, "TimeStamp"=0, "TimeFlag"=0, "SendType"=0, "RemoteFlag"=0, "ExternFlag"=0, "DataLen"=0, "Data"=[], "Reserved"=[]} ("Send"), "ID"=w1565, "RemoteFlag"=w1569, "ExternFlag"=w1568, "DataLen"=u8 3, "Data"=w1564) -> (w1570:T6)
            n770 = Build Array(w1570) -> (w1571:T6[])
            n771 = Unbundle By Name(w1563) -> ("DevType"=w1574:T5, "DevIndex"=w1573:u32, "CanIndex"=w1572:T4)
            n772 = call "VCI_Transmit.vi"("Buffer"=w1571, "CANIndex"=w1572, "DevIndex"=w1573, "DevType"=w1574) -> ()  [unwired: 1 in, 7 out]
          }
          event "T2_W": Value Change {
            w1601 = u8 0 items=["数据帧", "遥控帧"]
            w1602 = u8 0 items=["标准帧", "扩展帧"]
            # "索引地址"
            n773 = event-data() -> ()  [unwired: 2 out]
            n774 = property on="电机ID" class="CmbBox"() -> ("Value"=w1593:string)  [unwired: 2 in, 2 out]
            n775 = Scan From String(format string="%x" ("格式字符串"), input string=w1593, default 1=u8 0) -> (output 1=w1590:u8)  [unwired: 2 in, 3 out]
            n776 = Split Number(x="T2") -> (hi(x)=w1605:u8, lo(x)=w1606:u8)
            n777 = Add(x=u32 16, y=w1590) -> (x+y=w1588:u32)
            n778 = Build Array(u8 101, w1605, w1606) -> (w1587:u8[])
            n779 = Bundle By Name(cluster=T6 {"ID"=0, "TimeStamp"=0, "TimeFlag"=0, "SendType"=0, "RemoteFlag"=0, "ExternFlag"=0, "DataLen"=0, "Data"=[], "Reserved"=[]} ("Send"), "ID"=w1588, "RemoteFlag"=w1601, "ExternFlag"=w1602, "DataLen"=u8 3, "Data"=w1587) -> (w1600:T6)
            n780 = Build Array(w1600) -> (w1599:T6[])
            n781 = Unbundle By Name(w1589) -> ("DevType"=w1596:T5, "DevIndex"=w1597:u32, "CanIndex"=w1598:T4)
            n782 = call "VCI_Transmit.vi"("Buffer"=w1599, "CANIndex"=w1598, "DevIndex"=w1597, "DevType"=w1596) -> ()  [unwired: 1 in, 7 out]
          }
          event "T2_R": Value Change {
            w1615 = u8 0 items=["数据帧", "遥控帧"]
            w1614 = u8 0 items=["标准帧", "扩展帧"]
            # "地址"
            n783 = event-data() -> ()  [unwired: 2 out]
            n784 = property on="电机ID" class="CmbBox"() -> ("Value"=w1624:string)  [unwired: 2 in, 2 out]
            n785 = Scan From String(format string="%x" ("格式字符串"), input string=w1624, default 1=u8 0) -> (output 1=w1627:u8)  [unwired: 2 in, 3 out]
            n786 = call "Demo_MakeData.vi"("DataString"="65") -> ("Data"=w1610:u8[], "DataLen"=w1619:u8)  [unwired: 9 out]
            n787 = Add(x=u32 48, y=w1627) -> (x+y=w1611:u32)
            n788 = Bundle By Name(cluster=T6 {"ID"=0, "TimeStamp"=0, "TimeFlag"=0, "SendType"=0, "RemoteFlag"=0, "ExternFlag"=0, "DataLen"=0, "Data"=[], "Reserved"=[]} ("Send"), "ID"=w1611, "RemoteFlag"=w1615, "ExternFlag"=w1614, "DataLen"=w1619, "Data"=w1610) -> (w1616:T6)
            n789 = Build Array(w1616) -> (w1617:T6[])
            n790 = Unbundle By Name(w1612) -> ("DevType"=w1621:T5, "DevIndex"=w1620:u32, "CanIndex"=w1618:T4)
            n791 = call "VCI_Transmit.vi"("Buffer"=w1617, "CANIndex"=w1618, "DevIndex"=w1620, "DevType"=w1621) -> ()  [unwired: 1 in, 7 out]
          }
          event "T3_W": Value Change {
            w1646 = u8 0 items=["数据帧", "遥控帧"]
            w1647 = u8 0 items=["标准帧", "扩展帧"]
            # "索引地址"
            n792 = event-data() -> ()  [unwired: 2 out]
            n793 = property on="电机ID" class="CmbBox"() -> ("Value"=w1638:string)  [unwired: 2 in, 2 out]
            n794 = Scan From String(format string="%x" ("格式字符串"), input string=w1638, default 1=u8 0) -> (output 1=w1635:u8)  [unwired: 2 in, 3 out]
            n795 = Split Number(x="T3") -> (hi(x)=w1650:u8, lo(x)=w1651:u8)
            n796 = Add(x=u32 16, y=w1635) -> (x+y=w1633:u32)
            n797 = Build Array(u8 102, w1650, w1651) -> (w1632:u8[])
            n798 = Bundle By Name(cluster=T6 {"ID"=0, "TimeStamp"=0, "TimeFlag"=0, "SendType"=0, "RemoteFlag"=0, "ExternFlag"=0, "DataLen"=0, "Data"=[], "Reserved"=[]} ("Send"), "ID"=w1633, "RemoteFlag"=w1646, "ExternFlag"=w1647, "DataLen"=u8 3, "Data"=w1632) -> (w1645:T6)
            n799 = Build Array(w1645) -> (w1644:T6[])
            n800 = Unbundle By Name(w1634) -> ("DevType"=w1641:T5, "DevIndex"=w1642:u32, "CanIndex"=w1643:T4)
            n801 = call "VCI_Transmit.vi"("Buffer"=w1644, "CANIndex"=w1643, "DevIndex"=w1642, "DevType"=w1641) -> ()  [unwired: 1 in, 7 out]
          }
          event "T3_R": Value Change {
            w1670 = u8 0 items=["数据帧", "遥控帧"]
            w1671 = u8 0 items=["标准帧", "扩展帧"]
            # "地址"
            n802 = event-data() -> ()  [unwired: 2 out]
            n803 = property on="电机ID" class="CmbBox"() -> ("Value"=w1661:string)  [unwired: 2 in, 2 out]
            n804 = Scan From String(format string="%x" ("格式字符串"), input string=w1661, default 1=u8 0) -> (output 1=w1658:u8)  [unwired: 2 in, 3 out]
            n805 = call "Demo_MakeData.vi"("DataString"="66") -> ("Data"=w1655:u8[], "DataLen"=w1666:u8)  [unwired: 9 out]
            n806 = Add(x=u32 48, y=w1658) -> (x+y=w1656:u32)
            n807 = Bundle By Name(cluster=T6 {"ID"=0, "TimeStamp"=0, "TimeFlag"=0, "SendType"=0, "RemoteFlag"=0, "ExternFlag"=0, "DataLen"=0, "Data"=[], "Reserved"=[]} ("Send"), "ID"=w1656, "RemoteFlag"=w1670, "ExternFlag"=w1671, "DataLen"=w1666, "Data"=w1655) -> (w1669:T6)
            n808 = Build Array(w1669) -> (w1668:T6[])
            n809 = Unbundle By Name(w1654) -> ("DevType"=w1664:T5, "DevIndex"=w1665:u32, "CanIndex"=w1667:T4)
            n810 = call "VCI_Transmit.vi"("Buffer"=w1668, "CANIndex"=w1667, "DevIndex"=w1665, "DevType"=w1664) -> ()  [unwired: 1 in, 7 out]
          }
          event "T4_W": Value Change {
            w1685 = u8 0 items=["数据帧", "遥控帧"]
            w1684 = u8 0 items=["标准帧", "扩展帧"]
            # "索引地址"
            n811 = event-data() -> ()  [unwired: 2 out]
            n812 = property on="电机ID" class="CmbBox"() -> ("Value"=w1693:string)  [unwired: 2 in, 2 out]
            n813 = Scan From String(format string="%x" ("格式字符串"), input string=w1693, default 1=u8 0) -> (output 1=w1696:u8)  [unwired: 2 in, 3 out]
            n814 = Add(x=u32 16, y=w1696) -> (x+y=w1677:u32)
            n815 = Split Number(x="T4") -> (hi(x)=w1681:u8, lo(x)=w1680:u8)
            n816 = Build Array(u8 103, w1681, w1680) -> (w1676:u8[])
            n817 = Bundle By Name(cluster=T6 {"ID"=0, "TimeStamp"=0, "TimeFlag"=0, "SendType"=0, "RemoteFlag"=0, "ExternFlag"=0, "DataLen"=0, "Data"=[], "Reserved"=[]} ("Send"), "ID"=w1677, "RemoteFlag"=w1685, "ExternFlag"=w1684, "DataLen"=u8 3, "Data"=w1676) -> (w1686:T6)
            n818 = Build Array(w1686) -> (w1687:T6[])
            n819 = Unbundle By Name(w1679) -> ("DevType"=w1690:T5, "DevIndex"=w1689:u32, "CanIndex"=w1688:T4)
            n820 = call "VCI_Transmit.vi"("Buffer"=w1687, "CANIndex"=w1688, "DevIndex"=w1689, "DevType"=w1690) -> ()  [unwired: 1 in, 7 out]
          }
          event "T4_R": Value Change {
            w1715 = u8 0 items=["数据帧", "遥控帧"]
            w1716 = u8 0 items=["标准帧", "扩展帧"]
            # "地址"
            n821 = event-data() -> ()  [unwired: 2 out]
            n822 = property on="电机ID" class="CmbBox"() -> ("Value"=w1706:string)  [unwired: 2 in, 2 out]
            n823 = Scan From String(format string="%x" ("格式字符串"), input string=w1706, default 1=u8 0) -> (output 1=w1703:u8)  [unwired: 2 in, 3 out]
            n824 = call "Demo_MakeData.vi"("DataString"="67") -> ("Data"=w1699:u8[], "DataLen"=w1711:u8)  [unwired: 9 out]
            n825 = Add(x=u32 48, y=w1703) -> (x+y=w1700:u32)
            n826 = Bundle By Name(cluster=T6 {"ID"=0, "TimeStamp"=0, "TimeFlag"=0, "SendType"=0, "RemoteFlag"=0, "ExternFlag"=0, "DataLen"=0, "Data"=[], "Reserved"=[]} ("Send"), "ID"=w1700, "RemoteFlag"=w1715, "ExternFlag"=w1716, "DataLen"=w1711, "Data"=w1699) -> (w1714:T6)
            n827 = Build Array(w1714) -> (w1713:T6[])
            n828 = Unbundle By Name(w1702) -> ("DevType"=w1709:T5, "DevIndex"=w1710:u32, "CanIndex"=w1712:T4)
            n829 = call "VCI_Transmit.vi"("Buffer"=w1713, "CANIndex"=w1712, "DevIndex"=w1710, "DevType"=w1709) -> ()  [unwired: 1 in, 7 out]
          }
          event "Direction_W": Value Change {
            w1727 = u8 0 items=["数据帧", "遥控帧"]
            w1726 = u8 0 items=["标准帧", "扩展帧"]
            # "索引地址"
            n830 = event-data() -> ()  [unwired: 2 out]
            n831 = property on="电机ID" class="CmbBox"() -> ("Value"=w1735:string)  [unwired: 2 in, 2 out]
            n832 = Scan From String(format string="%x" ("格式字符串"), input string=w1735, default 1=u8 0) -> (output 1=w1738:u8)  [unwired: 2 in, 3 out]
            n833 = Add(x=u32 16, y=w1738) -> (x+y=w1724:u32)
            n834 = Build Array(u8 106, "方向") -> (w1723:u16[])
            n835 = Bundle By Name(cluster=T6 {"ID"=0, "TimeStamp"=0, "TimeFlag"=0, "SendType"=0, "RemoteFlag"=0, "ExternFlag"=0, "DataLen"=0, "Data"=[], "Reserved"=[]} ("Send"), "ID"=w1724, "RemoteFlag"=w1727, "ExternFlag"=w1726, "DataLen"=u8 2, "Data"=w1723) -> (w1728:T6)
            n836 = Build Array(w1728) -> (w1729:T6[])
            n837 = Unbundle By Name(w1721) -> ("DevType"=w1732:T5, "DevIndex"=w1731:u32, "CanIndex"=w1730:T4)
            n838 = call "VCI_Transmit.vi"("Buffer"=w1729, "CANIndex"=w1730, "DevIndex"=w1731, "DevType"=w1732) -> ()  [unwired: 1 in, 7 out]
          }
          event "Direction_R": Value Change {
            w1748 = u8 0 items=["数据帧", "遥控帧"]
            w1747 = u8 0 items=["标准帧", "扩展帧"]
            # "地址"
            n839 = event-data() -> ()  [unwired: 2 out]
            n840 = property on="电机ID" class="CmbBox"() -> ("Value"=w1757:string)  [unwired: 2 in, 2 out]
            n841 = Scan From String(format string="%x" ("格式字符串"), input string=w1757, default 1=u8 0) -> (output 1=w1760:u8)  [unwired: 2 in, 3 out]
            n842 = call "Demo_MakeData.vi"("DataString"="6A ") -> ("Data"=w1743:u8[], "DataLen"=w1752:u8)  [unwired: 9 out]
            n843 = Add(x=u32 48, y=w1760) -> (x+y=w1744:u32)
            n844 = Bundle By Name(cluster=T6 {"ID"=0, "TimeStamp"=0, "TimeFlag"=0, "SendType"=0, "RemoteFlag"=0, "ExternFlag"=0, "DataLen"=0, "Data"=[], "Reserved"=[]} ("Send"), "ID"=w1744, "RemoteFlag"=w1748, "ExternFlag"=w1747, "DataLen"=w1752, "Data"=w1743) -> (w1749:T6)
            n845 = Build Array(w1749) -> (w1750:T6[])
            n846 = Unbundle By Name(w1742) -> ("DevType"=w1754:T5, "DevIndex"=w1753:u32, "CanIndex"=w1751:T4)
            n847 = call "VCI_Transmit.vi"("Buffer"=w1750, "CANIndex"=w1751, "DevIndex"=w1753, "DevType"=w1754) -> ()  [unwired: 1 in, 7 out]
          }
          event "W_EN_W": Value Change {
            w1779 = u8 0 items=["数据帧", "遥控帧"]
            w1780 = u8 0 items=["标准帧", "扩展帧"]
            # "索引地址"
            n848 = event-data() -> ()  [unwired: 2 out]
            n849 = property on="电机ID" class="CmbBox"() -> ("Value"=w1771:string)  [unwired: 2 in, 2 out]
            n850 = Scan From String(format string="%x" ("格式字符串"), input string=w1771, default 1=u8 0) -> (output 1=w1768:u8)  [unwired: 2 in, 3 out]
            n851 = Add(x=u32 16, y=w1768) -> (x+y=w1766:u32)
            n852 = Build Array(u8 105, "过载诊断") -> (w1765:u8[])
            n853 = Bundle By Name(cluster=T6 {"ID"=0, "TimeStamp"=0, "TimeFlag"=0, "SendType"=0, "RemoteFlag"=0, "ExternFlag"=0, "DataLen"=0, "Data"=[], "Reserved"=[]} ("Send"), "ID"=w1766, "RemoteFlag"=w1779, "ExternFlag"=w1780, "DataLen"=u8 2, "Data"=w1765) -> (w1778:T6)
            n854 = Build Array(w1778) -> (w1777:T6[])
            n855 = Unbundle By Name(w1767) -> ("DevType"=w1774:T5, "DevIndex"=w1775:u32, "CanIndex"=w1776:T4)
            n856 = call "VCI_Transmit.vi"("Buffer"=w1777, "CANIndex"=w1776, "DevIndex"=w1775, "DevType"=w1774) -> ()  [unwired: 1 in, 7 out]
          }
          event "W_EN_R": Value Change {
            w1800 = u8 0 items=["数据帧", "遥控帧"]
            w1801 = u8 0 items=["标准帧", "扩展帧"]
            # "地址"
            n857 = event-data() -> ()  [unwired: 2 out]
            n858 = property on="电机ID" class="CmbBox"() -> ("Value"=w1792:string)  [unwired: 2 in, 2 out]
            n859 = Scan From String(format string="%x" ("格式字符串"), input string=w1792, default 1=u8 0) -> (output 1=w1789:u8)  [unwired: 2 in, 3 out]
            n860 = call "Demo_MakeData.vi"("DataString"="69 ") -> ("Data"=w1786:u8[], "DataLen"=w1803:u8)  [unwired: 9 out]
            n861 = Add(x=u32 48, y=w1789) -> (x+y=w1787:u32)
            n862 = Bundle By Name(cluster=T6 {"ID"=0, "TimeStamp"=0, "TimeFlag"=0, "SendType"=0, "RemoteFlag"=0, "ExternFlag"=0, "DataLen"=0, "Data"=[], "Reserved"=[]} ("Send"), "ID"=w1787, "RemoteFlag"=w1800, "ExternFlag"=w1801, "DataLen"=w1803, "Data"=w1786) -> (w1799:T6)
            n863 = Build Array(w1799) -> (w1798:T6[])
            n864 = Unbundle By Name(w1788) -> ("DevType"=w1795:T5, "DevIndex"=w1796:u32, "CanIndex"=w1797:T4)
            n865 = call "VCI_Transmit.vi"("Buffer"=w1798, "CANIndex"=w1797, "DevIndex"=w1796, "DevType"=w1795) -> ()  [unwired: 1 in, 7 out]
          }
          event "I_EN_W": Value Change {
            w1822 = u8 0 items=["数据帧", "遥控帧"]
            w1823 = u8 0 items=["标准帧", "扩展帧"]
            # "索引地址"
            n866 = event-data() -> ()  [unwired: 2 out]
            n867 = property on="电机ID" class="CmbBox"() -> ("Value"=w1814:string)  [unwired: 2 in, 2 out]
            n868 = Scan From String(format string="%x" ("格式字符串"), input string=w1814, default 1=u8 0) -> (output 1=w1811:u8)  [unwired: 2 in, 3 out]
            n869 = Add(x=u32 16, y=w1811) -> (x+y=w1810:u32)
            n870 = Build Array(u8 104, "电流诊断") -> (w1809:u8[])
            n871 = Bundle By Name(cluster=T6 {"ID"=0, "TimeStamp"=0, "TimeFlag"=0, "SendType"=0, "RemoteFlag"=0, "ExternFlag"=0, "DataLen"=0, "Data"=[], "Reserved"=[]} ("Send"), "ID"=w1810, "RemoteFlag"=w1822, "ExternFlag"=w1823, "DataLen"=u8 2, "Data"=w1809) -> (w1821:T6)
            n872 = Build Array(w1821) -> (w1820:T6[])
            n873 = Unbundle By Name(w1807) -> ("DevType"=w1817:T5, "DevIndex"=w1818:u32, "CanIndex"=w1819:T4)
            n874 = call "VCI_Transmit.vi"("Buffer"=w1820, "CANIndex"=w1819, "DevIndex"=w1818, "DevType"=w1817) -> ()  [unwired: 1 in, 7 out]
          }
          event "I_EN_R": Value Change {
            w1834 = u8 0 items=["数据帧", "遥控帧"]
            w1833 = u8 0 items=["标准帧", "扩展帧"]
            # "地址"
            n875 = event-data() -> ()  [unwired: 2 out]
            n876 = property on="电机ID" class="CmbBox"() -> ("Value"=w1843:string)  [unwired: 2 in, 2 out]
            n877 = Scan From String(format string="%x" ("格式字符串"), input string=w1843, default 1=u8 0) -> (output 1=w1846:u8)  [unwired: 2 in, 3 out]
            n878 = call "Demo_MakeData.vi"("DataString"="68 ") -> ("Data"=w1829:u8[], "DataLen"=w1838:u8)  [unwired: 9 out]
            n879 = Add(x=u32 48, y=w1846) -> (x+y=w1830:u32)
            n880 = Bundle By Name(cluster=T6 {"ID"=0, "TimeStamp"=0, "TimeFlag"=0, "SendType"=0, "RemoteFlag"=0, "ExternFlag"=0, "DataLen"=0, "Data"=[], "Reserved"=[]} ("Send"), "ID"=w1830, "RemoteFlag"=w1834, "ExternFlag"=w1833, "DataLen"=w1838, "Data"=w1829) -> (w1835:T6)
            n881 = Build Array(w1835) -> (w1836:T6[])
            n882 = Unbundle By Name(w1828) -> ("DevType"=w1840:T5, "DevIndex"=w1839:u32, "CanIndex"=w1837:T4)
            n883 = call "VCI_Transmit.vi"("Buffer"=w1836, "CANIndex"=w1837, "DevIndex"=w1839, "DevType"=w1840) -> ()  [unwired: 1 in, 7 out]
          }
          event "位置环KP_W": Value Change {
            w1861 = u8 0 items=["数据帧", "遥控帧"]
            w1860 = u8 0 items=["标准帧", "扩展帧"]
            # "索引地址"
            n884 = event-data() -> ()  [unwired: 2 out]
            n885 = property on="电机ID" class="CmbBox"() -> ("Value"=w1869:string)  [unwired: 2 in, 2 out]
            n886 = Multiply ("乘")(x="位置环KP", y=u16 256) -> (x*y=w1856:u16)
            n887 = Scan From String(format string="%x" ("格式字符串"), input string=w1869, default 1=u8 0) -> (output 1=w1872:u8)  [unwired: 2 in, 3 out]
            n888 = Split Number(x=w1856) -> (hi(x)=w1855:u8, lo(x)=w1854:u8)
            n889 = Add(x=u32 16, y=w1872) -> (x+y=w1852:u32)
            n890 = Build Array(u8 107, w1855, w1854) -> (w1851:u8[])
            n891 = Bundle By Name(cluster=T6 {"ID"=0, "TimeStamp"=0, "TimeFlag"=0, "SendType"=0, "RemoteFlag"=0, "ExternFlag"=0, "DataLen"=0, "Data"=[], "Reserved"=[]} ("Send"), "ID"=w1852, "RemoteFlag"=w1861, "ExternFlag"=w1860, "DataLen"=u8 3, "Data"=w1851) -> (w1862:T6)
            n892 = Build Array(w1862) -> (w1863:T6[])
            n893 = Unbundle By Name(w1853) -> ("DevType"=w1866:T5, "DevIndex"=w1865:u32, "CanIndex"=w1864:T4)
            n894 = call "VCI_Transmit.vi"("Buffer"=w1863, "CANIndex"=w1864, "DevIndex"=w1865, "DevType"=w1866) -> ()  [unwired: 1 in, 7 out]
          }
          event "位置环KP_R": Value Change {
            w1891 = u8 0 items=["数据帧", "遥控帧"]
            w1892 = u8 0 items=["标准帧", "扩展帧"]
            # "地址"
            n895 = event-data() -> ()  [unwired: 2 out]
            n896 = property on="电机ID" class="CmbBox"() -> ("Value"=w1882:string)  [unwired: 2 in, 2 out]
            n897 = Scan From String(format string="%x" ("格式字符串"), input string=w1882, default 1=u8 0) -> (output 1=w1879:u8)  [unwired: 2 in, 3 out]
            n898 = call "Demo_MakeData.vi"("DataString"="6B ") -> ("Data"=w1876:u8[], "DataLen"=w1887:u8)  [unwired: 9 out]
            n899 = Add(x=u32 48, y=w1879) -> (x+y=w1877:u32)
            n900 = Bundle By Name(cluster=T6 {"ID"=0, "TimeStamp"=0, "TimeFlag"=0, "SendType"=0, "RemoteFlag"=0, "ExternFlag"=0, "DataLen"=0, "Data"=[], "Reserved"=[]} ("Send"), "ID"=w1877, "RemoteFlag"=w1891, "ExternFlag"=w1892, "DataLen"=w1887, "Data"=w1876) -> (w1890:T6)
            n901 = Build Array(w1890) -> (w1889:T6[])
            n902 = Unbundle By Name(w1878) -> ("DevType"=w1885:T5, "DevIndex"=w1886:u32, "CanIndex"=w1888:T4)
            n903 = call "VCI_Transmit.vi"("Buffer"=w1889, "CANIndex"=w1888, "DevIndex"=w1886, "DevType"=w1885) -> ()  [unwired: 1 in, 7 out]
          }
          event "位置环KI_W": Value Change {
            w1908 = u8 0 items=["数据帧", "遥控帧"]
            w1907 = u8 0 items=["标准帧", "扩展帧"]
            # "索引地址"
            n904 = event-data() -> ()  [unwired: 2 out]
            n905 = property on="电机ID" class="CmbBox"() -> ("Value"=w1916:string)  [unwired: 2 in, 2 out]
            n906 = Multiply ("乘")(x="位置环KI", y=u16 256) -> (x*y=w1903:u16)
            n907 = Scan From String(format string="%x" ("格式字符串"), input string=w1916, default 1=u8 0) -> (output 1=w1919:u8)  [unwired: 2 in, 3 out]
            n908 = Split Number(x=w1903) -> (hi(x)=w1902:u8, lo(x)=w1901:u8)
            n909 = Add(x=u32 16, y=w1919) -> (x+y=w1899:u32)
            n910 = Build Array(u8 108, w1902, w1901) -> (w1898:u8[])
            n911 = Bundle By Name(cluster=T6 {"ID"=0, "TimeStamp"=0, "TimeFlag"=0, "SendType"=0, "RemoteFlag"=0, "ExternFlag"=0, "DataLen"=0, "Data"=[], "Reserved"=[]} ("Send"), "ID"=w1899, "RemoteFlag"=w1908, "ExternFlag"=w1907, "DataLen"=u8 3, "Data"=w1898) -> (w1909:T6)
            n912 = Build Array(w1909) -> (w1910:T6[])
            n913 = Unbundle By Name(w1900) -> ("DevType"=w1913:T5, "DevIndex"=w1912:u32, "CanIndex"=w1911:T4)
            n914 = call "VCI_Transmit.vi"("Buffer"=w1910, "CANIndex"=w1911, "DevIndex"=w1912, "DevType"=w1913) -> ()  [unwired: 1 in, 7 out]
          }
          event "位置环KI_R": Value Change {
            w1938 = u8 0 items=["数据帧", "遥控帧"]
            w1939 = u8 0 items=["标准帧", "扩展帧"]
            # "地址"
            n915 = event-data() -> ()  [unwired: 2 out]
            n916 = property on="电机ID" class="CmbBox"() -> ("Value"=w1929:string)  [unwired: 2 in, 2 out]
            n917 = Scan From String(format string="%x" ("格式字符串"), input string=w1929, default 1=u8 0) -> (output 1=w1926:u8)  [unwired: 2 in, 3 out]
            n918 = call "Demo_MakeData.vi"("DataString"="6C ") -> ("Data"=w1923:u8[], "DataLen"=w1934:u8)  [unwired: 9 out]
            n919 = Add(x=u32 48, y=w1926) -> (x+y=w1924:u32)
            n920 = Bundle By Name(cluster=T6 {"ID"=0, "TimeStamp"=0, "TimeFlag"=0, "SendType"=0, "RemoteFlag"=0, "ExternFlag"=0, "DataLen"=0, "Data"=[], "Reserved"=[]} ("Send"), "ID"=w1924, "RemoteFlag"=w1938, "ExternFlag"=w1939, "DataLen"=w1934, "Data"=w1923) -> (w1937:T6)
            n921 = Build Array(w1937) -> (w1936:T6[])
            n922 = Unbundle By Name(w1925) -> ("DevType"=w1932:T5, "DevIndex"=w1933:u32, "CanIndex"=w1935:T4)
            n923 = call "VCI_Transmit.vi"("Buffer"=w1936, "CANIndex"=w1935, "DevIndex"=w1933, "DevType"=w1932) -> ()  [unwired: 1 in, 7 out]
          }
          event "电压限制_W": Value Change {
            w1954 = u8 0 items=["数据帧", "遥控帧"]
            w1953 = u8 0 items=["标准帧", "扩展帧"]
            # "索引地址"
            n924 = event-data() -> ()  [unwired: 2 out]
            n925 = property on="电机ID" class="CmbBox"() -> ("Value"=w1962:string)  [unwired: 2 in, 2 out]
            n926 = Multiply ("乘")(x="电压限制", y=i16 8) -> (x*y=w1950:i16)
            n927 = Scan From String(format string="%x" ("格式字符串"), input string=w1962, default 1=u8 0) -> (output 1=w1965:u8)  [unwired: 2 in, 3 out]
            n928 = Absolute Value(x=w1950) -> (abs(x)=w1948:i16)
            n929 = Add(x=u32 16, y=w1965) -> (x+y=w1946:u32)
            n930 = Split Number(x=w1948) -> (hi(x)=w1966:u8, lo(x)=w1967:u8)
            n931 = Build Array(u8 109, w1966, w1967) -> (w1945:u8[])
            n932 = Bundle By Name(cluster=T6 {"ID"=0, "TimeStamp"=0, "TimeFlag"=0, "SendType"=0, "RemoteFlag"=0, "ExternFlag"=0, "DataLen"=0, "Data"=[], "Reserved"=[]} ("Send"), "ID"=w1946, "RemoteFlag"=w1954, "ExternFlag"=w1953, "DataLen"=u8 3, "Data"=w1945) -> (w1955:T6)
            n933 = Build Array(w1955) -> (w1956:T6[])
            n934 = Unbundle By Name(w1947) -> ("DevType"=w1959:T5, "DevIndex"=w1958:u32, "CanIndex"=w1957:T4)
            n935 = call "VCI_Transmit.vi"("Buffer"=w1956, "CANIndex"=w1957, "DevIndex"=w1958, "DevType"=w1959) -> ()  [unwired: 1 in, 7 out]
          }
          event "电压限制_R": Value Change {
            w1986 = u8 0 items=["数据帧", "遥控帧"]
            w1987 = u8 0 items=["标准帧", "扩展帧"]
            # "地址"
            n936 = event-data() -> ()  [unwired: 2 out]
            n937 = property on="电机ID" class="CmbBox"() -> ("Value"=w1977:string)  [unwired: 2 in, 2 out]
            n938 = Scan From String(format string="%x" ("格式字符串"), input string=w1977, default 1=u8 0) -> (output 1=w1974:u8)  [unwired: 2 in, 3 out]
            n939 = call "Demo_MakeData.vi"("DataString"="6d ") -> ("Data"=w1972:u8[], "DataLen"=w1982:u8)  [unwired: 9 out]
            n940 = Add(x=u32 48, y=w1974) -> (x+y=w1973:u32)
            n941 = Bundle By Name(cluster=T6 {"ID"=0, "TimeStamp"=0, "TimeFlag"=0, "SendType"=0, "RemoteFlag"=0, "ExternFlag"=0, "DataLen"=0, "Data"=[], "Reserved"=[]} ("Send"), "ID"=w1973, "RemoteFlag"=w1986, "ExternFlag"=w1987, "DataLen"=w1982, "Data"=w1972) -> (w1985:T6)
            n942 = Build Array(w1985) -> (w1984:T6[])
            n943 = Unbundle By Name(w1971) -> ("DevType"=w1980:T5, "DevIndex"=w1981:u32, "CanIndex"=w1983:T4)
            n944 = call "VCI_Transmit.vi"("Buffer"=w1984, "CANIndex"=w1983, "DevIndex"=w1981, "DevType"=w1980) -> ()  [unwired: 1 in, 7 out]
          }
          event "上限位_R": Value Change {
            w1997 = u8 0 items=["数据帧", "遥控帧"]
            w1996 = u8 0 items=["标准帧", "扩展帧"]
            # "地址"
            n945 = event-data() -> ()  [unwired: 2 out]
            n946 = property on="电机ID" class="CmbBox"() -> ("Value"=w2006:string)  [unwired: 2 in, 2 out]
            n947 = Scan From String(format string="%x" ("格式字符串"), input string=w2006, default 1=u8 0) -> (output 1=w2009:u8)  [unwired: 2 in, 3 out]
            n948 = call "Demo_MakeData.vi"("DataString"="6E") -> ("Data"=w1992:u8[], "DataLen"=w2001:u8)  [unwired: 9 out]
            n949 = Add(x=u32 48, y=w2009) -> (x+y=w1993:u32)
            n950 = Bundle By Name(cluster=T6 {"ID"=0, "TimeStamp"=0, "TimeFlag"=0, "SendType"=0, "RemoteFlag"=0, "ExternFlag"=0, "DataLen"=0, "Data"=[], "Reserved"=[]} ("Send"), "ID"=w1993, "RemoteFlag"=w1997, "ExternFlag"=w1996, "DataLen"=w2001, "Data"=w1992) -> (w1998:T6)
            n951 = Build Array(w1998) -> (w1999:T6[])
            n952 = Unbundle By Name(w1994) -> ("DevType"=w2003:T5, "DevIndex"=w2002:u32, "CanIndex"=w2000:T4)
            n953 = call "VCI_Transmit.vi"("Buffer"=w1999, "CANIndex"=w2000, "DevIndex"=w2002, "DevType"=w2003) -> ()  [unwired: 1 in, 7 out]
          }
          event "下限位_W": Value Change {
            w2024 = u8 0 items=["数据帧", "遥控帧"]
            w2023 = u8 0 items=["标准帧", "扩展帧"]
            # "索引地址"
            n954 = event-data() -> ()  [unwired: 2 out]
            n955 = Multiply ("乘")(x="下限", y=1) -> (x*y=w2018:i16)
            n956 = property on="电机ID" class="CmbBox"() -> ("Value"=w2032:string)  [unwired: 2 in, 2 out]
            n957 = Split Number(x=w2018) -> (hi(x)=w2017:u8, lo(x)=w2016:u8)
            n958 = Scan From String(format string="%x" ("格式字符串"), input string=w2032, default 1=u8 0) -> (output 1=w2035:u8)  [unwired: 2 in, 3 out]
            n959 = Add(x=u32 16, y=w2035) -> (x+y=w2020:u32)
            n960 = Build Array(u8 111, w2017, w2016) -> (w2015:u8[])
            n961 = Bundle By Name(cluster=T6 {"ID"=0, "TimeStamp"=0, "TimeFlag"=0, "SendType"=0, "RemoteFlag"=0, "ExternFlag"=0, "DataLen"=0, "Data"=[], "Reserved"=[]} ("Send"), "ID"=w2020, "RemoteFlag"=w2024, "ExternFlag"=w2023, "DataLen"=u8 3, "Data"=w2015) -> (w2025:T6)
            n962 = Build Array(w2025) -> (w2026:T6[])
            n963 = Unbundle By Name(w2021) -> ("DevType"=w2029:T5, "DevIndex"=w2028:u32, "CanIndex"=w2027:T4)
            n964 = call "VCI_Transmit.vi"("Buffer"=w2026, "CANIndex"=w2027, "DevIndex"=w2028, "DevType"=w2029) -> ()  [unwired: 1 in, 7 out]
          }
          event "下限位R": Value Change {
            w2054 = u8 0 items=["数据帧", "遥控帧"]
            w2055 = u8 0 items=["标准帧", "扩展帧"]
            # "地址"
            n965 = event-data() -> ()  [unwired: 2 out]
            n966 = property on="电机ID" class="CmbBox"() -> ("Value"=w2045:string)  [unwired: 2 in, 2 out]
            n967 = Scan From String(format string="%x" ("格式字符串"), input string=w2045, default 1=u8 0) -> (output 1=w2042:u8)  [unwired: 2 in, 3 out]
            n968 = call "Demo_MakeData.vi"("DataString"="6F") -> ("Data"=w2040:u8[], "DataLen"=w2050:u8)  [unwired: 9 out]
            n969 = Add(x=u32 48, y=w2042) -> (x+y=w2041:u32)
            n970 = Bundle By Name(cluster=T6 {"ID"=0, "TimeStamp"=0, "TimeFlag"=0, "SendType"=0, "RemoteFlag"=0, "ExternFlag"=0, "DataLen"=0, "Data"=[], "Reserved"=[]} ("Send"), "ID"=w2041, "RemoteFlag"=w2054, "ExternFlag"=w2055, "DataLen"=w2050, "Data"=w2040) -> (w2053:T6)
            n971 = Build Array(w2053) -> (w2052:T6[])
            n972 = Unbundle By Name(w2038) -> ("DevType"=w2048:T5, "DevIndex"=w2049:u32, "CanIndex"=w2051:T4)
            n973 = call "VCI_Transmit.vi"("Buffer"=w2052, "CANIndex"=w2051, "DevIndex"=w2049, "DevType"=w2048) -> ()  [unwired: 1 in, 7 out]
          }
          event "Kt_W": Value Change {
            w2071 = u8 0 items=["数据帧", "遥控帧"]
            w2070 = u8 0 items=["标准帧", "扩展帧"]
            # "索引地址"
            n974 = event-data() -> ()  [unwired: 2 out]
            n975 = property on="电机ID" class="CmbBox"() -> ("Value"=w2079:string)  [unwired: 2 in, 2 out]
            n976 = Multiply ("乘")(x="Kt", y=u16 256) -> (x*y=w2066:u16)
            n977 = Scan From String(format string="%x" ("格式字符串"), input string=w2079, default 1=u8 0) -> (output 1=w2082:u8)  [unwired: 2 in, 3 out]
            n978 = Split Number(x=w2066) -> (hi(x)=w2065:u8, lo(x)=w2064:u8)
            n979 = Add(x=u32 16, y=w2082) -> (x+y=w2062:u32)
            n980 = Build Array(u8 112, w2065, w2064) -> (w2061:u8[])
            n981 = Bundle By Name(cluster=T6 {"ID"=0, "TimeStamp"=0, "TimeFlag"=0, "SendType"=0, "RemoteFlag"=0, "ExternFlag"=0, "DataLen"=0, "Data"=[], "Reserved"=[]} ("Send"), "ID"=w2062, "RemoteFlag"=w2071, "ExternFlag"=w2070, "DataLen"=u8 3, "Data"=w2061) -> (w2072:T6)
            n982 = Build Array(w2072) -> (w2073:T6[])
            n983 = Unbundle By Name(w2063) -> ("DevType"=w2076:T5, "DevIndex"=w2075:u32, "CanIndex"=w2074:T4)
            n984 = call "VCI_Transmit.vi"("Buffer"=w2073, "CANIndex"=w2074, "DevIndex"=w2075, "DevType"=w2076) -> ()  [unwired: 1 in, 7 out]
          }
          event "Servo_EN_W": Value Change {
            w2101 = u8 0 items=["数据帧", "遥控帧"]
            w2102 = u8 0 items=["标准帧", "扩展帧"]
            # "索引地址"
            n985 = event-data() -> ()  [unwired: 2 out]
            n986 = property on="电机ID" class="CmbBox"() -> ("Value"=w2093:string)  [unwired: 2 in, 2 out]
            n987 = Scan From String(format string="%x" ("格式字符串"), input string=w2093, default 1=u8 0) -> (output 1=w2090:u8)  [unwired: 2 in, 3 out]
            n988 = Add(x=u32 16, y=w2090) -> (x+y=w2088:u32)
            n989 = Build Array(u8 114, "伺服En") -> (w2087:u8[])
            n990 = Bundle By Name(cluster=T6 {"ID"=0, "TimeStamp"=0, "TimeFlag"=0, "SendType"=0, "RemoteFlag"=0, "ExternFlag"=0, "DataLen"=0, "Data"=[], "Reserved"=[]} ("Send"), "ID"=w2088, "RemoteFlag"=w2101, "ExternFlag"=w2102, "DataLen"=u8 2, "Data"=w2087) -> (w2100:T6)
            n991 = Build Array(w2100) -> (w2099:T6[])
            n992 = Unbundle By Name(w2089) -> ("DevType"=w2096:T5, "DevIndex"=w2097:u32, "CanIndex"=w2098:T4)
            n993 = call "VCI_Transmit.vi"("Buffer"=w2099, "CANIndex"=w2098, "DevIndex"=w2097, "DevType"=w2096) -> ()  [unwired: 1 in, 7 out]
          }
          event "Servo_EN_R": Value Change {
            w2123 = u8 0 items=["数据帧", "遥控帧"]
            w2124 = u8 0 items=["标准帧", "扩展帧"]
            # "地址"
            n994 = event-data() -> ()  [unwired: 2 out]
            n995 = property on="电机ID" class="CmbBox"() -> ("Value"=w2114:string)  [unwired: 2 in, 2 out]
            n996 = Scan From String(format string="%x" ("格式字符串"), input string=w2114, default 1=u8 0) -> (output 1=w2111:u8)  [unwired: 2 in, 3 out]
            n997 = call "Demo_MakeData.vi"("DataString"="72") -> ("Data"=w2108:u8[], "DataLen"=w2119:u8)  [unwired: 9 out]
            n998 = Add(x=u32 48, y=w2111) -> (x+y=w2109:u32)
            n999 = Bundle By Name(cluster=T6 {"ID"=0, "TimeStamp"=0, "TimeFlag"=0, "SendType"=0, "RemoteFlag"=0, "ExternFlag"=0, "DataLen"=0, "Data"=[], "Reserved"=[]} ("Send"), "ID"=w2109, "RemoteFlag"=w2123, "ExternFlag"=w2124, "DataLen"=w2119, "Data"=w2108) -> (w2122:T6)
            n1000 = Build Array(w2122) -> (w2121:T6[])
            n1001 = Unbundle By Name(w2110) -> ("DevType"=w2117:T5, "DevIndex"=w2118:u32, "CanIndex"=w2120:T4)
            n1002 = call "VCI_Transmit.vi"("Buffer"=w2121, "CANIndex"=w2120, "DevIndex"=w2118, "DevType"=w2117) -> ()  [unwired: 1 in, 7 out]
          }
          event "Kt_R": Value Change {
            w2144 = u8 0 items=["数据帧", "遥控帧"]
            w2145 = u8 0 items=["标准帧", "扩展帧"]
            # "地址"
            n1003 = event-data() -> ()  [unwired: 2 out]
            n1004 = property on="电机ID" class="CmbBox"() -> ("Value"=w2135:string)  [unwired: 2 in, 2 out]
            n1005 = Scan From String(format string="%x" ("格式字符串"), input string=w2135, default 1=u8 0) -> (output 1=w2132:u8)  [unwired: 2 in, 3 out]
            n1006 = call "Demo_MakeData.vi"("DataString"="70") -> ("Data"=w2129:u8[], "DataLen"=w2140:u8)  [unwired: 9 out]
            n1007 = Add(x=u32 48, y=w2132) -> (x+y=w2130:u32)
            n1008 = Bundle By Name(cluster=T6 {"ID"=0, "TimeStamp"=0, "TimeFlag"=0, "SendType"=0, "RemoteFlag"=0, "ExternFlag"=0, "DataLen"=0, "Data"=[], "Reserved"=[]} ("Send"), "ID"=w2130, "RemoteFlag"=w2144, "ExternFlag"=w2145, "DataLen"=w2140, "Data"=w2129) -> (w2143:T6)
            n1009 = Build Array(w2143) -> (w2142:T6[])
            n1010 = Unbundle By Name(w2131) -> ("DevType"=w2138:T5, "DevIndex"=w2139:u32, "CanIndex"=w2141:T4)
            n1011 = call "VCI_Transmit.vi"("Buffer"=w2142, "CANIndex"=w2141, "DevIndex"=w2139, "DevType"=w2138) -> ()  [unwired: 1 in, 7 out]
          }
          event "Gear_W": Value Change {
            w2165 = u8 0 items=["数据帧", "遥控帧"]
            w2166 = u8 0 items=["标准帧", "扩展帧"]
            # "索引地址"
            n1012 = event-data() -> ()  [unwired: 2 out]
            n1013 = property on="电机ID" class="CmbBox"() -> ("Value"=w2157:string)  [unwired: 2 in, 2 out]
            n1014 = Multiply ("乘")(x="Gear", y=u16 1) -> (x*y=w2170:u16)
            n1015 = Scan From String(format string="%x" ("格式字符串"), input string=w2157, default 1=u8 0) -> (output 1=w2154:u8)  [unwired: 2 in, 3 out]
            n1016 = Split Number(x=w2170) -> (hi(x)=w2171:u8, lo(x)=w2172:u8)
            n1017 = Add(x=u32 16, y=w2154) -> (x+y=w2153:u32)
            n1018 = Build Array(u8 113, w2171, w2172) -> (w2152:u8[])
            n1019 = Bundle By Name(cluster=T6 {"ID"=0, "TimeStamp"=0, "TimeFlag"=0, "SendType"=0, "RemoteFlag"=0, "ExternFlag"=0, "DataLen"=0, "Data"=[], "Reserved"=[]} ("Send"), "ID"=w2153, "RemoteFlag"=w2165, "ExternFlag"=w2166, "DataLen"=u8 3, "Data"=w2152) -> (w2164:T6)
            n1020 = Build Array(w2164) -> (w2163:T6[])
            n1021 = Unbundle By Name(w2151) -> ("DevType"=w2160:T5, "DevIndex"=w2161:u32, "CanIndex"=w2162:T4)
            n1022 = call "VCI_Transmit.vi"("Buffer"=w2163, "CANIndex"=w2162, "DevIndex"=w2161, "DevType"=w2160) -> ()  [unwired: 1 in, 7 out]
          }
          event "Gear_R": Value Change {
            w2181 = u8 0 items=["数据帧", "遥控帧"]
            w2180 = u8 0 items=["标准帧", "扩展帧"]
            # "地址"
            n1023 = event-data() -> ()  [unwired: 2 out]
            n1024 = property on="电机ID" class="CmbBox"() -> ("Value"=w2190:string)  [unwired: 2 in, 2 out]
            n1025 = Scan From String(format string="%x" ("格式字符串"), input string=w2190, default 1=u8 0) -> (output 1=w2193:u8)  [unwired: 2 in, 3 out]
            n1026 = call "Demo_MakeData.vi"("DataString"="71") -> ("Data"=w2176:u8[], "DataLen"=w2185:u8)  [unwired: 9 out]
            n1027 = Add(x=u32 48, y=w2193) -> (x+y=w2177:u32)
            n1028 = Bundle By Name(cluster=T6 {"ID"=0, "TimeStamp"=0, "TimeFlag"=0, "SendType"=0, "RemoteFlag"=0, "ExternFlag"=0, "DataLen"=0, "Data"=[], "Reserved"=[]} ("Send"), "ID"=w2177, "RemoteFlag"=w2181, "ExternFlag"=w2180, "DataLen"=w2185, "Data"=w2176) -> (w2182:T6)
            n1029 = Build Array(w2182) -> (w2183:T6[])
            n1030 = Unbundle By Name(w2178) -> ("DevType"=w2187:T5, "DevIndex"=w2186:u32, "CanIndex"=w2184:T4)
            n1031 = call "VCI_Transmit.vi"("Buffer"=w2183, "CANIndex"=w2184, "DevIndex"=w2186, "DevType"=w2187) -> ()  [unwired: 1 in, 7 out]
          }
          event "Servo_Count_W": Value Change {
            w2212 = u8 0 items=["数据帧", "遥控帧"]
            w2213 = u8 0 items=["标准帧", "扩展帧"]
            # "索引地址"
            n1032 = event-data() -> ()  [unwired: 2 out]
            n1033 = property on="电机ID" class="CmbBox"() -> ("Value"=w2204:string)  [unwired: 2 in, 2 out]
            n1034 = Scan From String(format string="%x" ("格式字符串"), input string=w2204, default 1=u8 0) -> (output 1=w2201:u8)  [unwired: 2 in, 3 out]
            n1035 = Add(x=u32 16, y=w2201) -> (x+y=w2199:u32)
            n1036 = Split Number(x="伺服频率") -> (hi(x)=w2216:u8, lo(x)=w2217:u8)
            n1037 = Build Array(u8 115, w2216, w2217) -> (w2198:u8[])
            n1038 = Bundle By Name(cluster=T6 {"ID"=0, "TimeStamp"=0, "TimeFlag"=0, "SendType"=0, "RemoteFlag"=0, "ExternFlag"=0, "DataLen"=0, "Data"=[], "Reserved"=[]} ("Send"), "ID"=w2199, "RemoteFlag"=w2212, "ExternFlag"=w2213, "DataLen"=u8 3, "Data"=w2198) -> (w2211:T6)
            n1039 = Build Array(w2211) -> (w2210:T6[])
            n1040 = Unbundle By Name(w2200) -> ("DevType"=w2207:T5, "DevIndex"=w2208:u32, "CanIndex"=w2209:T4)
            n1041 = call "VCI_Transmit.vi"("Buffer"=w2210, "CANIndex"=w2209, "DevIndex"=w2208, "DevType"=w2207) -> ()  [unwired: 1 in, 7 out]
          }
          event "Servo_Count_R": Value Change {
            w2226 = u8 0 items=["数据帧", "遥控帧"]
            w2225 = u8 0 items=["标准帧", "扩展帧"]
            # "地址"
            n1042 = event-data() -> ()  [unwired: 2 out]
            n1043 = property on="电机ID" class="CmbBox"() -> ("Value"=w2235:string)  [unwired: 2 in, 2 out]
            n1044 = Scan From String(format string="%x" ("格式字符串"), input string=w2235, default 1=u8 0) -> (output 1=w2238:u8)  [unwired: 2 in, 3 out]
            n1045 = call "Demo_MakeData.vi"("DataString"="73") -> ("Data"=w2222:u8[], "DataLen"=w2230:u8)  [unwired: 9 out]
            n1046 = Add(x=u32 48, y=w2238) -> (x+y=w2223:u32)
            n1047 = Bundle By Name(cluster=T6 {"ID"=0, "TimeStamp"=0, "TimeFlag"=0, "SendType"=0, "RemoteFlag"=0, "ExternFlag"=0, "DataLen"=0, "Data"=[], "Reserved"=[]} ("Send"), "ID"=w2223, "RemoteFlag"=w2226, "ExternFlag"=w2225, "DataLen"=w2230, "Data"=w2222) -> (w2227:T6)
            n1048 = Build Array(w2227) -> (w2228:T6[])
            n1049 = Unbundle By Name(w2220) -> ("DevType"=w2232:T5, "DevIndex"=w2231:u32, "CanIndex"=w2229:T4)
            n1050 = call "VCI_Transmit.vi"("Buffer"=w2228, "CANIndex"=w2229, "DevIndex"=w2231, "DevType"=w2232) -> ()  [unwired: 1 in, 7 out]
          }
          event "PosLimitEn_W": Value Change {
            w2257 = u8 0 items=["数据帧", "遥控帧"]
            w2258 = u8 0 items=["标准帧", "扩展帧"]
            # "索引地址"
            n1051 = event-data() -> ()  [unwired: 2 out]
            n1052 = property on="电机ID" class="CmbBox"() -> ("Value"=w2249:string)  [unwired: 2 in, 2 out]
            n1053 = Scan From String(format string="%x" ("格式字符串"), input string=w2249, default 1=u8 0) -> (output 1=w2246:u8)  [unwired: 2 in, 3 out]
            n1054 = Add(x=u32 16, y=w2246) -> (x+y=w2244:u32)
            n1055 = Build Array(u8 116, "限位En") -> (w2243:u8[])
            n1056 = Bundle By Name(cluster=T6 {"ID"=0, "TimeStamp"=0, "TimeFlag"=0, "SendType"=0, "RemoteFlag"=0, "ExternFlag"=0, "DataLen"=0, "Data"=[], "Reserved"=[]} ("Send"), "ID"=w2244, "RemoteFlag"=w2257, "ExternFlag"=w2258, "DataLen"=u8 2, "Data"=w2243) -> (w2256:T6)
            n1057 = Build Array(w2256) -> (w2255:T6[])
            n1058 = Unbundle By Name(w2245) -> ("DevType"=w2252:T5, "DevIndex"=w2253:u32, "CanIndex"=w2254:T4)
            n1059 = call "VCI_Transmit.vi"("Buffer"=w2255, "CANIndex"=w2254, "DevIndex"=w2253, "DevType"=w2252) -> ()  [unwired: 1 in, 7 out]
          }
          event "PosLimitEn_R": Value Change {
            w2269 = u8 0 items=["数据帧", "遥控帧"]
            w2268 = u8 0 items=["标准帧", "扩展帧"]
            # "地址"
            n1060 = event-data() -> ()  [unwired: 2 out]
            n1061 = property on="电机ID" class="CmbBox"() -> ("Value"=w2278:string)  [unwired: 2 in, 2 out]
            n1062 = Scan From String(format string="%x" ("格式字符串"), input string=w2278, default 1=u8 0) -> (output 1=w2281:u8)  [unwired: 2 in, 3 out]
            n1063 = call "Demo_MakeData.vi"("DataString"="74") -> ("Data"=w2264:u8[], "DataLen"=w2273:u8)  [unwired: 9 out]
            n1064 = Add(x=u32 48, y=w2281) -> (x+y=w2265:u32)
            n1065 = Bundle By Name(cluster=T6 {"ID"=0, "TimeStamp"=0, "TimeFlag"=0, "SendType"=0, "RemoteFlag"=0, "ExternFlag"=0, "DataLen"=0, "Data"=[], "Reserved"=[]} ("Send"), "ID"=w2265, "RemoteFlag"=w2269, "ExternFlag"=w2268, "DataLen"=w2273, "Data"=w2264) -> (w2270:T6)
            n1066 = Build Array(w2270) -> (w2271:T6[])
            n1067 = Unbundle By Name(w2266) -> ("DevType"=w2275:T5, "DevIndex"=w2274:u32, "CanIndex"=w2272:T4)
            n1068 = call "VCI_Transmit.vi"("Buffer"=w2271, "CANIndex"=w2272, "DevIndex"=w2274, "DevType"=w2275) -> ()  [unwired: 1 in, 7 out]
          }
          event "ZeroEn_W": Value Change {
            w2300 = u8 0 items=["数据帧", "遥控帧"]
            w2301 = u8 0 items=["标准帧", "扩展帧"]
            # "索引地址"
            n1069 = event-data() -> ()  [unwired: 2 out]
            n1070 = property on="电机ID" class="CmbBox"() -> ("Value"=w2292:string)  [unwired: 2 in, 2 out]
            n1071 = Scan From String(format string="%x" ("格式字符串"), input string=w2292, default 1=u8 0) -> (output 1=w2289:u8)  [unwired: 2 in, 3 out]
            n1072 = Add(x=u32 16, y=w2289) -> (x+y=w2287:u32)
            n1073 = Build Array(u8 118, "零位En") -> (w2286:u8[])
            n1074 = Bundle By Name(cluster=T6 {"ID"=0, "TimeStamp"=0, "TimeFlag"=0, "SendType"=0, "RemoteFlag"=0, "ExternFlag"=0, "DataLen"=0, "Data"=[], "Reserved"=[]} ("Send"), "ID"=w2287, "RemoteFlag"=w2300, "ExternFlag"=w2301, "DataLen"=u8 2, "Data"=w2286) -> (w2299:T6)
            n1075 = Build Array(w2299) -> (w2298:T6[])
            n1076 = Unbundle By Name(w2288) -> ("DevType"=w2295:T5, "DevIndex"=w2296:u32, "CanIndex"=w2297:T4)
            n1077 = call "VCI_Transmit.vi"("Buffer"=w2298, "CANIndex"=w2297, "DevIndex"=w2296, "DevType"=w2295) -> ()  [unwired: 1 in, 7 out]
          }
          event "ZeroEn_R": Value Change {
            w2322 = u8 0 items=["数据帧", "遥控帧"]
            w2323 = u8 0 items=["标准帧", "扩展帧"]
            # "地址"
            n1078 = event-data() -> ()  [unwired: 2 out]
            n1079 = property on="电机ID" class="CmbBox"() -> ("Value"=w2313:string)  [unwired: 2 in, 2 out]
            n1080 = Scan From String(format string="%x" ("格式字符串"), input string=w2313, default 1=u8 0) -> (output 1=w2310:u8)  [unwired: 2 in, 3 out]
            n1081 = call "Demo_MakeData.vi"("DataString"="76 ") -> ("Data"=w2306:u8[], "DataLen"=w2318:u8)  [unwired: 9 out]
            n1082 = Add(x=u32 48, y=w2310) -> (x+y=w2307:u32)
            n1083 = Bundle By Name(cluster=T6 {"ID"=0, "TimeStamp"=0, "TimeFlag"=0, "SendType"=0, "RemoteFlag"=0, "ExternFlag"=0, "DataLen"=0, "Data"=[], "Reserved"=[]} ("Send"), "ID"=w2307, "RemoteFlag"=w2322, "ExternFlag"=w2323, "DataLen"=w2318, "Data"=w2306) -> (w2321:T6)
            n1084 = Build Array(w2321) -> (w2320:T6[])
            n1085 = Unbundle By Name(w2309) -> ("DevType"=w2316:T5, "DevIndex"=w2317:u32, "CanIndex"=w2319:T4)
            n1086 = call "VCI_Transmit.vi"("Buffer"=w2320, "CANIndex"=w2319, "DevIndex"=w2317, "DevType"=w2316) -> ()  [unwired: 1 in, 7 out]
          }
          event "Zero_R": Value Change {
            w2333 = u8 0 items=["数据帧", "遥控帧"]
            w2332 = u8 0 items=["标准帧", "扩展帧"]
            # "地址"
            n1087 = event-data() -> ()  [unwired: 2 out]
            n1088 = property on="电机ID" class="CmbBox"() -> ("Value"=w2342:string)  [unwired: 2 in, 2 out]
            n1089 = Scan From String(format string="%x" ("格式字符串"), input string=w2342, default 1=u8 0) -> (output 1=w2345:u8)  [unwired: 2 in, 3 out]
            n1090 = call "Demo_MakeData.vi"("DataString"="75 ") -> ("Data"=w2328:u8[], "DataLen"=w2337:u8)  [unwired: 9 out]
            n1091 = Add(x=u32 48, y=w2345) -> (x+y=w2329:u32)
            n1092 = Bundle By Name(cluster=T6 {"ID"=0, "TimeStamp"=0, "TimeFlag"=0, "SendType"=0, "RemoteFlag"=0, "ExternFlag"=0, "DataLen"=0, "Data"=[], "Reserved"=[]} ("Send"), "ID"=w2329, "RemoteFlag"=w2333, "ExternFlag"=w2332, "DataLen"=w2337, "Data"=w2328) -> (w2334:T6)
            n1093 = Build Array(w2334) -> (w2335:T6[])
            n1094 = Unbundle By Name(w2330) -> ("DevType"=w2339:T5, "DevIndex"=w2338:u32, "CanIndex"=w2336:T4)
            n1095 = call "VCI_Transmit.vi"("Buffer"=w2335, "CANIndex"=w2336, "DevIndex"=w2338, "DevType"=w2339) -> ()  [unwired: 1 in, 7 out]
          }
        }
        "数组" <- w151
        "CAN ID" <- w150
      }
      frame "Exit" {
        n1096 = Release Queue(queue=w2357) -> ()  [unwired: 1 in, 4 out]
        n1097 = Unregister For Events(event registration refnum=w2356) -> (error out=w2355:errorcluster)  [unwired: 1 in]
        n1098 = Destroy User Event(user event=w2354, error in=w2355) -> ()  [unwired: 1 out]
        n1099 = Unbundle By Name(w2353) -> ("Open"=w2352:bool)
        n1100 = case shown="真" w2352 {
          tunnel: w2351 -> [_ w2361]
          frame False {
          }
          frame True {
            n1101 = Unbundle By Name(w2361) -> ("DevType"=w2360:T5, "DevIndex"=w2359:u32)
            n1102 = call "VCI_CloseDevice.vi"("DevIndex"=w2359, "DevType"=w2360) -> ()  [unwired: 1 in, 9 out]
          }
        }
        n1103 = local write "RcvEnable"(FALSE ("RcvEnable")) -> ()
      }
    }
  }
  n1104 = while "数据更新线程" {
    tunnel: w9 -> [w2367]
    shift-right: [w2362] -> _
    shift-left: u32 0 ("RecvCnt") -> [w2363]
    stop <- w2366 stop-if-true
    n1105 = Dequeue Element(queue=w2367) -> (element=w2365:T7, timed out?=w2364:bool, error out=w2366:errorcluster)  [unwired: 2 in, 1 out]
    n1106 = case shown="假" w2364 {
      tunnel: w2365 -> [w2377 _]
      tunnel: w2363 -> [w2371 w2943]
      tunnel: [w2370 w2943] -> w2362
      frame False {
        n1107 = Array To Cluster(array=w2377) -> (cluster=w2379:T12)
        n1108 = Unbundle By Name(w2379) -> ("[0]"=w2378:T13)
        n1109 = Increment(x=w2371) -> (x+1=w2370:u32)
        "sCnt" <- w2370
        n1110 = Unbundle By Name(w2378) -> ("VCI_CAN_OBJ"=w2376:T6)  [unwired: 3 out]
        n1111 = Unbundle By Name(w2376) -> ("ID"=w2374:u32, "Data"=w2375:u8[])  [unwired: 7 out]
        "CAN STD_ID" <- w2374
        n1112 = And(x=w2374, y=u32 15) -> (x .and. y?=→"电机ID_R":u32)
        n1113 = And(x=w2374, y=u32 240) -> (x .and. y?=w2369:u32)
        n1114 = case shown="40" w2369 {
          tunnel: w2375 -> [_ w2385]
          frame 0, Default {
          }
          frame 64 {
            n1115 = local read "存储路径"() -> (w2381:path)
            n1116 = local read "保存_S"() -> (w2382:bool)
            n1117 = Index Array(array=w2385, index=0) -> (element=w2384:u8)
            n1118 = case shown="6F" w2384 {
              tunnel: w2385 -> [_ w2410 w2419 w2432 w2443 w2450 w2469 w2489 w2513 w2530 w2550 w2563 w2588 w2607 w2624 w2628 w2635 w2643 w2653 w2659 w2672 w2675 w2685 w2695 w2705 w2715 w2725 w2735 w2745 w2755 w2763 w2772 w2775 w2781 w2789 w2795 w2801 w2807 w2813 w2819 w2825 w2831 w2834 w2837 w2840 w2850 w2860 w2868 w2874 w2882 w2887 w2895 w2899 w2902 w2912 w2915 w2923 w2929 w2935 w2938]
              tunnel: [_ _ _ _ _ _ w2458 w2479 w2502 w2528 w2545 w2562 w2577 w2601 _ _ _ _ _ _ _ _ _ _ _ _ _ _ _ _ _ _ _ _ _ _ _ _ _ _ _ _ _ _ _ _ _ _ _ _ _ _ _ _ _ _ _ _ _ _] -> w2380
              frame 0, Default {
              }
              frame 1 {
                n1119 = Array To Cluster(array=w2410) -> (cluster=w2411:T14)
                n1120 = Unbundle By Name(w2411) -> ("Data[1]"=w2413:u8, "Data[2]"=w2414:u8)  [unwired: 1 out]
                n1121 = Join Numbers(hi=w2413, lo=w2414) -> ((hi.lo)=w2412:u16)
                n1122 = To Unsigned Word Integer(number=w2412) -> (unsigned 16bit integer=→"看门狗周期_回":u16)
              }
              frame 32 {
                n1123 = Array To Cluster(array=w2419) -> (cluster=w2420:T14)
                n1124 = Unbundle By Name(w2420) -> ("Data[1]"=w2418:u8)  [unwired: 1 out]
                n1125 = To Unsigned Byte Integer(number=w2418) -> (unsigned 8bit integer=w2415:u8)
                n1126 = Number To Hexadecimal String(1:2, 2:w2415) -> (0:w2416:string)
                n1127 = property on="模式_回" class="CmbBox"("Value"=w2416) -> ()  [unwired: 2 in, 2 out]
              }
              frame 33 {
                n1128 = Array To Cluster(array=w2432) -> (cluster=w2434:T14)
                n1129 = Unbundle By Name(w2434) -> ("Data[1]"=w2433:u8)  [unwired: 1 out]
                n1130 = To Unsigned Byte Integer(number=w2433) -> (unsigned 8bit integer=w2431:u8)
                n1131 = Number To Boolean Array(number=w2431) -> (Boolean array=w2430:bool[])
                n1132 = Array To Cluster(array=w2430) -> (cluster=w2429:T15)
                n1133 = Unbundle(w2429) -> ("Boolean array[0]"=→"warn0":bool, "Boolean array[1]"=→"warn1":bool, "Boolean array[2]"=→"高温":bool, "Boolean array[3]"=→"warn3":bool, "Boolean array[4]"=→"warn4":bool, "Boolean array[5]"=→"warn5":bool, "Boolean array[6]"=→"warn6":bool, "Boolean array[7]"=→"warn7":bool)
              }
              frame 34 {
                n1134 = Array To Cluster(array=w2443) -> (cluster=w2448:T14)
                n1135 = Unbundle By Name(w2448) -> ("Data[1]"=w2447:u8)  [unwired: 1 out]
                n1136 = To Unsigned Byte Integer(number=w2447) -> (unsigned 8bit integer=w2446:u8)
                n1137 = Number To Boolean Array(number=w2446) -> (Boolean array=w2445:bool[])
                n1138 = Array To Cluster(array=w2445) -> (cluster=w2444:T15)
                n1139 = Unbundle(w2444) -> ("Boolean array[0]"=→"低压":bool, "Boolean array[1]"=→"高压":bool, "Boolean array[2]"=→"高温":bool, "Boolean array[3]"=→"ERRO3":bool, "Boolean array[4]"=→"ERRO4":bool, "Boolean array[5]"=→"ERRO5":bool, "Boolean array[6]"=→"ERRO6":bool, "Boolean array[7]"=→"ERRO7":bool)
              }
              frame 35 {
                n1140 = Array To Cluster(array=w2450) -> (cluster=w2451:T14)
                n1141 = Unbundle By Name(w2451) -> ("Data[1]"=w2453:u8, "Data[2]"=w2454:u8)  [unwired: 1 out]
                n1142 = Join Numbers(hi=w2453, lo=w2454) -> ((hi.lo)=w2452:u16)
                n1143 = To Unsigned Word Integer(number=w2452) -> (unsigned 16bit integer=→"监测周期_回":u16)
              }
              frame 49 {
                w2471 = 8
                n1144 = Array To Cluster(array=w2469) -> (cluster=w2475:T14)
                n1145 = Unbundle By Name(w2475) -> ("Data[1]"=w2463:u8, "Data[2]"=w2464:u8, "Data[3]"=w2465:u8, "Data[4]"=w2466:u8, "Data[5]"=w2462:u8, "Data[6]"=w2461:u8)  [unwired: 1 out]
                n1146 = Join Numbers(hi=w2462, lo=w2461) -> ((hi.lo)=w2460:u16)
                n1147 = To Word Integer(number=w2463) -> (16bit integer=w2478:i16)
                n1148 = To Unsigned Word Integer(number=w2465) -> (unsigned 16bit integer=w2474:u16)
                n1149 = To Word Integer(number=w2460) -> (16bit integer=w2459:i16)
                n1150 = Rotate(1:w2478, 2:w2471) -> (0:w2477:i16)
                n1151 = Rotate(1:w2474, 2:w2471) -> (0:w2473:u16)
                n1152 = Add(x=w2477, y=w2464) -> (x+y=w2476:i16)
                n1153 = Add(x=w2473, y=w2466) -> (x+y=w2472:u16)
                n1154 = Divide(x=w2476, y=128.0) -> (x/y=w2468:dbl)
                "机械角度" <- w2468
                n1155 = Multiply(x=w2472, y=0.00549) -> (x*y=w2467:dbl)
                "电气角度" <- w2467
                n1156 = Divide(x=w2459, y=1.0) -> (x/y=w2457:dbl)
                "转速" <- w2457
                "转速" <- w2457
                n1157 = Build Array(w2468, w2467, w2457) -> (w2458:dbl[])
              }
              frame 50 {
                w2490 = i16 1024
                w2491 = 8
                n1158 = Array To Cluster(array=w2489) -> (cluster=w2498:T14)
                n1159 = Unbundle By Name(w2498) -> ("Data[1]"=w2488:u8, "Data[2]"=w2487:u8, "Data[3]"=w2486:u8, "Data[4]"=w2485:u8, "Data[5]"=w2484:u8, "Data[6]"=w2483:u8)  [unwired: 1 out]
                n1160 = To Word Integer(number=w2488) -> (16bit integer=w2501:i16)
                n1161 = To Word Integer(number=w2484) -> (16bit integer=w2494:i16)
                n1162 = To Word Integer(number=w2486) -> (16bit integer=w2497:i16)
                n1163 = Rotate(1:w2501, 2:w2491) -> (0:w2500:i16)
                n1164 = Rotate(1:w2494, 2:w2491) -> (0:w2493:i16)
                n1165 = Rotate(1:w2497, 2:w2491) -> (0:w2496:i16)
                n1166 = Add(x=w2500, y=w2487) -> (x+y=w2499:i16)
                n1167 = Add(x=w2493, y=w2483) -> (x+y=w2492:i16)
                n1168 = Add(x=w2496, y=w2485) -> (x+y=w2495:i16)
                n1169 = Divide(x=w2499, y=w2490) -> (x/y=w2482:dbl)
                "A电流" <- w2482
                "波形图表1" <- w2482
                n1170 = Divide(x=w2492, y=w2490) -> (x/y=w2480:dbl)
                "C电流" <- w2480
                "波形图表3" <- w2480
                n1171 = Divide(x=w2495, y=w2490) -> (x/y=w2481:dbl)
                "B电流" <- w2481
                "波形图表2" <- w2481
                n1172 = Build Array(w2482, w2481, w2480) -> (w2479:dbl[])
              }
              frame 51 {
                w2515 = i16 256
                w2514 = 8
                n1173 = Array To Cluster(array=w2513) -> (cluster=w2522:T14)
                n1174 = Unbundle By Name(w2522) -> ("Data[1]"=w2512:u8, "Data[2]"=w2511:u8, "Data[3]"=w2510:u8, "Data[4]"=w2509:u8, "Data[5]"=w2508:u8, "Data[6]"=w2507:u8)  [unwired: 1 out]
                n1175 = To Unsigned Word Integer(number=w2512) -> (unsigned 16bit integer=w2525:u16)
                n1176 = To Word Integer(number=w2510) -> (16bit integer=w2521:i16)
                n1177 = To Word Integer(number=w2508) -> (16bit integer=w2518:i16)
                n1178 = Rotate(1:w2525, 2:w2514) -> (0:w2524:u16)
                n1179 = Rotate(1:w2521, 2:w2514) -> (0:w2520:i16)
                n1180 = Rotate(1:w2518, 2:w2514) -> (0:w2517:i16)
                n1181 = Add(x=w2524, y=w2511) -> (x+y=w2523:u16)
                n1182 = Add(x=w2520, y=w2509) -> (x+y=w2519:i16)
                n1183 = Add(x=w2517, y=w2507) -> (x+y=w2516:i16)
                n1184 = Divide(x=w2523, y=i16 1024) -> (x/y=w2505:dbl)
                "供电电压" <- w2505
                n1185 = Divide(x=w2519, y=w2515) -> (x/y=w2504:dbl)
                "Ialfa" <- w2504
                n1186 = Divide(x=w2516, y=w2515) -> (x/y=w2503:dbl)
                "Ibeta" <- w2503
                n1187 = Build Array(w2505, w2504, w2503) -> (w2502:dbl[])
              }
              frame 52 {
                w2529 = i16 256
                w2535 = 8
                n1188 = Array To Cluster(array=w2530) -> (cluster=w2539:T14)
                n1189 = Unbundle By Name(w2539) -> ("Data[1]"=w2534:u8, "Data[2]"=w2533:u8, "Data[3]"=w2532:u8, "Data[4]"=w2531:u8)  [unwired: 1 out]
                n1190 = To Word Integer(number=w2534) -> (16bit integer=w2542:i16)
                n1191 = To Word Integer(number=w2532) -> (16bit integer=w2538:i16)
                n1192 = Rotate(1:w2542, 2:w2535) -> (0:w2541:i16)
                n1193 = Rotate(1:w2538, 2:w2535) -> (0:w2537:i16)
                n1194 = Add(x=w2541, y=w2533) -> (x+y=w2540:i16)
                n1195 = Add(x=w2537, y=w2531) -> (x+y=w2536:i16)
                n1196 = Divide(x=w2540, y=w2529) -> (x/y=w2527:dbl)
                "Iqnow" <- w2527
                n1197 = Divide(x=w2536, y=w2529) -> (x/y=w2526:dbl)
                "Idnow" <- w2526
                n1198 = Build Array(w2527, w2526) -> (w2528:dbl[])
              }
              frame 53 {
                w2552 = i16 1024
                w2551 = 8
                n1199 = Array To Cluster(array=w2550) -> (cluster=w2556:T14)
                n1200 = Unbundle By Name(w2556) -> ("Data[1]"=w2549:u8, "Data[2]"=w2548:u8, "Data[3]"=w2547:u8, "Data[4]"=w2546:u8)  [unwired: 1 out]
                n1201 = To Word Integer(number=w2549) -> (16bit integer=w2559:i16)
                n1202 = To Word Integer(number=w2547) -> (16bit integer=w2555:i16)
                n1203 = Rotate(1:w2559, 2:w2551) -> (0:w2558:i16)
                n1204 = Rotate(1:w2555, 2:w2551) -> (0:w2554:i16)
                n1205 = Add(x=w2558, y=w2548) -> (x+y=w2557:i16)
                n1206 = Add(x=w2554, y=w2546) -> (x+y=w2553:i16)
                n1207 = Divide(x=w2557, y=w2552) -> (x/y=w2544:dbl)
                "Uq" <- w2544
                n1208 = Divide(x=w2553, y=w2552) -> (x/y=w2543:dbl)
                "Ud" <- w2543
                n1209 = Build Array(w2544, w2543) -> (w2545:dbl[])
              }
              frame 54 {
                w2569 = i16 1024
                w2568 = 8
                n1210 = Array To Cluster(array=w2563) -> (cluster=w2573:T14)
                n1211 = Unbundle By Name(w2573) -> ("Data[1]"=w2567:u8, "Data[2]"=w2566:u8, "Data[3]"=w2565:u8, "Data[4]"=w2564:u8)  [unwired: 1 out]
                n1212 = To Word Integer(number=w2567) -> (16bit integer=w2576:i16)
                n1213 = To Word Integer(number=w2565) -> (16bit integer=w2572:i16)
                n1214 = Rotate(1:w2576, 2:w2568) -> (0:w2575:i16)
                n1215 = Rotate(1:w2572, 2:w2568) -> (0:w2571:i16)
                n1216 = Add(x=w2575, y=w2566) -> (x+y=w2574:i16)
                n1217 = Add(x=w2571, y=w2564) -> (x+y=w2570:i16)
                n1218 = Divide(x=w2574, y=w2569) -> (x/y=w2561:dbl)
                "Ualfa" <- w2561
                n1219 = Divide(x=w2570, y=w2569) -> (x/y=w2560:dbl)
                "Ubate" <- w2560
                n1220 = Build Array(w2561, w2560) -> (w2562:dbl[])
              }
              frame 55 {
                w2590 = u16 0
                w2589 = 8
                n1221 = Array To Cluster(array=w2588) -> (cluster=w2597:T14)
                n1222 = Unbundle By Name(w2597) -> ("Data[1]"=w2582:u8, "Data[2]"=w2583:u8, "Data[3]"=w2584:u8, "Data[4]"=w2585:u8, "Data[5]"=w2586:u8, "Data[6]"=w2587:u8, "Data[7]"=w2578:u8)  [unwired: 1 out]
                "sector" <- w2578
                n1223 = To Word Integer(number=w2582) -> (16bit integer=w2600:i16)
                n1224 = To Word Integer(number=w2584) -> (16bit integer=w2596:i16)
                n1225 = To Word Integer(number=w2586) -> (16bit integer=w2593:i16)
                n1226 = Rotate(1:w2600, 2:w2589) -> (0:w2599:i16)
                n1227 = Rotate(1:w2596, 2:w2589) -> (0:w2595:i16)
                n1228 = Rotate(1:w2593, 2:w2589) -> (0:w2592:i16)
                n1229 = Add(x=w2599, y=w2583) -> (x+y=w2598:i16)
                n1230 = Add(x=w2595, y=w2585) -> (x+y=w2594:i16)
                n1231 = Add(x=w2592, y=w2587) -> (x+y=w2591:i16)
                n1232 = Subtract ("减")(x=w2598, y=w2590) -> (x-y=w2581:u16)
                "PWM1" <- w2581
                n1233 = Subtract ("减")(x=w2594, y=w2590) -> (x-y=w2580:u16)
                "PWM2" <- w2580
                n1234 = Subtract ("减")(x=w2591, y=w2590) -> (x-y=w2579:u16)
                "PWM3" <- w2579
                n1235 = Build Array(w2581, w2580, w2579, w2578) -> (w2577:u16[])
              }
              frame 56 {
                n1236 = Array Subset(array=w2607, index=1, length=4) -> (w2604:u8[])
                n1237 = Type Cast(type=2097152, x=w2604) -> (*(type *) &x=w2602:i32)
                "Sin" <- w2602
                "Cosin" <- w2602
                n1238 = Build Array(w2602, w2602) -> (w2601:i32[])
              }
              frame 57 {
                n1239 = Array To Cluster(array=w2624) -> (cluster=w2625:cluster{"Data[0]":u8, "Data[1]":u8})
                n1240 = Unbundle By Name(w2625) -> ("Data[1]"=w2616:u8)  [unwired: 1 out]
                n1241 = And(x=w2616, y=u8 56) -> (x .and. y?=w2619:u8)
                n1242 = And(x=w2616, y=u8 192) -> (x .and. y?=w2622:u8)
                n1243 = And(x=w2616, y=u8 7) -> (x .and. y?=w2613:u8)
                n1244 = Logical Shift(y=i16 -3, x=w2619) -> (x << y=w2615:u8)
                n1245 = Logical Shift(y=i16 -6, x=w2622) -> (x << y=w2611:u8)
                n1246 = Divide(x=w2615, y=u8 10) -> (x/y=w2610:dbl)
                n1247 = Divide(x=w2613, y=u8 100) -> (x/y=w2609:dbl)
                n1248 = Compound Arithmetic op=ADD(w2611, w2610, w2609) -> (→"版本号":dbl)
              }
              frame 58 {
                n1249 = Array To Cluster(array=w2628) -> (cluster=w2633:T14)
                n1250 = Unbundle By Name(w2633) -> ("Data[1]"=w2631:u8, "Data[2]"=w2630:u8)  [unwired: 1 out]
                n1251 = Join Numbers(hi=w2631, lo=w2630) -> ((hi.lo)=w2632:u16)
                n1252 = To Unsigned Word Integer(number=w2632) -> (unsigned 16bit integer=w2629:u16)
                n1253 = Multiply(x=w2629, y=0.0054931640625) -> (x*y=w2627:dbl)
                n1254 = property on="机械角度" class="DigNum (严格)"("Value"=w2627) -> ()  [unwired: 2 in, 2 out]
              }
              frame 59 {
                n1255 = Array To Cluster(array=w2635) -> (cluster=w2641:T14)
                n1256 = Unbundle By Name(w2641) -> ("Data[1]"=w2639:u8, "Data[2]"=w2638:u8)  [unwired: 1 out]
                n1257 = Join Numbers(hi=w2639, lo=w2638) -> ((hi.lo)=w2640:u16)
                n1258 = To Word Integer(number=w2640) -> (16bit integer=w2637:i16)
                n1259 = Divide(x=w2637, y=i16 1) -> (x/y=w2634:dbl)
                n1260 = property on="转速" class="DigNum (严格)"("Value"=w2634) -> ()  [unwired: 2 in, 2 out]
              }
              frame 60 {
                n1261 = Array To Cluster(array=w2643) -> (cluster=w2649:T14)
                n1262 = Unbundle By Name(w2649) -> ("Data[1]"=w2647:u8, "Data[2]"=w2646:u8)  [unwired: 1 out]
                n1263 = Join Numbers(hi=w2647, lo=w2646) -> ((hi.lo)=w2648:u16)
                n1264 = To Word Integer(number=w2648) -> (16bit integer=w2645:i16)
                n1265 = Divide(x=w2645, y=i16 256) -> (x/y=w2642:dbl)
                n1266 = property on="Iqnow" class="DigNum (严格)"("Value"=w2642) -> ()  [unwired: 2 in, 2 out]
              }
              frame 61 {
                n1267 = Array To Cluster(array=w2653) -> (cluster=w2657:T14)
                n1268 = Unbundle By Name(w2657) -> ("Data[1]"=w2655:u8, "Data[2]"=w2654:u8)  [unwired: 1 out]
                n1269 = Join Numbers(hi=w2655, lo=w2654) -> ((hi.lo)=w2656:u16)
                n1270 = To Word Integer(number=w2656) -> (16bit integer=w2652:i16)
                n1271 = Divide(x=w2652, y=i16 4) -> (x/y=→"温度":dbl)
              }
              frame 64 {
                n1272 = Array To Cluster(array=w2659) -> (cluster=w2664:T14)
                n1273 = Unbundle By Name(w2664) -> ("Data[1]"=w2660:u8, "Data[2]"=w2661:u8)  [unwired: 1 out]
                n1274 = To Unsigned Word Integer(number=w2660) -> (unsigned 16bit integer=w2667:u16)
                n1275 = Rotate(1:w2667, 2:8) -> (0:w2666:u16)
                n1276 = Add ("加")(x=w2666, y=w2661) -> (x+y=w2665:u16)
                n1277 = Divide(x=w2665, y=u16 256) -> (x/y=→"设定位置_回":dbl)
              }
              frame 65 {
                n1278 = Array To Cluster(array=w2672) -> (cluster=w2673:T14)
                n1279 = Unbundle By Name(w2673) -> ("Data[1]"=w2670:u8, "Data[2]"=w2669:u8)  [unwired: 1 out]
                n1280 = Join Numbers(hi=w2670, lo=w2669) -> ((hi.lo)=w2671:u16)
                n1281 = To Word Integer(number=w2671) -> (16bit integer=→"设定速度_回":i16)
              }
              frame 67 {
                n1282 = Array To Cluster(array=w2675) -> (cluster=w2679:T14)
                n1283 = Unbundle By Name(w2679) -> ("Data[1]"=w2683:u8, "Data[2]"=w2682:u8)  [unwired: 1 out]
                n1284 = To Word Integer(number=w2683) -> (16bit integer=w2676:i16)
                n1285 = Rotate(1:w2676, 2:8) -> (0:w2677:i16)
                n1286 = Add ("加")(x=w2677, y=w2682) -> (x+y=w2678:i16)
                n1287 = Divide(x=w2678, y=u16 256) -> (x/y=→"设定力矩_回":dbl)
              }
              frame 66 {
                n1288 = Array To Cluster(array=w2685) -> (cluster=w2690:T14)
                n1289 = Unbundle By Name(w2690) -> ("Data[1]"=w2686:u8, "Data[2]"=w2687:u8)  [unwired: 1 out]
                n1290 = To Word Integer(number=w2686) -> (16bit integer=w2693:i16)
                n1291 = Rotate(1:w2693, 2:8) -> (0:w2692:i16)
                n1292 = Add ("加")(x=w2692, y=w2687) -> (x+y=w2691:i16)
                n1293 = Divide(x=w2691, y=u16 256) -> (x/y=→"设定电流_回":dbl)
              }
              frame 81 {
                n1294 = Array To Cluster(array=w2695) -> (cluster=w2700:T14)
                n1295 = Unbundle By Name(w2700) -> ("Data[1]"=w2696:u8, "Data[2]"=w2697:u8)  [unwired: 1 out]
                n1296 = To Unsigned Word Integer(number=w2696) -> (unsigned 16bit integer=w2703:u16)
                n1297 = Rotate(1:w2703, 2:8) -> (0:w2702:u16)
                n1298 = Add ("加")(x=w2702, y=w2697) -> (x+y=w2701:u16)
                n1299 = Divide(x=w2701, y=u16 256) -> (x/y=→"电流环KP_回":dbl)
              }
              frame 82 {
                n1300 = Array To Cluster(array=w2705) -> (cluster=w2710:T14)
                n1301 = Unbundle By Name(w2710) -> ("Data[1]"=w2706:u8, "Data[2]"=w2707:u8)  [unwired: 1 out]
                n1302 = To Unsigned Word Integer(number=w2706) -> (unsigned 16bit integer=w2713:u16)
                n1303 = Rotate(1:w2713, 2:8) -> (0:w2712:u16)
                n1304 = Add ("加")(x=w2712, y=w2707) -> (x+y=w2711:u16)
                n1305 = Divide(x=w2711, y=u16 256) -> (x/y=→"电流环KI_回":dbl)
              }
              frame 83 {
                n1306 = Array To Cluster(array=w2715) -> (cluster=w2720:T14)
                n1307 = Unbundle By Name(w2720) -> ("Data[1]"=w2716:u8, "Data[2]"=w2717:u8)  [unwired: 1 out]
                n1308 = To Unsigned Word Integer(number=w2716) -> (unsigned 16bit integer=w2723:u16)
                n1309 = Rotate(1:w2723, 2:8) -> (0:w2722:u16)
                n1310 = Add ("加")(x=w2722, y=w2717) -> (x+y=w2721:u16)
                n1311 = Divide(x=w2721, y=u16 256) -> (x/y=→"速度环KP_回":dbl)
              }
              frame 84 {
                n1312 = Array To Cluster(array=w2725) -> (cluster=w2730:T14)
                n1313 = Unbundle By Name(w2730) -> ("Data[1]"=w2726:u8, "Data[2]"=w2727:u8)  [unwired: 1 out]
                n1314 = To Unsigned Word Integer(number=w2726) -> (unsigned 16bit integer=w2733:u16)
                n1315 = Rotate(1:w2733, 2:8) -> (0:w2732:u16)
                n1316 = Add ("加")(x=w2732, y=w2727) -> (x+y=w2731:u16)
                n1317 = Divide(x=w2731, y=u16 256) -> (x/y=→"速度环KI_回":dbl)
              }
              frame 85 {
                n1318 = Array To Cluster(array=w2735) -> (cluster=w2740:T14)
                n1319 = Unbundle By Name(w2740) -> ("Data[1]"=w2736:u8, "Data[2]"=w2737:u8)  [unwired: 1 out]
                n1320 = To Unsigned Word Integer(number=w2736) -> (unsigned 16bit integer=w2743:u16)
                n1321 = Rotate(1:w2743, 2:8) -> (0:w2742:u16)
                n1322 = Add ("加")(x=w2742, y=w2737) -> (x+y=w2741:u16)
                n1323 = Divide(x=w2741, y=u16 8) -> (x/y=→"加速度_回":dbl)
              }
              frame 86 {
                n1324 = Array To Cluster(array=w2745) -> (cluster=w2750:T14)
                n1325 = Unbundle By Name(w2750) -> ("Data[1]"=w2746:u8, "Data[2]"=w2747:u8)  [unwired: 1 out]
                n1326 = To Unsigned Word Integer(number=w2746) -> (unsigned 16bit integer=w2753:u16)
                n1327 = Rotate(1:w2753, 2:8) -> (0:w2752:u16)
                n1328 = Add ("加")(x=w2752, y=w2747) -> (x+y=w2751:u16)
                n1329 = Divide(x=w2751, y=u16 8) -> (x/y=→"减速度_回":dbl)
              }
              frame 87 {
                n1330 = Array To Cluster(array=w2755) -> (cluster=w2761:T14)
                n1331 = Unbundle By Name(w2761) -> ("Data[1]"=w2759:u8, "Data[2]"=w2758:u8)  [unwired: 1 out]
                n1332 = Join Numbers(hi=w2759, lo=w2758) -> ((hi.lo)=w2760:u16)
                n1333 = To Unsigned Word Integer(number=w2760) -> (unsigned 16bit integer=w2757:u16)
                n1334 = Divide(x=w2757, y=u16 8) -> (x/y=→"电流限制_回":dbl)
              }
              frame 88 {
                n1335 = Array To Cluster(array=w2763) -> (cluster=w2767:T14)
                n1336 = Unbundle By Name(w2767) -> ("Data[1]"=w2765:u8, "Data[2]"=w2764:u8)  [unwired: 1 out]
                n1337 = Join Numbers(hi=w2765, lo=w2764) -> ((hi.lo)=w2766:u16)
                n1338 = To Unsigned Word Integer(number=w2766) -> (unsigned 16bit integer=→"速度限制_回":u16)
              }
              frame 90 {
                n1339 = Array To Cluster(array=w2772) -> (cluster=w2773:T14)
                n1340 = Unbundle By Name(w2773) -> ("Data[1]"=w2770:u8, "Data[2]"=w2769:u8)  [unwired: 1 out]
                n1341 = Join Numbers(hi=w2770, lo=w2769) -> ((hi.lo)=w2771:u16)
                n1342 = To Unsigned Word Integer(number=w2771) -> (unsigned 16bit integer=→"AI_K0_回":u16)
              }
              frame 91 {
                n1343 = Array To Cluster(array=w2775) -> (cluster=w2779:T14)
                n1344 = Unbundle By Name(w2779) -> ("Data[1]"=w2777:u8, "Data[2]"=w2776:u8)  [unwired: 1 out]
                n1345 = Join Numbers(hi=w2777, lo=w2776) -> ((hi.lo)=w2778:u16)
                n1346 = To Unsigned Word Integer(number=w2778) -> (unsigned 16bit integer=→"BI_K0_回":u16)
              }
              frame 92 {
                n1347 = Array To Cluster(array=w2781) -> (cluster=w2785:T14)
                n1348 = Unbundle By Name(w2785) -> ("Data[1]"=w2783:u8, "Data[2]"=w2782:u8)  [unwired: 1 out]
                n1349 = Join Numbers(hi=w2783, lo=w2782) -> ((hi.lo)=w2784:u16)
                n1350 = To Unsigned Word Integer(number=w2784) -> (unsigned 16bit integer=→"CI_K0_回":u16)
              }
              frame 93 {
                n1351 = Array To Cluster(array=w2789) -> (cluster=w2793:T14)
                n1352 = Unbundle By Name(w2793) -> ("Data[1]"=w2791:u8, "Data[2]"=w2790:u8)  [unwired: 1 out]
                n1353 = Join Numbers(hi=w2791, lo=w2790) -> ((hi.lo)=w2792:u16)
                n1354 = To Unsigned Word Integer(number=w2792) -> (unsigned 16bit integer=w2788:u16)
                n1355 = Divide(x=w2788, y=u16 8) -> (x/y=→"对准角_回":dbl)
              }
              frame 96 {
                n1356 = Array To Cluster(array=w2795) -> (cluster=w2799:T14)
                n1357 = Unbundle By Name(w2799) -> ("Data[1]"=w2798:u8, "Data[2]"=w2797:u8)  [unwired: 1 out]
                n1358 = Join Numbers(hi=w2798, lo=w2797) -> ((hi.lo)=w2796:u16)
                n1359 = To Unsigned Word Integer(number=w2796) -> (unsigned 16bit integer=→"W1":u16)
              }
              frame 98 {
                n1360 = Array To Cluster(array=w2801) -> (cluster=w2802:T14)
                n1361 = Unbundle By Name(w2802) -> ("Data[1]"=w2804:u8, "Data[2]"=w2805:u8)  [unwired: 1 out]
                n1362 = Join Numbers(hi=w2804, lo=w2805) -> ((hi.lo)=w2803:u16)
                n1363 = To Unsigned Word Integer(number=w2803) -> (unsigned 16bit integer=→"W3":u16)
              }
              frame 99 {
                n1364 = Array To Cluster(array=w2807) -> (cluster=w2808:T14)
                n1365 = Unbundle By Name(w2808) -> ("Data[1]"=w2810:u8, "Data[2]"=w2811:u8)  [unwired: 1 out]
                n1366 = Join Numbers(hi=w2810, lo=w2811) -> ((hi.lo)=w2809:u16)
                n1367 = To Unsigned Word Integer(number=w2809) -> (unsigned 16bit integer=→"W4":u16)
              }
              frame 100 {
                n1368 = Array To Cluster(array=w2813) -> (cluster=w2814:T14)
                n1369 = Unbundle By Name(w2814) -> ("Data[1]"=w2816:u8, "Data[2]"=w2817:u8)  [unwired: 1 out]
                n1370 = Join Numbers(hi=w2816, lo=w2817) -> ((hi.lo)=w2815:u16)
                n1371 = To Unsigned Word Integer(number=w2815) -> (unsigned 16bit integer=→"T1":u16)
              }
              frame 102 {
                n1372 = Array To Cluster(array=w2819) -> (cluster=w2820:T14)
                n1373 = Unbundle By Name(w2820) -> ("Data[1]"=w2822:u8, "Data[2]"=w2823:u8)  [unwired: 1 out]
                n1374 = Join Numbers(hi=w2822, lo=w2823) -> ((hi.lo)=w2821:u16)
                n1375 = To Unsigned Word Integer(number=w2821) -> (unsigned 16bit integer=→"T3":u16)
              }
              frame 103 {
                n1376 = Array To Cluster(array=w2825) -> (cluster=w2826:T14)
                n1377 = Unbundle By Name(w2826) -> ("Data[1]"=w2828:u8, "Data[2]"=w2829:u8)  [unwired: 1 out]
                n1378 = Join Numbers(hi=w2828, lo=w2829) -> ((hi.lo)=w2827:u16)
                n1379 = To Unsigned Word Integer(number=w2827) -> (unsigned 16bit integer=→"T4":u16)
              }
              frame 104 {
                n1380 = Array To Cluster(array=w2831) -> (cluster=w2832:T14)
                n1381 = Unbundle By Name(w2832) -> ("Data[1]"=→"电流使能":u8)  [unwired: 1 out]
              }
              frame 105 {
                n1382 = Array To Cluster(array=w2834) -> (cluster=w2835:T14)
                n1383 = Unbundle By Name(w2835) -> ("Data[1]"=→"功率使能":u8)  [unwired: 1 out]
              }
              frame 106 {
                n1384 = Array To Cluster(array=w2837) -> (cluster=w2838:T14)
                n1385 = Unbundle By Name(w2838) -> ("Data[1]"=→"方向":u8)  [unwired: 1 out]
              }
              frame 107 {
                n1386 = Array To Cluster(array=w2840) -> (cluster=w2844:T14)
                n1387 = Unbundle By Name(w2844) -> ("Data[1]"=w2848:u8, "Data[2]"=w2847:u8)  [unwired: 1 out]
                n1388 = To Unsigned Word Integer(number=w2848) -> (unsigned 16bit integer=w2841:u16)
                n1389 = Rotate(1:w2841, 2:8) -> (0:w2842:u16)
                n1390 = Add ("加")(x=w2842, y=w2847) -> (x+y=w2843:u16)
                n1391 = Divide(x=w2843, y=u16 256) -> (x/y=→"位置环KP_回":dbl)
              }
              frame 108 {
                n1392 = Array To Cluster(array=w2850) -> (cluster=w2855:T14)
                n1393 = Unbundle By Name(w2855) -> ("Data[1]"=w2851:u8, "Data[2]"=w2852:u8)  [unwired: 1 out]
                n1394 = To Unsigned Word Integer(number=w2851) -> (unsigned 16bit integer=w2858:u16)
                n1395 = Rotate(1:w2858, 2:8) -> (0:w2857:u16)
                n1396 = Add ("加")(x=w2857, y=w2852) -> (x+y=w2856:u16)
                n1397 = Divide(x=w2856, y=u16 256) -> (x/y=→"位置环KI_回":dbl)
              }
              frame 110 {
                n1398 = Array To Cluster(array=w2860) -> (cluster=w2861:T14)
                n1399 = Unbundle By Name(w2861) -> ("Data[1]"=w2863:u8, "Data[2]"=w2864:u8)  [unwired: 1 out]
                n1400 = Join Numbers(hi=w2863, lo=w2864) -> ((hi.lo)=w2862:u16)
                n1401 = To Word Integer(number=w2862) -> (16bit integer=w2865:i16)
                n1402 = Divide(x=w2865, y=u16 1) -> (x/y=→"上限位 _回":dbl)
              }
              frame 111 {
                n1403 = Array To Cluster(array=w2868) -> (cluster=w2872:T14)
                n1404 = Unbundle By Name(w2872) -> ("Data[1]"=w2870:u8, "Data[2]"=w2869:u8)  [unwired: 1 out]
                n1405 = Join Numbers(hi=w2870, lo=w2869) -> ((hi.lo)=w2871:u16)
                n1406 = To Word Integer(number=w2871) -> (16bit integer=→"下限位":i16)
              }
              frame 113 {
                n1407 = Array To Cluster(array=w2874) -> (cluster=w2880:T14)
                n1408 = Unbundle By Name(w2880) -> ("Data[1]"=w2878:u8, "Data[2]"=w2877:u8)  [unwired: 1 out]
                n1409 = Join Numbers(hi=w2878, lo=w2877) -> ((hi.lo)=w2879:u16)
                n1410 = To Unsigned Word Integer(number=w2879) -> (unsigned 16bit integer=w2876:u16)
                n1411 = Divide(x=w2876, y=u16 1) -> (x/y=→"Gear":dbl)
              }
              frame 115 {
                n1412 = Array To Cluster(array=w2882) -> (cluster=w2883:T14)
                n1413 = Unbundle By Name(w2883) -> ("Data[1]"=w2885:u8, "Data[2]"=w2886:u8)  [unwired: 1 out]
                n1414 = Join Numbers(hi=w2885, lo=w2886) -> ((hi.lo)=w2884:u16)
                n1415 = To Unsigned Word Integer(number=w2884) -> (unsigned 16bit integer=→"伺服频率R":u16)
              }
              frame 117 {
                n1416 = Array To Cluster(array=w2887) -> (cluster=w2894:T14)
                n1417 = Unbundle By Name(w2894) -> ("Data[1]"=w2892:u8, "Data[2]"=w2891:u8)  [unwired: 1 out]
                n1418 = Join Numbers(hi=w2892, lo=w2891) -> ((hi.lo)=w2893:u16)
                n1419 = To Unsigned Word Integer(number=w2893) -> (unsigned 16bit integer=w2890:u16)
                n1420 = Divide(x=w2890, y=u16 128) -> (x/y=→"零位角":dbl)
              }
              frame 118 {
                n1421 = Array To Cluster(array=w2895) -> (cluster=w2897:T14)
                n1422 = Unbundle By Name(w2897) -> ("Data[1]"=→"零位使能":u8)  [unwired: 1 out]
              }
              frame 116 {
                n1423 = Array To Cluster(array=w2899) -> (cluster=w2900:T14)
                n1424 = Unbundle By Name(w2900) -> ("Data[1]"=→"限位使能":u8)  [unwired: 1 out]
              }
              frame 114 {
                n1425 = Array To Cluster(array=w2902) -> (cluster=w2903:T14)
                n1426 = Unbundle By Name(w2903) -> ("Data[1]"=→"伺服使能":u8)  [unwired: 1 out]
              }
              frame 112 {
                n1427 = Array To Cluster(array=w2912) -> (cluster=w2913:T14)
                n1428 = Unbundle By Name(w2913) -> ("Data[1]"=w2908:u8, "Data[2]"=w2907:u8)  [unwired: 1 out]
                n1429 = To Unsigned Word Integer(number=w2908) -> (unsigned 16bit integer=w2911:u16)
                n1430 = Rotate(1:w2911, 2:8) -> (0:w2910:u16)
                n1431 = Add ("加")(x=w2910, y=w2907) -> (x+y=w2906:u16)
                n1432 = Divide(x=w2906, y=256) -> (x/y=→"Kt回":dbl)
              }
              frame 109 {
                n1433 = Array To Cluster(array=w2915) -> (cluster=w2921:T14)
                n1434 = Unbundle By Name(w2921) -> ("Data[1]"=w2919:u8, "Data[2]"=w2918:u8)  [unwired: 1 out]
                n1435 = Join Numbers(hi=w2919, lo=w2918) -> ((hi.lo)=w2920:u16)
                n1436 = To Unsigned Word Integer(number=w2920) -> (unsigned 16bit integer=w2917:u16)
                n1437 = Divide(x=w2917, y=u16 8) -> (x/y=→"电压限制_回":dbl)
              }
              frame 101 {
                n1438 = Array To Cluster(array=w2923) -> (cluster=w2924:T14)
                n1439 = Unbundle By Name(w2924) -> ("Data[1]"=w2926:u8, "Data[2]"=w2927:u8)  [unwired: 1 out]
                n1440 = Join Numbers(hi=w2926, lo=w2927) -> ((hi.lo)=w2925:u16)
                n1441 = To Unsigned Word Integer(number=w2925) -> (unsigned 16bit integer=→"T2":u16)
              }
              frame 97 {
                n1442 = Array To Cluster(array=w2929) -> (cluster=w2930:T14)
                n1443 = Unbundle By Name(w2930) -> ("Data[1]"=w2932:u8, "Data[2]"=w2933:u8)  [unwired: 1 out]
                n1444 = Join Numbers(hi=w2932, lo=w2933) -> ((hi.lo)=w2931:u16)
                n1445 = To Unsigned Word Integer(number=w2931) -> (unsigned 16bit integer=→"W2":u16)
              }
              frame 94 {
                n1446 = Array To Cluster(array=w2935) -> (cluster=w2936:cluster{"Data[0]":u8, "Data[1]":u8})
                n1447 = Unbundle By Name(w2936) -> ("Data[1]"=→"极对数_回":u8)  [unwired: 1 out]
              }
              frame 95 {
                n1448 = Array To Cluster(array=w2938) -> (cluster=w2942:T14)
                n1449 = Unbundle By Name(w2942) -> ("Data[1]"=w2940:u8, "Data[2]"=w2939:u8)  [unwired: 1 out]
                n1450 = Join Numbers(hi=w2940, lo=w2939) -> ((hi.lo)=w2941:u16)
                n1451 = To Unsigned Word Integer(number=w2941) -> (unsigned 16bit integer=→"编码器线数_回":u16)
              }
            }
            n1452 = case shown="真" w2382 {
              tunnel: w2381 -> [_ w2392]
              tunnel: w2380 -> [_ w2390]
              frame False {
              }
              frame True {
                n1453 = Array Size(array=w2390) -> (size(s)=w2391:i32)
                n1454 = Open/Create/Replace File(file path (use dialog)=w2392, operation (0:open)=T11."open or create") -> (refnum out=w2400:refnum<file>, error out=w2389:errorcluster)  [unwired: 4 in, 1 out]
                n1455 = for {
                  N: w2391 -> [_]
                  shift-right: [w2408] -> w2397
                  shift-left: "" -> [w2405]
                  tunnel: w2390 -> [w2403]
                  i -> [w2404]
                  # "浮点文本存储"
                  # "2-14"
                  n1456 = Index Array(array=w2403, index=w2404) -> (element=w2402:dbl)
                  n1457 = Number To Fractional String(number=w2402) -> (F-format string=w2407:string)  [unwired: 3 in]
                  n1458 = Concatenate Strings(w2405, w2407, "\t") -> (w2408:string)
                }
                n1459 = Set File Position(refnum=w2400, from (0:start)=u16 1, error in=w2389) -> (refnum out=w2399:refnum<file>, error out=w2388:errorcluster)  [unwired: 1 in]
                n1460 = Concatenate Strings(w2397, "\r") -> (w2395:string)
                n1461 = Write to Text File(file (use dialog)=w2399, text=w2395, error in=w2388) -> (refnum out=w2398:refnum<file>, error out=w2387:errorcluster)  [unwired: 1 in, 1 out]
                n1462 = Close File(refnum=w2398, error in=w2387) -> (error out=w2386:errorcluster)  [unwired: 1 out]
                n1463 = call <vilib>:"Clear Errors.vi"("error in (no error)"=w2386) -> ()  [unwired: 6 in, 1 out]
              }
            }
          }
        }
      }
      frame True {
      }
    }
  }
  n1464 = while "接收线程" {
    tunnel: w9 -> [w2946]
    shift-right: [w2944] -> _
    shift-left: u32 0 ("RecvCnt") -> [w2945]
    stop <- "RcvEnable" continue-if-true
    n1465 = local read "Open"() -> (w2947:bool)
    n1466 = case shown="真" w2947 {
      tunnel: w2946 -> [_ w2954]
      tunnel: w2945 -> [w2949 w2953]
      tunnel: [w2949 w2952] -> w2944
      frame False {
        # "CAN未打开，延时50ms"
        n1467 = Wait (ms)(milliseconds to wait=u32 50 ("等待时间（毫秒）")) -> ()  [unwired: 1 out]
      }
      frame True {
        n1468 = local read "DevType"() -> (w2958:T5)
        n1469 = local read "Channel"() -> (w2951:T4)
        n1470 = call "VCI_Receive.vi"("CANIndex"=w2951, "DevIndex"=u32 0, "DevType"=w2958) -> ("Recieve"=w2955:T6[])  [unwired: 3 in, 5 out]
        n1471 = Empty Array?(array=w2955) -> (empty?=w2956:bool)
        n1472 = case shown="假" w2956 {
          tunnel: w2954 -> [w2965 _]
          tunnel: w2955 -> [w2960 _]
          tunnel: [w2964 _] -> _
          tunnel: w2953 -> [w2962 w2977]
          tunnel: [w2961 w2977] -> w2952
          tunnel: w2951 -> [w2963 _]
          frame False {
            n1473 = Array Size(array=w2960) -> (size(s)=w2959:i32)
            n1474 = for {
              N: w2959 -> [_]
              tunnel: w2965 -> [w2976]
              tunnel: [w2974] -> w2964 mode=indexing
              tunnel: w2960 -> [w2969]
              tunnel: w2963 -> [w2973]
              shift-right: [w2970] -> w2961
              shift-left: w2962 -> [w2971]
              i -> [w2967]
              n1475 = Array Subset(array=w2969, index=w2967, length=1) -> (w2968:T6[])
              n1476 = Increment(x=w2971) -> (x+1=w2970:u32)
              n1477 = call "Demo_MakeDispBuff.vi"("Channel"=w2973, "Type"=enum16{"接收", "发送"}."接收", "OBJs"=w2968) -> ("Buffer"=w2975:T7)
              n1478 = Enqueue Element(queue=w2976, element=w2975) -> (error out=w2974:errorcluster)  [unwired: 1 in, 3 out]
            }
            "RecvCnt" <- w2961
          }
          frame True {
          }
        }
      }
    }
  }
  n1479 = control-ref of="本应用程序"() -> (w6:refnum<vi>)
  n1480 = invoke class="VI" method="FP.Close"(error in=w4) -> (error out=w3:errorcluster)  [unwired: 2 in, 2 out]
  n1481 = property class="App"(reference=w6) -> ("App.Kind"=w5:T16)  [unwired: 1 in, 2 out]
  n1482 = case shown="\"Development System\"" w5 {
    tunnel: w3 -> [_ _]
    frame "invalid app kind", Default {
      n1483 = Quit LabVIEW() -> ()  [unwired: 1 out]
    }
    frame "Development System" {
    }
  }
